vi "7Decembre2016.vi"() -> ()   [LabVIEW 2014]
panel:
  out "Pattern BAB":string[](array[string])
  out "Pattern ABA":string[](array[string])
  out "SLS Support":i16
  out "ATS Support":i16
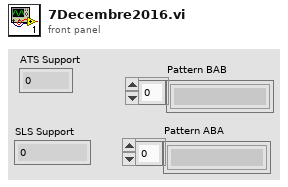
[diagram p1: front panel]
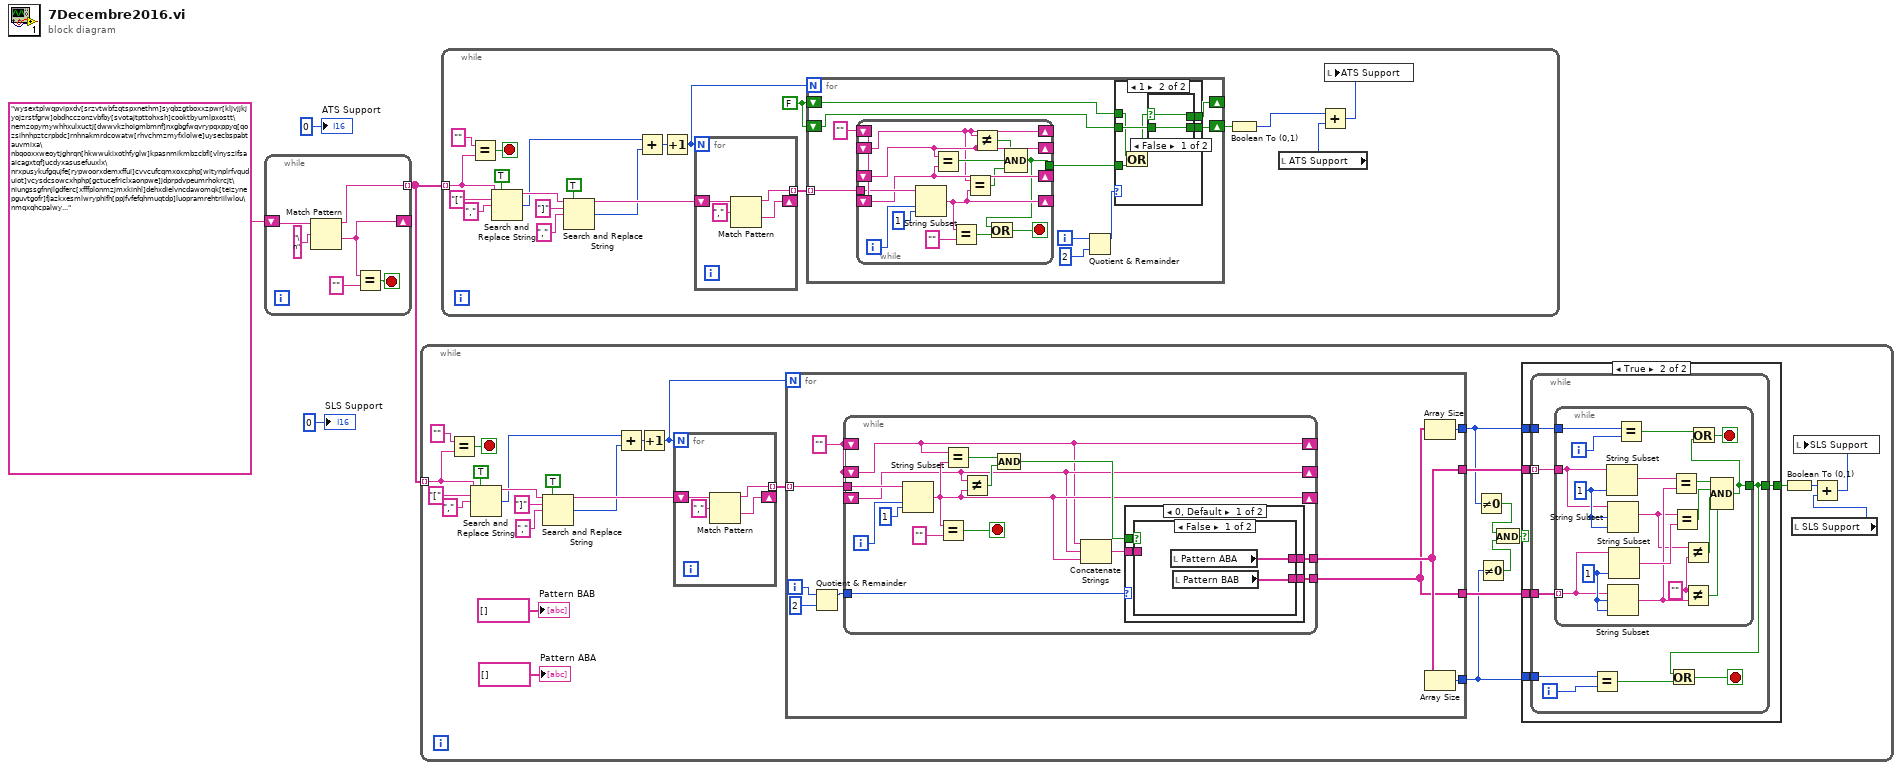
[diagram p0: block diagram]
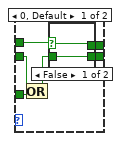
[diagram p2: hidden frame]
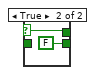
[diagram p3: hidden frame]
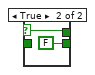
[diagram p4: hidden frame]
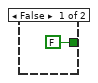
[diagram p5: hidden frame]
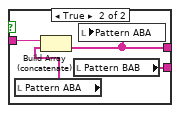
[diagram p6: hidden frame]
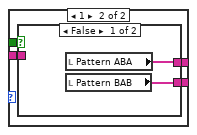
[diagram p7: hidden frame]
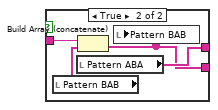
[diagram p8: hidden frame]
diagram:
  n1 = while {
    shift-right: [w7] -> _
    shift-left: "wysextplwqpvipxdv[srzvtwbfzqtspxnethm]syqbzgtboxxzpwr[kljvjjkjyojzrstfgrw]obdhcczonzvbfby[svotajtpttohxsh]cooktbyumlpxostt\nemzopymywhhxulxuctj[dwwvkzhoigmbmnf]nxgbgfwqvrypqxppyq[qozsihnhpztcrpbdc]rnhnakmrdcowatw[rhvchmzmyfxlolwe]uysecbspabtauvmixa\nbqooxxweoytjghrqn[hkwwukixothfyglw]kpasnmikmbzcbfi[vlnyszifsaaicagxtqf]ucdyxasusefuuxlx\nrxpusykufgqujfe[rypwoorxdemxffui]cvvcufcqmxoxcphp[witynplrfvquduiot]vcysdcsowcxhphp[gctucefriclxaonpwe]jdprpdvpeumrhokrcjt\niungssgfnnjlgdferc[xfffplonmzjmxkinhl]dehxdielvncdawomqk[teizynepguvtgofr]fjazkxesmlwryphifh[ppjfvfefqhmuqtdp]luopramrehtriilwlou\nmqxqhcpalwycdxw[fkwhjscfmgywhtvdb]khadwvhkxygtxqx\nihekzgbwpjxgbau[eqpvqxncntbtsqn]mbtbcujdkbrhxdu\nizikobnovmjzngo[ombcpcvshnedtndu]lnnmdkuapgnxpgyxcmg[bgnxdzmiolfvvaizu]tcvnrfufuvhgmlxcm\nyhrowrreplrrsbupeor[nchtznfzbzwnogh]rynudxihckzattbz[dshxeaqusdlhydtm]rvqzuffgqtysfzxp\nunfjgussbjxzlhopoqg[ppdnqkiuooukdmbqlo]flfiieiitmettblfln\nhgtbgxarmgbxqrhghxb[hflfvoetxfisqsj]syhkugztqkywetyhad[fmptjuaqittvvyooda]cjkxbnylglnlfleelzu\nnpxhwtitqnddkwg[gmzggwnvygsroeaadtc]gudnfyefqbbgyspdxjw[ilthbdqubqnveowv]xitfldhfjyjsomygjg[knmrlvoiqyytigytlum]dlfpsnyzmhkmeevfwsf\nwjzwftiuixvwyzmgoe[jbfghrqhyywwhlu]wcijbojvlgjjdtowzpv[lgfvxfdusgxddsppbxb]pagicuiuerzeydww[wlpjklgzyilrifonz]gdicckmxibtwwoesaxf\neilrieezaciolhnhrc[hcisnfomqiiaculxfv]bfyxxhgrakqogthzft\nxijomgpzpilomlpy[sfgwaovcybyhoogrxsv]ufncwrahejwlhyvz\nnojlhdpfkjbhahgqo[lqrkjabuijutlcbq]caszlkvkofxjyqzsttc[isqicyomykudneq]izuzehgtmwnnvfrlrja\nqwfvuzrogqzvnhyqdv[qhnjhafmrtghosbmskc]msmwswtgzlpmtmzne[kovzhefjqtqadhj]myqisirynftmtzvxvvz\nfrfongnaecavmrhj[uuptwvcqozxnglsd]kwpovfwuhmqjkog[phtrgysxaltvbohmv]abhuahonmbhsmfglltm\nwdqcwcbtpexduecepe[zwrcpctlwglgfpappb]zdadimzdcpxhxwde[yquulvwgyyzwcfsvkdt]thgziwclyxxfyjpbpc[ypkjfrfkxlkavboh]hxylcecamgezuoljh\nyqxkafpkuuxfafe[zehlwtvpprtiqbl]qswqigaeaneovxm[bqoieihtxarwyrqegb]yzdopgmqklqaizxjm[jhrsftklywefyevvha]xuvydwcntczjvuduj\njudhawjtmpsxfocai[qghshlgvbitxevt]xehceioknrewezihnb[jvrzemakemtgmqiqmvj]wewpjflvqmottqx\nuhokpvanmvdobqitn[eosarcmqnukoczgz]rmoowtgbbyimkptlxdu[rqhewmnpypqpyosgehz]nqdwglwscsizxey\nsbnojmynueuyyutr[oonxqrbbjxwvwafad]krqlneuehyrghmkrq[khsckkfwowubtglegu]xweufrmlufamzbcedk\nnmgjmbwyrvcbthw[ogtvotifzugvvrsfe]jucqbvfqclkuxzumoed\nuaokpcytcrfpitfursj[lweyfahryjfprulw]dsdutsxdtugaced\nahshwqihivxlgsj[ldnmuwbrmoxtypqluyz]intafryfavcnotgxu[xjggdyvoarfajgp]zhfgnytzjhuyheqdy[yeynlfshsyrhjxrzguu]onvyhjfwooikmmqzwgc\ndjkgxfnfojgjpxec[ngwqajfbywoxlbm]oqdqigzeqadgqjt[tvojayieruftbjokeeq]gxwtruomnhorqqrpzt[bxppvnbiwhkhdka]rhpffqekyrcgwqmoi\naasbwiocfkaahrjwerr[dvlemehlhfzxnzymqn]okxibfrlswfvmreuf\nrwcjoknjvyufkrp[hsqrwhdlwrtlthp]ijezyezjdrhzgltliq\nazawpddzkqbosmltyxt[zoaaqnowmmwkmfkq]lgusvzwnimvgagupkt[scbjhqdftzssbvnvff]coiaslgcrwvyioxx[jouvwdiwvbsembzf]popmlnhjkoaeahcny\nsnucfdhspcbcsgjnmcc[qbicureolmbzhsy]cuabqhzbcbkezsumkq[cnggwqizurflommitua]ajtxxkqwqynnwroi\nbsxzwpiauwlqelesq[uqfdggoirtlucvedpl]asacxftfqfswiapmj[nqohanbbzodfgkxihtt]lhshhkgjvjkumja\nbeewgulkwnmwxenstrz[vybrrqhcdpkhfnshccv]xdfvqzdslwosulzatc[kuknmynmjntvtyduwlh]trfvychdobyghnrxrfy\noxrwmqpvxntdkohmxb[wugyubwxumwnxlk]jidpzvtbomuymyf\npqzbwlnmvtytsfre[pmtmcnxkylmqaeb]alfdaofnqpohulpmfoj\nqopdwichdepaubxxeu[ifjozmlqttahyugyt]mfmlwxifscsnuom[kiyjlqqxunsxfmht]icofrxpdpsktwiifyb[hetijegmockkyjhhc]aarioqngqmdpkti\nklumchkwczxuuekdb[nlalmjunselydybqxdj]alagfcxocldfyzdnzd[abfnqrgrxbscagj]cohrecgrcaxljkz\ndjydzyiyydcneoubp[gorqzujuwkjsqhelfrp]pvtvbhztirfzmwcopfv[wfjumxbfvvgvzltlcf]ergdkkakrtfzcxmqcc[vwnkrxhayzbvbauvn]yjoqveipzibbmjq\nqbdruhoywfjhaljfkoy[tznfejprrnzrrewdx]jziputgqfcqtbhvhlnw[ikahxtlheeunzrdq]tmoanjmpioumvpcu[tnmcvxkewovprxgzd]trnmnhdvtsisiujqjk\nllojixxpxtvcwxaxp[rurmhymwuztchngs]weaefxdkjmofeydvfy[hmbracjdcwxfeva]jkiybiomykfexjlyg[pgrlrqgoxqqtoio]rdynpcndtqarmkagbw\nkislmybuoblnpsc[dvsrnwlsvxxmzuu]jakczftcvijbavhjgb[osdyplcgliragfnpezx]kihkywmwgbkjtgxn[tdsgdadcvcaxfrbur]lzyjmrjqztybfdmm\norfngwdzlrucbkbqd[ibvlkwlnnzwkhnoad]brstantuaxwkibofh\nvuumejklanuomqqdbva[mwjzrpargsphzkkhaaz]lkkewmbrvuczyyu[ebpoqgoifelelzzhd]biflvclnnimuojihdmn[llrnjdgzagktjrys]edtbmzmcbthpixhwwyz\nftaciyszakisxhzjhbo[khfshezpopvjaki]pdnnsqmgpgatvubllrr[ovjrouomglbpgvtya]ifwcvhascqptbvbums[cfpimraygtnuimiup]zeykmilehidtlstjux\nnzgbxxiimmzsvhe[ixypsgextxvdckbjelq]jpklrvkhgzprfrsv\nmpdlsziccgzmvorvm[vhxbfkwfwbxqbvxp]zbsxgodzhgmrhrprpu[pvawdsvqybgdncgxido]zuhyfbmmhzegohu\nrdkteyoeleyhxdlfa[nrrzftpiqatsnnnsd]qwelhxwbpuwjmrjxmgq\nvpdhtcgjpkrqmrt[gozqldncggxpvou]zedtarenbxskusqk[mwpmzpwraryuqqmdhrd]eoculislafmbqzy[okpddsvrtyrkbjtihhb]dvuadhnaxkfewhnksl\nivjfulhqfbdqiprzbbe[ezhkhqxcviwxbwmlnbb]ttekmmdrphuteslzwcj[iocuduwexawydww]qmrfnnedqtqezclpuq\ntksplumjkpsjjorux[dpffmbayilzuszc]rsiowigabmredkfv[aurieaasmsrxufpo]lbwvhcrjfgomkff\nuwuobjzxkgeugrivc[biktdwykzondbwiko]nnrtnqzhdhdwzkau\ncjjawanjvbxvmvdmtu[kubvvkuoynaawzowphv]ssijoohfemyhrde\nqlykdpnioshrexuw[tjwoswemjxylnqupgv]ymovhecbliuuzhjwu[ghxibaaourtzzogrynv]hmlndovkousrtbomlnz[nzkdpmqrqovnvskh]vdvntntzrqrhvcaxdov\ntdhrefyrccgkdquxz[jqeprpsvvkmmldlwyq]lwhnimtgegsziejeh[gyefzqbmfnhzgtq]fmbcvbjtsriuicde[sbkkbqwzlluccpa]nwxmuolcbhtwcllmz\ncakfzlwlaxgrzjpgck[toihlzbehdzesbt]azrsizelgzczqxwejb[ypecquckfavmixeyjgr]njiyddhuwlwogbnpt\njadaohixgxzjcopk[wopcnehanaabtklxnez]jgvumwvmixxxwaolxb[lrhmslkbmylyvlkx]tatmsbtlbcutcydlrf\ngelrpwfiyiszejt[skpclwjhzgwvfbbd]ibwzelwwhvudmvoe[gpdveubkzkkxvtjn]khmkjslnkdlmefcx[fcwhuyiyvnjgfcva]qjcfuqxwmkyvvzuj\npbejigkioxtdjjzbl[uihultqxejdyegacm]fitsnuitopdzrxskz[shbzwyodcotpvoixoz]qrhuyetkmnnljfqt\nyohbaryhrhuobkf[fmfsylvacrgvpnlqdb]iucbpagpbziaqae[lfcjrlbgxiytord]mhjlzecyrqcpbxsaq\nvguohtnahunrvrfv[lwbganvrrgnasnkqjz]yuoncrmethwiglfiy\npljibizefgbrfauieem[yadmbpkftrtwjrize]fuzpxdpomsdxfocc[lvoahklovaxtucrpwhj]newpgoizivpqkpo[uloztzclhwixtcjhyon]qyzzqoyirejavchy\nplinqqpqghkeuipqppp[rndecheohrsftgvku]ogsyvyxuetmdomwdmx[lumcfskwppjacuddm]uptsydogwyqaupdft\newvtreckmjqvkvwgtz[leisttvtmrxnzjv]bfzzponjsjmepqjfs[knbonuuuhvtvteiov]vaejlijsnrpqppo[hvwwdxernqcxtxe]ssznbkhfmchmjjiahkk\nrrofpphpfkeeqlxcev[ierkxtuduxxxbilmg]vmipzdomogxwiazla\nuqmllifxqxwcskoj[lwrjkmxgwxwvkqrsajx]wpbkbsohlaeskzbv[boyvlwxpqpppcknocv]pgsvgtugmxmoexrvpkk\nzupunwchccxqggie[sdcdhzciymhppyaaaib]izbizcvzvbcnofmqt[lvvxmcmydxruvudsar]gnspfiadqokusllygyw[wbcpnuppeugrqobtnu]mcvfhylypayxquurcv\nngscsmmvttxjxoaniu[wsfnnfnkwmjxjql]ijtqswaevexzcmgime\nhkmykmrremccqxvfdps[izfaeewfadfhuwwd]yffzgiqtmayebphb\nznzxjrdnxhfydrhr[kwafvmygvlylite]hmskvvpqyoblrygj\ngkxzweijinwxyajq[jzljdfxlossksqa]octzjmrvxkumtpn[jypbqguwpybykguwn]ngriygtjydfznsf[cpwtojpifkhwtfknjsg]zahxvqxjtoutvvsphh\nkmvndjahzayidho[fitbtgfncjvmbyrbvnf]fodwrbklqhxpsrqwh[ccwvgmocbtbqvwzu]uuidhylekzxzvmce[qbhkjfhnczasecv]ctsfirxwjfvrmayoeb\noktwbkikybfwojcweal[pnhqkawxmfxggabhgpa]kdjghdalrpgsdhqj[bxjcqdytenfjirvb]odnhihekqyskaoedyor[pqsixozypkjdnnntbng]negjtmkqfykrjgewt\nhriyrcurqmacydyay[gfblxaovvngyesfa]tmftedgxujvmjze[knivpbneiuxdsowcxdt]zzncnfcouzoppog\nedabqgdgbyjqkzjvzhr[rdejmmymhnvfrqvf]zknrxaqjohlncvwc[lcpuoqnkvwgjycfm]ohuebodqzydltckrsb\nrxcyawcfxcjtdshxg[zvggbsrobekoxidyx]zdpvqowndwgdubbhst\nqngajrgvzuafovkr[kracjvrryquumqerjev]mqddkdpqmfgexahczm[psmbzonkrrtlqdpgqci]obiynfssuwhprevmzm\ndihkldbnjicztjfrvga[qtlevmacqkefjomc]opjaojctoraohocxaca[ojldoulpocpcpexnyx]qnouppkcuggjmod[oeiywfzmbjrhtxz]mvhoarchbrpndgwhxga\nqyncschbsnqwgvfu[cscsfdcfbfqiwgwqi]pqzbontuospgycwzqn\nlwvovybfksidtajq[vrtqmrxzouplnjogzk]gailtfjtszlxzwhbs[bgqzyhgudphwgufmg]levofhjnxjqhkcy[wbffnapyutukiavenm]olkwwlrbbobqudwvnur\nyeqiptxuczuxzeatp[upzutosphyfhuho]jehejxjvfpqeifogn[odhltqvdcwwmshl]coezfdamogigspon[syppfhysfwfkisltwr]ihkaelrbcelykby\nnmciqyaovpdwzldwt[zoaowvxkrpfuwnyepcb]yhqlmmrxxvguuajawb[rmilfmqzokaeabc]yhmswnsiyrepbudi\npifzooabiqmuicfqi[tvaqijdwxsbamxzg]zncutzbfmraagej\njpgkrbovswsjnbcj[bjybzimnzszdkqj]mvwmgdithrxecpselt[kghbhnctqnhhxxhdro]drttsuyvtuuygdtfaf[zohajxyfyjnqrigq]gadarjzfafqxsjxk\nwivyofwdmipecdxuqu[trccnlbsvfbagstm]xajuejldffxzxfygsg\nqsuxdmtfgpmlgkh[gisuuzaglpmbmydtt]qzyfvzryxepjmnr[mgsjrbmtxxzkadomelm]fqzjahepxspwkwpwd\npncauthrouncvjkrik[cyiovjnoesdgpeyjpvd]ajhonypsbifeghxi[wmudcxwbewumjbegnh]qetzbstgmzfruzxqln\nqmkcddrhexvtylukq[nwrryzbnjnhvvgm]edxlyprwzzhgfmhz\niuonniejtavofqdqsln[ynjrsfsqrdsgydhpdvh]xvqtjledtcgkjkealws\nfhbxdtddlvkjrmjyae[nwwjmjvxtabdwdezfdy]iwnsmstiulolahbxka[lqrxlwifzndbeid]jilfjomwrbjeniwybv\niptzrdexpfzabqcqkm[kvaxgarrbrobtmu]fqaedifschjkoepn[widcirixuswhcvcqywp]kpkxphryiwwnkmb\nzbeoanntetxhvigve[fhwvhghpujcldib]ncrcyvevibooqesy[ougjirkquasabeqad]ydufeicmimcwgtbg\njaocnzcwgxknexaf[cqykwbyvxtcwnurw]udxjnumyhelfogapi\nsduqgjoijyfrcnfencj[uxuiwklsiuqwjjrzcfn]epnvqcjspwopyffl[mwghrhtfclodjan]ghamugnhrrzjwmnc\nwoygyvtrlmjzaeteuj[vvvfohavzuuzyzgu]xjjcxhosambmkixiie[lqholbwbktlvdljmapw]diufpkdnjmjnmyc[ehjexwagbmezmpj]czhwzecixzxfykaiafj\nnkijgkhyilzqvtgj[llydwhyhnhpcracxxd]zgtsspcwpyujndbxvp\nnawnrsgxqpctinyek[ieguugfkwujnymij]rfmqypeekkdsttdw[rfuanabgfjgctueaaqo]vranbomhrynvjyywmh[zjncmschlfmkvhd]gfeoftxsawcgrzvrlx\njgazasxbickiiiz[duuskjowanfmieegl]cwgdwtrzpbfemqitbhb\nlahkgoaoeofjlocsei[bwxyguvgmenwnpwlp]jigdlgdjptkimoyipa[zlcyjbqohvmlxgxp]bmovqedgchicusqzq\njhkxinkbwhpddvjzgod[fypyyhptvewejlbwdmx]teagznqhjydanxxi[wkppnjsyzhwshtpo]piaqxcwqolwklwzsfkg\nsjedigezzdkqlxlcnr[xanehtpradlngiob]uonmjrieoycpthh[wnsqwfubwxkqhlflzv]smrebfwpnhskzlknva[pylbyttmhyggonlk]dwqkzjmatybpmgeb\nktfcuvnwueamlwvgwmq[czcgevditrtvddgfh]djmmelqewdnzrlqliz[fkpieaipgyxnkmjp]rdpkfzvqpfpvczv\ntixjemagwmynkihelk[bnwfmkugsnivgdmvskc]nlasqrjqrlorszi[kbatouwdhejxchpdhd]etmbkytyrpnrpgqvel[xahfkfjmsqjycaq]mispsimhcckrhqvek\nabudxncgozbrbnx[fllpjgocynbuyawgs]hiphrvpugpfnnppn[jhmlgjsufflkdgw]ldmdclrkorzjtbjqcrn\naljahmvdrraiavzv[tevjntkppnjqwovvuuh]ozmgagxzixxyzuy[zgefziawisowuyqra]nrqmsbwgqbfrxqvzu[zvzglmnjmjpmditiodb]odzbozesvocemfyis\nzgdukwtswaosbrossf[ugdnezayjnbjuhpeh]knkvomcsgfptssifni[votpmaaohcyofgdz]skbvfugaaxutcmrmsc\nywiphurgqcvybiakgok[cscyksufsduegggw]rtvvvokrvwmwsvmk[oqvdxhoqfsfdwwm]sbzajtnbxzkyiwrj\nnxrvrsbjsrysysvftoo[qowwnvlezexjyynm]nknzluizyzjpbzpevb[adkqviapkjbmknchtb]xsgtthuifmsqidyh\nejrplkjjbnjjouesaph[bdtybzkfyictcjuagr]ivtcttyunertnzgmpqv[roikukeznmtkqomqbk]lsxzsjrnsrdlxevj\nqgcebktqtyjjwsav[naozjsnqufkkgkp]evimphuulhzflub[weanrdvlsmmypnh]rojhwlyxtszxsjiuai\nzludmyuqlfpefvxcm[hejpyhwaqdndtwslan]ldtxkxxtegoqpntsnwg[olhtlkpvkdgkkxkisp]hursraavetjgloks\nrosuljoqspxeovaqr[ocjdnpuzmwioylt]txylrlsndrifxiuxuyg[jnubpcjyfzhiwul]pdtcjcrkpmzlayzcty[gasynfnouxnvrplkym]naxwpqsxlsbvyuavty\noxbyqbqmpckkdpfjtr[ggnmfcjtyfspqrqkg]tzapjijawrabozckadp[varichgjrivmseddxv]admqmnzxzqcbapdquwd\njvhvqxvhqfxnjzmv[hwfwxvwhxorzqizc]rpjpwggqxqkaznkuqn\nyrsucbqcfaukancrr[nabtowgijsnzryuvbiv]sfpffzxrftnrkjx[qfyfsbkyhetcedf]xdykjbymrqgheanxx[oxchcwrkbqvvfeyi]bztjlknshikocxztjm\niniqqqqprdeznwhr[arooglolfjgprfrbhbm]sczcmpftuhbaagwgedq[yutgzaqyxntjxoglmb]vswbhlspwfulowkif\nbjcjrdzwhmssgoinrcj[jobrpyapaxkasve]hzacshssrxkdtrlqhr[yygotqrmvhiqjrja]ljwfwudymzkpczysknf\nlrnqnaxtavkhwfebb[vwyqnqkveujnlzv]coizhrfmviizxgz[zklqinvtnwtajyjx]nxvpznyebozrosfgh\nccjjszgrbozbpopagns[abiuzirqfzactus]eemrbqrkhhppvan\nxeaifcibybamzzzic[ymvsqllvremyfify]ftgmrkhzswdpbmukcdv[fbyevcnnwtnodgxy]slfjznnldyuvair\najmeryqwfhniqenmi[bdzlgljpkkgsvpjcy]hqzxecqxmneterlqizz[pzrbbprbhujzpcxhjmh]lvrckyomhvidbiapikk[cyyapugbrwlubpmn]toodggarcneobyz\nlehpdvqjccdfpzpo[ssunfejvfxwzlzqy]dvhwfrwiipveqpb\nijmthhifxtkoubt[jcgoxkntpnxkmdp]rzsfekfmamzddgm[szvzrwthulqzcorhnk]lmgsxsjjcagkaysalnj\nqmfgzmmoylbruqxoh[uoyinkzbglorxud]frtffuhkchkrwbxfx[urlwigeirzobvhir]pqrqujuwxueommaj\ntzjhaiqumjufkzcvphi[lhfohqxxuoqybomckm]qjhpjkjljzekboyc[gvzfehzyrfaarfklybg]fhurcpaukztwesz[lhvnhfgpmunjukye]mdzcvgeehmchcqe\ncbyyjbdwzgdhveyw[ockkdpwglixvbom]ozezplbkvaulagw[vmzfmqxplwaqjrf]upytqbnzjrclzfvti[hztxfkqwcuypqyhsfa]sfwcfhrnccesyncbg\nzaclpaavkxbpjxse[dmuzswkobdcfmrejhaj]eqdwvpiphijpwrvg\nyvectfptgdasqxi[rmpaospaiqhwpjwdru]ollajqbxmfnqmqrdce[jqixwgznolbepskpm]pmyfsrnbdcqdrhplko[pzblovbmbnbwjzsxrk]hgwpjhgshxoozdu\ngpnplfnpnmdlhehgazx[gkgcsjdcfnxytzp]wamlpixcrqvbtseb[ijaxccauotewzkgu]usgmgqmezufmgqjslbu\njgtqghpjnbjkmajymfw[isxpkhlvtuyqpscvm]czbrsyeqmjnksov\nfjsepwfaxbbsdxlcz[efiljmecvcsybpj]fsvcvvewoepnvqz\nnxzdtgomsakdhwefrn[cobjsrlxnkxvmhk]wkfnuypvsigzcnswufj[ttmtjfkbnhmmdebtr]ffumzvnvgitjccgz[offnegtizuxhpqmic]lbhljegbjmldqbzryis\ngnnsvlcqoatssjuijb[eaodophfeufuvdodj]jplhbuvzqfgvrqbuy[ezxxqanlgnxdkohew]vsukbzhjshwmmqdkzdh\nshfhzsmqdeibrwgyr[slyyksjeywcnuaocadr]kdwnsokrwkajgnwi[zsfujtkhknplyieg]kijuvumdqvjyjpbhl[qyrlzloooajylfrsfk]gwqdkfpitiitrednt\nzhmwbilhpywvxrza[tgnybotdqixzolvn]ptxzyjbayyevmcqua[hcmgjpycosutmqbtkf]tboiprpyhwgjceu\nejuvrirctrlirihunm[nfjigabdmqnkfoauuyg]rfwcumqndfgotyx\ncxkwlruaswigkrtxxch[fjsovwltjonhegm]zkfawxnzxlkaqawq[rgfftbipxlmelfnpf]qhhslyyiluvowxz[bgxutaxmhxyxxdob]hzthuaqpiyeomlgqqcn\nqyzwezoszvwrwiilglw[opryawlpulfkpkmuave]taxeqyunnihulfp[vzxzosekvamoofva]bbtonpohbgdwfmt[xwzkmwrwruatcdqrj]enrapbeqoxrufgp\nlowqonzaekybouni[uehkpbaxwfixuwlj]ionorsihznoszwzyq[cnatlobscugfpvpbw]lnsmgieepzvmhvbz[lsjebmtctttclkxqok]jwevnfmcrtmgjyniiuf\nltxumfyzdinfqrlf[jyiwmlpqkbnbgmu]bnicegkghtwivvyozea[qhgoiugrookfmdsln]fpokyqsoknuahpmutnm[smzqellevlxgdbbet]vsadiuyglyyuccgkrz\nfvhanaukvcjdkhsydnz[pbjsoundyybhvaqglj]esjjvkdvjmgmlox\nhcckhzdfmmvnsmuzjg[uuajvdzksgilxpjmnv]opbmjvfljnqzxkql[pgdelzddxqrfdoqnit]hqrrfnwrokufpybg\novtjlczqesucgox[kiqphngcbakoelqncyi]jhrwrpwdjxbhnqp[kqvqdyokyuxulxidc]qumskxudarjyagegy\nmxrxpfkynragapzrmdv[rdhsbrxgeywqbqh]rpoerdiwdisciarhl\nejbdfeqrdsrijztlibc[beglofnxveiorftulay]jslqibpnunabgqmi\nuplsbqledimexhzwnkk[sfreaeitecravsu]exfxqlrumxaeasi\ngicahlhkuxbhppe[cypyeqpzkrggfqrielv]pkuwwtbezndgtqhbz[ojnnxanlkamvmpqfj]eozgnkxtbtyecuhs\njtzwiyeueztuiwysyv[awibgssyyssrnuxrvuw]mmyvqfgaaraahzzen[rhscfvdrvagricw]qsqbnurcszgekmp\ndxkeveuauhblqnq[oksqvawybtejxmdw]jrbwmyxdggncxitwcms[fvhnmupxnynxmprs]odbifiqqxskxaqn[xwdwagplcltcepjmtf]zsfevibkmzwtzoq\nkflcnlkdujmtiug[rwydvjaazfgmfcn]qolbbuxzxhoizfqcwn[tprjkbylcrlvmbggae]pjwhgcmgxzhxbxdceme\ndonbjfkqtygixfpaa[lhfcyuzcmsgixjbr]njvgmbwgzimrtpdmvf[eonodblqfpgtmex]rkakjzfmuyeajvhs[lmgtvenasnqbyby]jdbxoeqnwoednoncq\nlaiyueskjnlltkwm[lzrgjwrjchpmnais]pqltpskalrwtmtagvm[luctnpiuqvulmtmw]awlqbuutunlbpusn[hdetxhrtzhkyfktmfn]qpmezabxzrtquidbjc\nhritvdzjxipitctgoex[jtbjcyaysbefjme]ebbcyqglydfhqjfa[uwuwqhwanfydpxqk]enevryjyzduawrfc\naxxprqpxpifqnwte[qwkkhbywyixngun]ufwcbmerbqiblbdmn[mguzyerbfhpqnybh]gscgmmckgfxvvwgxxm[gfjzckcxdowpwmhmg]hjblyfatzhxjyvlccb\nqzzkrqfnnzvgfmrpjr[sktcrqxcctcduir]vmhsrsedrxpnrugm\nmpxgzowtjabzwfcbeg[olgfqepvinejmstbrj]fnqxcfzuxojvkscyk[pxbyuusrrbjwrygkxm]wiojjquwvhineivnkys\nvqcisychxuswbqlzdkj[jetvpggxtqqguuh]tyllnzfyfphoudijzj[xlnznxybxscqjktjn]oysyrlqascsqbclsb[rzhxpwwrjwakoldm]mrwzibdjlhsdsbew\nrttdskfweqmkjolrgsd[gmdwcimmgetwiprem]wkyklvpjyhpzvmsh[zftyxsrvhnioomw]mrvoyvyyrlguwedz[xyrajtcatyabfqigup]srjmohoxwdybksfv\nxzeexlrzdznmhbph[vobtfjuyowqppxw]mjxwhgwveozusndvi[jthhtubbkbmdiepfh]gtedeqwesiwzlrfny[tppxuofhnwwkbkysg]aygwlnvczaarhfgkw\nzxirxtzlqkptwqd[vwdzostlmrbjclfj]aluxqfcdbjwbeerhr[nsjcafnammlxjafrzaa]kipaqywrtrpkbcdtnyi\nvovbpdgnfhmeuadh[bcgvleartfaspvvjjz]ajyzrbirtimuifvs[lykguucpvkxuupcbims]qplsipqneiycefb\nalqzdecagmvodcigcd[atmngaijkfehfbc]cprsiaclouvtbpaab[lfrxlrzuuooqdtfirbj]olcjwtrkndcvykp[lelvgglysdxycvk]uyakjndqzxtzmxs\nsyngsortxjqcdwcz[qkiseyvolwhibxdg]ucuxqdozkfgaxqwovk[eqeessuwvcayhpc]wkhzcbkxgakgxnmho\nbhtxesznfkwqbodb[ptpuhbdsvbcjpmnsl]oohvgktjsjwxqgyxov\nudnbbnkojrdevgujkg[cramyjeuckywtuw]qtldussgogyblkm[yuwacyafnikvgbibmwn]xvsgxmywenrmhdctxg\nuzqtkzkmmeuttwyklv[rgnrxkbavqabukxvnp]whhgpmwocfmplba\nkvbjvjxyqiqitikvm[vkzunkivwcpvxng]totvodotoqiqokouz[luzygityrnpuiih]eadddxqveeuujmvnek[nyxhwlkatungkgm]bdhobvhktlnfpjelr\ninmnseeoqimzjwzhltk[ntwlsdvvybtdoqciu]jaurhomtnyudxxmslj[wqygsctddywlbxg]apsdlaftsghmhtj\npxieimaprtbntgvm[xuvwwsinhwjjapu]taeomoijctvzyeijfr[gitzztxejfefzvepf]udobxonjlqagrkpaehc[fkqjhfjicleroxp]hxpzoklhbgtngtagcz\nlqmoxvnknpqzcgs[zktsmqcgzqjponj]wfhhzvqiqkxfwrrw[actbxtcdlogatfkprc]tvzphmtxfrptzlopv\nczdnqiwqhighizbmivy[tptpsvsahslbsovazkk]ycppvkqvuggebgxibe[qutumfpnpzjkgqyfkok]ixywxvmvliftixfie[qipgniycxomhgmwje]vnhxbcnofkcnzep\nigvdicnzsefxlgk[dzppkxdievabwyh]fvyywjzcyfcqahv\nbjzwblslduiolbezybz[flvsgshhznvzmrxo]lottitaizuksqfihn[kgsgzawzjlqjsep]ihadewtrfpsudggga[oecgswhnbhslysd]flpdpxndzacxeskzmn\nsyxfjuakhrnntipfpb[xmntswflflstndkv]lityfpfignnxsyirja\nunggjaqgvzrckyqx[llllagrmuioghea]qafuiwqpxcljhvf[tevtmuvcyqqrzvrduc]kqnaadyfxfyyzjuco\ncpjvjnocqphsagdizq[rzfbvtnodwqrqprvqh]rnlzshtjhrevjgdu[lbozqegfwoaikxbnt]cqmzymvkummuzjfx[vtknqltevighwfdnjv]djhfeemiljlvkgqkpp\nadbbbgxmiqomckxesb[dmwxvrammletdiim]eiozjsockohijbiinia[zyjjubdniurametk]ajivyylxbhvkktrzdg[byxiykqfbvpfdzdv]zborzsvqimrhyoyhevj\nfrshflyhzegyezg[xxaoqtzxuqbamukfxed]klyullmlailfvcz[boefzsdpblwpbna]dbnxivwobykcfwogv\nxxycwortiwhndrvlr[mspdwmhyqdwtctlyek]qnzfcwwvvlfsael\nfnekkofpuwhttni[mlwvhzrwfdtfnvof]gtlyjqokjymvtkiqdl[gdjobagxsuhudnoi]jgcgyusdyyocqwwtatk[rjujihcuqgdpcbdnkco]iewvagokrzdhhhskv\ndfadfbjefyinccgzt[gzoojtdlvqysetfihg]nlsriqansooflahzhoa[vlzwtzgipbaxudxg]htykxxpfmhigbdqsu[pzipnakgdfpajkbqowq]zrwedqiuobogirulfwm\nwevlduhhsouwlqxdcfc[bxcvjwespxdkulgun]hfuhwpzgdgqsujeex\nzweayhrezaoqibgvc[sosownrvumzvynfpvr]lzubqqqepwraqqdxxy[bniazltbdanpnjjjuox]tulybfbbzeiyidrv[zbebbcdzpcvegcms]jdfofmnlgwrnvann\ngkmbgzvludgmjgnrkck[ijywdgxetrginhtaa]yiokddkvhxebbuyrwoy[erhxxldeegvsebr]ujqickibpbjpizhbjw[mtzvltxionpxygo]mbcgbublhkajfdfvf\nddjzsqkoizakmeifr[sigtlzmyyrflvjowj]dyqyfvpkhdulwuj\njivforicorwbkmccpgj[oviyldmrjjzbojbs]wpztdiwcdrwttmfdw[jgylosmbgxlrogsa]htkvwsfczzoascpunqr[uemtqxhcvvphnvktio]xkghvnicljrlndjtsv\nzkzjccnvukaraob[asytykcstvxtkvermx]lqgjlittfqpyxcq[dwyrqfxmwryvxjzr]edufjnmxhzxokjgphk[ucthvgtgfpzxikmnjv]yqumujliwpjujnymcen\nbhbndmsnnbhspzjby[llodpdecwrlspsbhbhm]zqulqmxwcerescalp\nozkoqhvatxmivox[qffeloluwcgsimvcrnu]pweywrdkmtqjiflvcm\nrznstgdzevfsthcc[jpgjzgeibmumtatu]asgwjccfkwzaigwp[soegoylmysqcequdsw]pennknxcwwasonjz\nafniplpdesiwqvdioov[xfkwuijxjgtqbhqow]idmgzrcmwzmrfbsubkz[mjwyiznfpjztbfervj]cythmqghdkjcfrt[ekhpwckuwduoexycc]htaeivvotvlstvsrpj\ngecbcvpiswzjjeiriav[ivbfdesbkamvngogjb]xphdszgbcburesbfi\nuldzgctwccgqdbxrmpo[guiftcqomdqlqua]dmxluytucnlndazic[mhmdapmemlrwmvdzwkn]oqyvwmhlabcwxpzioz\nmganrfqbsckpjsnvlh[vlwmfxhxlnnpsghrhmr]eqyrkxjcwpkahqpxeqr\nwpbzefalgkbnrke[qruzjqtrkbzsvfgwz]vahtniazgsicquatrg[zzslttuxbwolldy]cuejnzjsuwgkobp[yspyowiamjpzcaqwb]vhakhmjrncjoroe\nycxznczxbzrprsiw[oggkqxyiyvsrmxck]asjjivqayantzzfysr\newbllymppqrdnaeni[qkytupytcgsftpprv]jfepwibznfbypfnf[lrparpwtkrzlxwep]vdsywhvslycyohef[lxhwibvmyypfrkdsley]kookbjfsapqphmywuu\ncfpbgrwdsnrgddzzh[vbqzujunswprxyxnk]efqzsevzxurynhnm[cyctdnsmqdssnmzyrg]vvswrmqzxnrbkhunu[homwjhndwctdbecwh]cdvggafdchgeuqy\nlihwrhvzkhbrgct[hmwzxlaycaimxchybqf]ruvcpltuinwybvv[xjbzxcihznlkorih]zxnxeqobqveujyrdnur[ijhueqaqprdlrdcjsh]blwxhcuajnskuntgo\niroxkwgrjpzdodvmohd[wexdltrhssaqwqnh]ynvmdpomrekdsfrjccp\ngfusgnroizvfwwcsc[jgvlrznerrnjretc]dcbnruamgkyrowpglv[tbusonvwwycqtfk]oqngfriboradzof[yosalcuxlovxpjnoss]teunwgykswgulguic\nbsjpzlhhqvnghwnp[gakhkxegeohljlwz]hfhculyhgdwcflbdt\nataqyejfhrpvpagptx[ufqdptheyevtxqjuqsm]tekvtwjvapcyamluzbn[xxktujajfnprffsvfkc]espinhantulzwpqug[pamkrynxvlrwccp]bgzabgrubbhhwwanvf\nqkyfobviahzasbi[dqhxzkbapqmrubogqg]aenfdyclijdpkeqzc[fbetcpbytjywomh]mqzvwjmgiexjfehor[ntwcsnflvlaxmfqh]uvubufoducqwacwio\nzvygygjncwkyceve[knrtgwmfgpjlqdzusvb]denyidxiinzvmhkeads[nuqpppqdsbypxncb]pzqujhpprhbxvnuzis[zxyppxjfqtzdplvbegi]imswdcvwdghzhmyyoci\nmpiwlfpsupluuwzyqte[mtyfeccxfpcorktwam]jtmnexxnxsdutfve[ktzdkimtvwbcjrr]crdupwumoriklqckirt\nclubjinwpyiguop[xummstkqfygcnsu]rektotfjzzguums[hcxlqatyhaqponifaa]vdzuiclpdtepfqmbdiw\nsswrlfxpvbjntaovr[cajokjrogvtnguj]jsyxzvoomnfbtcc[lgpureoznbgrfwv]rbrwjeeiqshuvkwub[gzvyjbprnocmpkyk]gzibarcxnwnvuymlxpn\nwpdzryxwfahiwguwvtz[epyjrrvvjpkuogtflte]shadblrllcaigwocsw\nosmgewmpcqugjqyddn[omtivijufzacwctoaf]rvlwqcfmfuazwlas[wbpvzrbsnzqnhygpexe]vxvfjrrcjutfivtxb\nunyfptkouxbhwwur[atheuhcficbccfur]djycwrtnlttopnjcm[pyocjfcogkyoogo]uoogeqkztdvsgdj\ngdmorpdnzddjtbzo[hxulwsrafnvyxokoe]flzcmbhukjwjfnxsq[bzqqvrmxihbugam]kwwzidcxteeodrcekl[vtjszsdbmsxqouutvkt]whnkvoierxzhehwcjh\nlaswazcejcxyzcocca[utnlyecffzypkiocowm]nievutnusvrsixk\nxlcgrfodctfmyxvsms[bgnofwciyllnekkiqf]knqjmtgrurhsjrwahoz\nenrcvyphrazilaqswz[gdxchlzickidnqfeo]wmadrvyuoczftbdbbij[jxlyycfmgmbujmas]gsreebayzepseakylr\nzeenyzzskgvaysxe[drhsgkqipilrdmcl]xyhouejaqgfdhoshp\nsclmsgjqcijlilhtyn[tyxuebqjqjqdnzg]rfeqmnwynyzfwsfq[jnrjwlqvcnvziqjqnz]zjyeqebxncecsykm[jizuywrcdskgjpv]nkogvpblfiwwnynxf\nrkklgzusmfikiyxsk[zfcqvybbvwxwxlosyhk]pbcybycsiegagdr[jfrnxtonuvihkiueuhz]xlfvapkzcpysqoi\nnllzirippgseojljl[oahmzicssbyckdhyb]qqaeuleefpxlwfl[orimgxtsfwsplrbuppt]eyzeliykpnmmklg\nsypyjddvabqnknl[zfoknkriiqmevubru]rcxkbkzngjzzcchl\nuveautnfudowpkocevc[xqckexnnmsrzxwrgnwo]fbrkssqktfmvbebfs[jmkkvbmhembpojk]vrixaskbnwyzibmtux[evdzaxyibnensgkua]djjjewnszeukvelm\nxcidhycxopgdfgzxp[wcybbxckgqmwttrrvq]zjynrtlsoibooaiqg[zzsjshnyyytzmrcskh]lnvmmzokrgnyqfvsi[kjpgxjqiyimfzec]bpdjsrxzsbwigarmwi\nzytphsjaeavezjmtjf[ocfrxoepijrllfc]gsnkhdomwvsrvmctk\nhjrxkkrrutrkmsiax[zwsclcwdqaukxxwmbgk]jjvxzyshctodfeeonp[eklzpyupurxmcvgndo]neaovsspupkhdclbo\nagrgepnpjdjmmzxtoz[yptupgqukzyiwko]zegusqzhdpylmvhgh[ftclkimlyjeiqxymyc]qplgypcugeybdlznf\nclmaojwiieaxtkf[hybxxzkuvyvljxs]nqyvgwkyfgwgpvjix[ffrpmlqwqbfqfpyn]wewixukrkkavdgpr[zabgeqjcvdsvydus]crgezocdrhjcufljyf\nxwekgqqxadszfqxp[xgftweqykbpaqymyaev]aawdhgjkmwqayhfuja\ntynmzjhrddacgjexrr[kgxebvnmaazmffon]qercmbticxiauyauxmp\nueswrzmngurxaqja[yzlfxoaxangzjbyqm]zrwxnhpmqiespczu\ncaxoesrhrghfcyunxkf[lmalmkbhrhijrvmafw]sdbhqytqtaviurkzi[ozohqgqrkgcbhet]wgwgtjtcfcqzvymnp[zxuhhoxlpsgrfcrejmn]hkopyalfpjzbptgetj\nosmyszkhkpaedzdy[xfincacxeotivra]lksiavomozgiywoxrdu\nfzbuakjjvpyjimycrt[vvbkutdqqtyjgqz]rxzeygtijyrfiqm[qxcgvagpoqyoxhziej]tfoadqfiddsurhergel[sxqvskkcvlkpavpls]ivztxqjuntogjxx\nhphqkgxgqhazalmlqoe[ovhvftdmpwudzdicfkc]tdfnmaosfddlzbhv[obkkfppmoqirgmih]xrsrqaohawnwlxpvq[btfonxzgatdqmohserb]bukakcwcagvcuuwvhtw\ncknwenzzehwdrlje[sctyfugmaxgbetxzf]fcsbyyqvoowzutlge\ngpjdtjgclynikoh[vicphcxycqsiiiglrsw]bcjlerxdimzupbpnw[waevcaeooffjikclq]nhajkvqepdnzgiijfrm[lvmtxqhswljuvux]rnmiklyolpctfrfgxs\nweolymxfeyqemlpxulo[ifjuypsxwrwczhpsw]hziolxpchkfouvegj[svfsshaljdhmwcmu]zqbrupsvenlvvfiuhf\nmxvfnwvzsyldqyi[bvfuwmmrksbxbzcmzrz]wktcxsiresexdodbtl[hijoaneecbrhpmaa]xajfvvnvwcocpcbrhbc\npboivziugjszfopvkwa[kdcvzroeislbcymt]plydaqvkrjbbtlutgvv\ndtzdswmudibubrthcxc[vgmrnyfsqtutxfq]xwbupswdznzazrecwr[ijppmhwabxmhfgcqu]rwvltmqsymbydmqfnzp\nagaxfzobcsjhyutfk[ftmcykjveqrlmvizdt]agbgsgsmhehzvoy\nfbgqlgcyjmcjajxgq[xrxyfyshmvxgquv]ubfzmnkgipmqeucbk[ebcveyedtkxwqcni]dvujsyfjdfowgxfh[oubuurnpwusoxrx]bzxtjgpylljsuruwlq\nnbctombtbcumuwmay[pryqddzmpxgkjlz]bwwebcrzdpkqlex\npvwqgvrjhkhjycm[luquegjefcvhweovots]vddsjvlawwxvkcepqx[xkomwqdwvymcgtgxky]tmjyqmzqxuhzxjekwpw[jdszwjkhkxkkpjjwkvh]jnlsvhnyijndbcavtlh\nccitzedsdvzmktzl[qjtmlhlgdmhomythbe]skkosmhqaqyxvrpwyvi[toqfnarddgzlwhipiqf]vlallikphqpggunc\naapudqmdqsoadhf[bptieajhwtguxpprkdn]fiopmsokjtonmei[rdcwfyvsmtkqwtpzwcg]pmgiakezkvhfiqxw[bmglrvzatxatgooc]jdkxirlaztzghpcgiot\ncsxohvjhmjbjmsw[zgvrfjdvjkjrrsc]wbnhtwfofrquxtzynmy[smcwkfovyaozfhhf]yfribcdfykfzsig\nmzvhznqsykmcdgkphhu[cmmcxolosuhnkmuwhf]gkzgbqwzbzzurzehdm\nyecvknvwvjguxlytj[pncdvmrcqcjmsyix]nvosjrornnfgznaby[tzuoscqaarhjnslab]whvfxspoocikxfkyj\nguaouikkjfrtolsug[tzdjiielpgytyhis]gwwwtmdeetytmerjk[sorwxqfcsuhbvecom]wmfmxfovbdjhajcaxyx\nouvjolrkjyetsqlo[vnadgdxvtdkqlgi]pivwtbhwibflcoh\npuboxtiwmmabyqgn[zhxzdcswdaavgdaly]ksukgpnictzfxxsuqsk[feoibpurptzvrqy]tytogwcrtiofplr\npyeiwajmvimttmi[pkvpbhnufrwpwdwy]dwdpuymdrskpgfwp\nuwctwjpjojxatnyjwm[utlxyebxsfrddigrjh]rwepcpjgrqeafmr\nmcibrhjsqyketegjx[wjiejdvcjjaijnmoy]lsjoughndzzedmblz[ovdcmldcmntnxwk]gtjntfaikfbfhuercc\nxkcadobnrwjczwpo[izovquqhogzhtajgcfu]feiizljlnxughttxhy\nzovyoejioovblepnri[wpjrezfxmhepyyhi]lissctcyvfbtuklymtd[vtakkwrsocdxmyqjkl]idfjftptuoiheqi\nfjylzurwqfvphvctbn[wtraagycimmpycsbtw]zdolnnawyfkozoduzht[wqccswxyzozewtayycz]zngifgtxacyrwiacyd\nmkdselqpwqchnwxgydj[orjtmojhzkuxfbpmxa]udrbphkhzchgiyq[ckkhkoltyjlfzrro]kdyudnkzdsjpvonrw\nbpjaenogjpzaxxkejpa[jqgajznyesxfcdhph]euziwygknckkkkunxux\nbtjnlodtnbaubkvb[topsbnzgxbfanulah]uksjmxxfwfzxqfcij\nzkfnmdwdaviehibtjy[adnmoctsyzhtangoxtk]rjydanokxyuxajmnx[rbamopbudxevhpoezc]mzurnxtacbelmitu[oidbxqghkpqjzyqrrox]ezgwbeyokfmjwblqq\nnwefqukauecrgki[ofkmtkzupjriwlml]diautbiayphukxvmhlo[iggbxeudmmbkayonzyc]hkijrjxiffmncybco\nytgimnonvbqexhbabc[jbkbctatpdataxjqtee]bxzwvqoqyazdgoy\nbjztbbhxzzuannkyvet[mngxjhitobvkzvls]abhmarswjsswftn[ihxeotxkwnknkbmkvjs]iovgdoevhkarwuraoef[wvsvcnptmpcktslrn]ldjniscnknkjaheayp\navmlgtbubxrilqdbvd[eqaifmlaniocwybqh]juzknvgrahckcrhagh\ndyvzlyoefrbtxizlod[ussgexxviaibhrkb]tcgkgkyckgkyewp\njvrsopjyjarbkenouax[gwyjvegfpwvjsdl]crgcqjzhywhasbuzdji[wqqiwpzcllmnopvbf]hpirheoriudpernd\ncpykkvqvowwhoiys[yjoethxfromctdkog]cvlcjvgbugyqvqxjbc[ipyvfwhqyocrksd]dsvipsvdgzruhsli\ngsyxcrknbxxyhvnss[zymlfgpcupgtzycu]sjucevsghhzpuqe[qldvqrwjankaiexmj]cacvncnvtlbnxfybngh\nndbxeywazfrnghgdjog[vncdnjelecbwcnuecit]obhfqkcyucffwbhk[wiboksymurccujv]kxhiktclvdsgbxt\nieqiuumamwhkexjene[tubauuniiqmzdntax]kxiqlujdvpjqqrtkiy[ubnpvsfjutgvfhpe]fnwawoyfoqqdgyr\nlromgmscqlmoqtqrr[wbndhgvivyrvevwpbd]fjvqzyqdkqfpica[isfiiygygruduhleff]lbfsdwsbvndxjord[zmgvcnxjevefjnqx]izvrxpsfekwsaxhzg\nvfqitwljrqvsyilpb[ugzycuwrexfoavmalm]dshatbrosrihtwpf\nhduooarqszvabcwukj[ajuwsrthbgchctbyuyj]tpzioxoqtyfuwtdccn[jisrxrmnmzhnhotwra]swseywswdlsbzzqqlv\naarocdgubnvehgg[xvfugpdczaccgttycv]nhzocbyrdhlppydelyq[uloucbldnjeulomssv]ayxgxkrslthaspz\ndhyljzgyamlcdmmz[zdkwfrroodcyfnfie]zkwhzngaidridcagekh[emzeeodcnuvzddnbm]vtwokrqakoovvcdisvm[nzdlsyrpcsicoedyx]rrnfnhgpaeqtlxv\nnxybztwairyftfvig[syeyundkruexgbwyvz]pspeqstftxbbaevhql\nsbbhfvvgyscleyxzki[hgjoiilqwuiiogtt]sblfjsptehcxdilpgw\nfmynycbkkkiwjllu[iolpwypqrdrnkitax]fwfzssjntanttkkboq[afgwfwvsudpprmpne]fbzhbkoxpxavaskchfq\njcyrspmtzwxqtomkqab[xqivjfrwadfvtfmp]fxkhdbiczckphwhil[ztemqpsvuwhwhfdfip]zxqetcaulofvxrsak\nozgxtokkrotpphxsnt[txgvekxlxkhufcwi]hspcyxwyijgjaqsyfw[bcjgsvsfzmvjklh]bxjmkqkynrusvvq\nwofaptbytcugaluqc[qdgdqupqigweysdhq]saaeqyqazqqaunofl[iorcsdtwdhfmajh]owdrcjffsvszwflax\nicrmudvzysqefbfgpae[uypfoutavxnzfpcfafy]moghronhxpgorkpypoi[ayrgvytktzzwtfuvfxm]ktoiazynmsksawusbsv[vypyasahxszocsfrcx]wyodebbscuterfrji\notrgqclsvnjpznt[dwzibvrmtngomacr]xtqtbpxdtejwbstddr\ncsiarmhcmunsjogtwp[nborrnynefhrgwy]lvsacfkgakkbjyny\nijejwezkizvuswn[zfkgmewadvwroqibng]kqhmbrdzuvhcwkwxfwe[mgopomvjdemllzygc]ivzzvgcwpmgjewb\njznavprnlcygwvvj[eobpbcbuqceogtei]jilcppgbqnzzjrjjjx[xurpitsmdxtiihb]pkwkdkckicticboagma\nhrarppjudvbccxdepdg[ksabupqjypyrwctd]jzmkavpyparwxrivfq\nkjtgdhvqyzisomc[koywiyiymrrjpbqno]vbbusjzesxjpwkrh[zfalkzmohlxcdykl]hdctcfabyzteadzofca[vlbsevgalpsvreryxda]oocgdkoeoxgepsikokz\nnckfsyxjdgmgcdyqoaz[cegnbhaksrdfaokttjc]rmfzhgwbszywwzbzpe[nofsbyxiguiaxju]vjjitkzyrugozdspwjy[gwkdakutwllydivtnns]gswugowdiouemkrf\nevjgxyciglvcnkjdep[ixmlhpvkldxvcerjb]eqpkpmyqvctcepuljz[aylvsdrrbajlptvfeo]nqmtctitzqxeluw[pkylojlgnaunmolry]patyaqnazqoykcls\nyklraufwcbbewrzdnl[dfsdynavgwiwbkmmpo]atqaaprzieowbqafr[udtaocwgbvqqztkykeh]eyzakgtvzrmejksf\ngplhegstsxbqvxtnp[sheoxtsrbdxposgmtx]fazbemqbzmssyce\nulhekckzsguaeuectg[msnwinlfedcaqdyb]przurxwotscdzgtcjv[sbqdcqeculwutvfecqm]mjosilvbpgaawll\nbjohxvdcujujaoxe[buibijjxplrerpiphn]eorjpmrcugznwsi\nyflomjbhtnsgkkx[hhpskaiqhzlmbnpv]lgsdbeankbosyptonh[vxodyzameaaajwc]nwpmycktztqrgmxgbg\neajkclofrzpwbscfuwv[vgcyrfqnycmarafkjc]yfrtobkpkwlmgyckhmt\nczamuejkegyxhetxmou[edrrdhmhhtxvpoxvx]wbzihlibvexqyvclzml[dnzwkagaeyicaojzg]wkireqqnngbfxsygz\nkwbjoaorrluxekext[ffjrmxvgeqyaoartr]pwxypyiquumrhbz\npyxpvbqfwlpnawrygi[dtqrrjolckhpczlk]mtknbyltlictunxq\ncgwtgnafiflwgoims[qdbdbgkqhmtkzmmyuke]cuhipgoscmxtoihh[ieqobhwtcxsehgils]pmtyremzeqhcuinxs\nlmcuchgkedjkgbvxjdw[jxqmqodwyieikurcwf]mkfmofgbnxsmluu[rymmyeyhyncfnzobk]jnwjbmejttstvhumye\nqsuhfviyinfcwufzu[pqmeenwhbstgguzs]ypqszcvmaxfqwqcvqro[xiofditiroisnpbx]vhftrwgnrxoxciva[esrtbbadduxicftf]vcslxziacmscxaxvnbs\nbbfcqaoedfdwphomkh[jnslunmdmvkiyup]gfnnjqweocbybtjdtn\nsrjpaxfvehavomsjq[nqqcwddbzqvxdacdep]hhpbhajjqaazpqyo[fclqwfkctufgmkqm]pzkwekfirzlcgduifqu\nkfmoszcssmucztdn[tllxhkubjuqjmgfeqw]djyeyajqakxkoxpk\npeeaqxjifuloiujd[tgplullzdgeqjononx]lsmrbynngeveozz\nchytpljkoqzhxfu[izwdbatnmmzzttst]pkfsahxrlgxedvsev[rcxdfirqmtavigilk]lvrudkskrxxyulbjbe\niatlnhdapqsyskgstls[nqzlofurrzibukxddw]yxdwqadthjynwvatmp[bdkndmhtngzerzwqgmx]iclavwyossjrhtoqf\nvvanifuojsytdel[dmqjrwfgjqrcyazxa]mivahklphnoapabp[tlwiiuvxlonsucr]fccfhxkvvqeqvclcnr[rankwbxciojgzdhuuu]eycbcqhnkawkwmkxb\nkyqnkbwfvcarqcrcfua[toxpqnxiuyvfjlekjk]hfponcmqqsfdzqtlgm\nksrmipfvtrgwofiqxx[dxncthyfpoivapdpf]tzlnjrfggtbgdxec[tmlpzqicqjfhxwjcigo]uzmkhvbltpwdbpxzfpi[yfkkmkzokekiidxpugj]jbmagsjlfozkajt\nxhrfhwrsgduyobjodd[pazkwxnflbwbpwxych]yvasgopohztnfcsbc[dohwmwtdklyjkbaqe]cttccmlckzlioizfufc\nlygkfdlnlrukwjskxqp[tcskymqclunvdqywv]rhxfxbjftjxdepuwax[eoqchqlngjnnshc]gvjhyrvjgueweik\ncehpocjxzxkpnxglhzc[ltjmejyuouzkisdnlah]ytzdlqcewgwzxdz[hcupzenhdmtvigdodq]oivalfgkscgnaxih[opciwwcvzkrsehcznh]iveqylobdjvqqrbb\nofluwuxajcsnkanvg[vwpsezopzkpvhlobfos]gmnrtcprhthefopis[yvcgpesbspnlbvdcdj]unooggcrpjinkxmqsg[stfmzxmnwkyujhwqilj]editpyjnpwaefawwq\ncdneyarppztbtwsaqy[euyswrwxaaolxkzgcx]cqqabzealhvuwzo[hvnmwoqlzyjguvyy]goqjeapcwghvfszwsc\nhohlnwotueozwhyfgg[bdiawrubvrnulfemv]yohmiujjdfjexybb[uyyzvnainybidqfmll]pyybgwdxcdqdgjp[qpowhiuynwospqdgui]lqdoiaufqbqljkvhgjj\ntirxyuvikznzsavp[omifkdfvljmhlrk]ouzmaxynnznyhfrud\niyoipjyrywuhpipcx[zkrusibgupcteuls]rkwpwfppboaxzgkbwuh\nyebynyhsovfufkhwoel[rqgwgiuuztoboxqo]tbcahalhrqzpqxhud\nmxvixuvpntcsxjzvpy[jnjtyjwuivtsxlko]zugkjugtwymssxd\nddxewdmzqrmjcdx[tehlbyapxxetbkp]lkfkrutmzvjsvynmt[aryjfitktobzfnhcxu]rrbqdbzhgjwwnfpkxbx[ggbsnbwuwlduhlfp]bdniebubtcxsubscaad\nosbvoidqyhsnydypy[virseojzmlplzxfwcdk]qyyespqaegmtzgckltr[kjowbsggjlyrbtcxj]poychjfbatvhkrs\nrlvvjqnaiasedvpjbr[fufrhampzwdniipjc]oqjmidcyiekvayqfl\nhvtczuskhiykvchxno[benlaiuubpaghzlwbf]tarjrksfzvilwquxj[wehwbwsxfuaptyty]gvvlkkyayfstbcut[hxnojqaxevtbvmaz]jnhvumhqfgkaqhumxt\nthxtkuentusmryim[hzgibspwboqacdlwc]clsunqcnrlgldjbsvz[scnclutgijjilirutnn]izdwhvipobyzirg[hliollkyedcuomrwyyq]dpibjmbezvzyspmkgwj\napezafwfsqifmip[kuxynugvrndkdifwhd]pixpqmsbuqspsdpqnzw[qfiqdwcdzbtidgm]otzbkrciacwchdnqa[kiblvlkmtkqjzyyv]hnucmptrhrodosk\nnuiovzzixafjgvl[slswktlejrrsmxujjrk]cjassomselslooj\nvnlustrakmrdrkjwju[nnlzyowyjshralbkgo]jpwjwpehndfweegrnq\nhdiueeojljpcqrdkdfk[aseznfnjilqktdx]fubppvpqwksxeiwpm\nkjlbdmnhtzcagcpc[wybonbamfkugypt]gnjrawnjietdzhaf\nufmoyzcmcxoqqpsg[hkdzmupftmazbrhul]mypsxfpshzcirslsq[rumehwhrobhrjstjd]tcdatsxbxwzxseileyd[iwyafcoefsrbynl]vedzteatonqliwgyj\nwtmyhvmsfoxphqrusjw[ozpswsyjxemnczhga]xeplvzvjzdgqspqjv\nwxyocgbulqhbzyekcln[dijevkhdfkfwmppnert]uuxxnhhkbmcegbtugap\nijgtsfvyzgrzjonlq[bxxhmrfelsyxkyxrex]pimhbbzahddhwrhudyo\nydjcoqvktwdjucx[riqvhezqqrwpizvn]pptmsnmubbjzwozxy[rbzbtfnnkeyuvjqhjhu]hnqyyqccouflfzmk\ndordtdxwtwahcjcb[gumvtsackxhwojebt]gdzjirhxegmrgishf[ueivwcnfptgagdj]kzqyptwgfykrxqsc\nyovgolzpfuxumuusnu[yzmsckgxuxbcfhpovdi]ydcgpjfgjgstljbkc[jnxpktvohnxeoett]wijsttknnkaxhyx\nxaajqzktqfslihurb[ssufsbsajcwrysbaweg]odddpcsenmcxilrkp\nlhkzyewhnntocluc[witlpxxovbpaeue]zokmfkrsuzblnubzq[qbubewghnsjcnbku]xicstwzulnzadvwgv\npzuhirxrvaghkajqsg[edyrpkukyvidoqbabcu]vfqcnorzlzxypla\nxythdypgcqkccfv[zrbuwbhkohddkmbj]dbkreagpyprchmoktz[mehstplzokdjkasge]bypysrypwfqaupkwmad[ywkktyjruqqoexms]xdvcvnaeuiwdtcjcwg\nebmymncvgrkqlusommh[wtkwqtpboedpdwaxoxv]iezxkyrvialjrev\nnjvacohjeagiztos[afpmzgmxbvpzrkpikb]cxbsozlksnpvdxh\nwnpqmnhzhaclqkn[neseqjerkxmpddehzpv]buwoodytrhkaffpb[zpqzycmuzkevvyl]iqdqjuqnmddqdmktojn[ocbknhhzdyzcpzi]srfnmfblqrqzwtusu\npaxcryjinpwgadnzgdn[pedljgwehinbuvueies]wykembvekyliivgd[mjonnndjrswlfvlo]vuanwryeqmmovavhf[pouuyesundysqaxzciv]itixbjpcioinvfkh\nvmlgtgupmvpnwkh[cpuwomxbeionmrkx]zwjdjcytxjxbzltbp\ngxbttoltnwfholw[srbxnbzsdlwegml]ufeghhwivplxych[kesniuppshrvbic]ongllrrsyzxurhxc[ucssycrhethdlhyzd]jvhniomjxluggwtcv\nkpwrbbrusxmusejnwz[wbgriazubzccotlcdbh]dxnvqwslhdxbbufe[pobrzwumffnjxfghv]qplrnuqjguonrpmpv[xxwugdzbckpvhhr]vbrmirtrwprtqli\nmlonozngubrbmumjxb[vzvxodkubovdionkb]uidfhtqhxxsetsnvy[spdgbqevotzyzhtyy]mjvctpqrtpxrbqeckq\nwftjnmpwffdunhwr[nzepzikompkwgje]rahnwuphbxpmwmtwboe[wcwxzwqppyaeihnxrvi]wozbvaemreqcvsoafr\nlmfgslqcwpzvgxgmgty[ihjhsbvhdnsbkroszc]scwicucudbqrvtygt[iomkilvjwsofqnjqtd]amzyfxiaogrsdikrgye\nfcjsdhrxjiuugivwyk[kazerfwbmgeiituwksg]nalxpcedxoajytfpg[lldrwcgzwhmukpmsvot]yzsnbooxncfhjdqi\nljjwrowxmpvvwvsit[lhezgrfdcwohtllany]huqtnutwnuamaahpwa[ezoifbtagkrzzjybsf]fehkkskjziztlravf\nqggqdwibskgshrkyc[bcqhsghufawaskgezjl]tikipezkvitcxtefpg[rwvlyjcgevwbikop]ygxubvtkciptbhi\ngmlqugapdwdohic[fbxygwjlnwqygmnxma]sgnfeprkyxrzspd\ngtokbujgojpkdtrvt[hxtbjjffjwxnpco]vaxogwcclwrodfdxlfp[hihtvdymxjotbfuyfr]muubeuzwzbdsydkkss\nrpqdqfjuutdfbaarkgb[nihwtvhhcmxwbgr]evovoyejllhtmpv[qvkudqduftuvccmeby]caeupguvwobwkccojl\ngxqxcqpcbqmscefvj[jodkjejtlvhhyrw]ciduukfamepbpemyol[uchoefnuqlolilidyp]rsjsqlxmjccoipqueq[qlxonqxtccxuwcnrizs]plzdntlmgcnrwawrxdm\njvbbytsctqrwjrdr[xtqorzwdmhunrtevfb]qqxbyumulbmrsbhtx\nyoenmlwliczccpkolc[xsolpcnqbbkrani]tzczkjomtarfeqiq\nogxowfxoqczptla[ayzmunzjrhsyyit]ckixtyzdkicgemx[hhubqmeqeenjuwuclx]zjhusfgvemklroia\nwtnnwdcuqnxduod[nugtcdeviqkajsqxgvh]ujsnisiydziqndzgtn\neylerocwshewgerk[szefiobgoejulsas]jxmoefzlxhchgmspo\nnnwqedoiuhqmmbqewzx[ocxrbmgeqxsjeorfrde]agqexvigcnntkdck[vopzcxqdokfydsh]aajrpilxdhftxbprqn\ngieaqwfwcaktnyrak[ckstsfspnaxvkkecu]nywzcpsrpeypytm\nnlsmbjepecyztmhys[yseyspewhduijglnxs]nmttyybnzhxcbuvcm\ngzimfexrobypudb[fmrtikpcalnxzjco]qbxokzuhvtgzerkwgig[otsumbzbiecnrsfvgox]pnbeigikjxbnesh[ifovbpoycogawpmbtuj]qjoaetsrenrirpvb\nybjllzyznkniidrl[txlisrbknkopgbgutv]rspeuydexyushei\nnnigaodunsopocfqf[fdkbcjzyxamtnwn]obloxevzqyrmswtc[jkuniykbwsytpivsh]ceuzwuogyqxferdic\ngyuypjyncazpjtbni[aietrzglhhgxscvnwvu]ccqmabbzdawwoctwywe[fassebimijhpenb]bwqtcbfdilruikksetv\nldxvntffkplnjgt[lhwtwwfoyuoumxngqbp]eyoreivfgqwyfet[ylipomgffukvmjynvu]npvyofzmqlyboidqya\ntpnxkxbhphxzetonae[sugfadsgjpdwxup]jainzhhwfvgcljydo\nuzllwzqtwsmvdpoivdm[geidfnypnnnszjjgc]vtwpieaxgzxbslxld\nlzeizipamzynfflhuhz[qzwbfnjeulpgjjn]aapdqkjbpljvnvt[qhauhykubojxcoyuglc]tkflnjrdtjgwilk[aorfkrzlpuhgozwyhj]kmbwxqqwfjxawbj\nivqhauvcbmbzijrl[lbsmgujvpbayaoy]kteathfvlzvbfzdgw[xkpwoqzbkbdgrsjzn]hnihhzpetldtahy[ocottuvddcefplijb]vfolexdinkkgmcdwfyc\nvqblvnbutgxixnfcwc[kphevjpgctxpkavh]riyfeqvpyvgckaselrb[ryoltaxliqsnlqdagr]shrflexwtlaivfow\nlreoiyjedxzdyhdnlde[levshlupfrkvdfdeav]ehfmfwbetbsduiudzr[uoxbgzrwlqkbkcwo]wjlwlixknhzeuyw\nabnhwwybagtjfrh[jaoeeifkdmlksncnjp]rulgazssxsmrrwe[hisspgixyvssxiumqtj]ohkxzqzkfnkvvgvrhgf\ndrtqdxxqsrkujjyyb[jxitdcumljupwcmxx]kmzgykavruhbplvjjp[tjxjcibazngasivc]iuhgnmtzaozykgtedes[pproeupegraihkv]vuptfrfnrwopiczzkos\nkbkxcesohyjlgyynpwe[bkintqjcoqshvve]torkeaaagbkbxosriuc\nqklkbdielutwmtwkgz[dtruujvmzvmannceu]xmrwrcevkgapcagtuof[ebouhjnkpgmqairnh]trgbvkjhgjvqmceu\nxcoycanpxtathanw[xdfzqcekyrgixxcc]zpbmkgrykuvlldgzh[zltkqabodeywxhtyfkc]jzetstuqnplogpkjyx\npirttznzezsktas[ogefjszaezeqipdhy]tfzgyjkulhtyuhnvf\nkxyvrtcpdqieyro[wnvmnmiobotxsispv]qyvdfrfhxkjuqwdtw[qolhrtzasgthtplihxg]gfjpittpnbsymvnotyj[znwgxnufnotguzwgwxd]rdmgzgfprxmavttnoz\nmubjhrjxqggcrus[ammffdekmguajiq]wvtsxaabnjzbekpx[thnwbdcskocytas]yimpbasvxqiylaqn[mrrzwqztanrkdqwvw]uvtlhtffzkcautuvm\nxbnvzradisweizc[ogurjxmpvzglqbgjlpc]hhujtmvfmcqqcukjvjp[wgkwvyjkwkufvventj]ehdkswmxyekfimbk[ovbdceenqmnrjeqvf]oqvujeqvjlplnzgi\nggbrbreeteveahudoxy[wuvddvvvugkdows]ftzrwbghewsdfqaigt\nshelsgoglooyenhx[lylymuuhrtnflwww]muaexmsuihzdiyly\nslmxqaktxwfpfgrqv[ekjhbymdpfpiqvm]zybjhwobkrylohor[xflqcdxcgvqpzzdd]txshvtkbijbkbnsh\nbpocmihqoplucwnvyb[scxgrmfmuycybgura]yupkvewviiggoszst[suowhbqfktiboyik]hqqmqjvjczoxgeoqof\nelmexemdeoaajpjhu[kilercdwmwidrkpx]pvyefsmytxvaxuzsq[xyyhrtmwtglmcqik]spnsavadaexrodemqbq[wzzqmadwqbqbuvdxpmv]tuvloljoyhrqccyd\nrzngofliosgytzkunp[cyjzxhswcqeeqhmkjn]ymhsqcfuowylqtjrb[pwocjlxtfqsmelq]ezhrwjlzjtsdqorfsn[iekekpprqmwpdyl]aduyoxkvlkxejyjnqdz\nyhwdblscdqhpdbthaac[xadcyjrkldvjlntkxl]tcohssfmczzbomezqdr[wspvzvkctwmmhfujxm]fgxpvtsninxayplzlas[poflalkhzwwqwotgldo]mihbeaapilajefhlxs\nxgwckmpjphdwvzujv[svfqqafftzlgoifup]pezixwriwatkcez\nmfgtxxoygegwmitbzkt[qxivglwljmpsfzn]mfvhkhhddithgxaokf\nnpkhgeapbthebsqk[bwoqhnxqzhkkwcm]alwpwqgoitrupvsz[yqvcrithxqfdgzux]adoiatxqsplvllzivzb[fcfyicpoiqaagrb]lummgoxyspqibxaq\nvikqemveklzlaqdxvev[tsqfmvvhysvdmlspknc]ejryfsjgnpmxcvks[ecwobztvirmokwcf]siwzbkgxlniwnmhzyhd\nltlhegkfxhbndmfcpo[pmcjzvzmerxvsdo]dijdhpewjuwnatewmg[ylninmvyjhiqvicagy]cqrtolyldnbzfufnju\nmxsbpkqgsuhpvsrwzdl[dlrlhbdjvmrjwwthq]rqowmkoukgclzrfh[djjugwzxaaqtqavlo]gdzvdzibnckhkqb[xvfheuckvskmouv]uwrmeqlloqbtbfc\nemfplgnlzranlwxnk[ubuhxoejgoxfciarjtr]uzcfagjxdfnewbxxcb\ntlkmvlcqcbaqozlwn[lbupwjeefgtoovnrkkh]sdzgkexzxzcpdjgaid[qisspueisheejzkfxdi]inhxlauecmmkpenqqf\nfdtrgsgechhugwnidpi[dtwwiqlxgtadmnrtej]hdgoyjhlzdrcjzvl\nmtglmkersierfaishps[gilijizfqdzqihkbsd]ieqqthavsiqbkxvrmll[oxznuqiocyxjzymxm]epuxtetrnfrzrlqd[gooprerdkioisowygrb]zzowrurkwngpvvh\ntznoyelqlffpalatbs[cmtlsjviihyavtxz]lphzihbzjykeuhuzpg[xqfwolpahmfquhuh]rpqawvkxodxmvfhswz\nybityzvtpsfbovx[yrggwxpkqjtzdvkr]gphdlfythiokoitpcjx[wmfvcehazqfxesy]utjcvxaybxcikaqgrx\nolqndwuwjvfqhxt[qfgqmmyeowawqckfh]ngkiagyxtqpdwbrwlm\nukuozdurxxrvljkoi[eysjyckwyiyuopa]fconkkukvvmgnvyn[nwkqsifcwlzjurruho]ryslsdfmhgesmdf\ntlchnjfxtkubrlta[rsqsxplnikmqxsyhyoq]xcytyjjduledlzhuh[qudvljyfmodytzaw]hspqkfbkjtsvcwpl[ptfjakjrpvqcqcuhmf]inxwobxnnzfirnvgmmr\ngaviilzxljsozua[vmqvdrqoqnztbdmzstt]ufxaggbphqyxgnpcgzm[zglcpiqjhahiqcb]tsiqxcvrwvqistphkj[ebajnjrqotekcerg]kciocwshxzksmunx\ncgpgikxsukwvmwi[janhpuvmccsdahfk]rrmkjehchkefwnz[plbujeqhgjvljzkwg]ttwfjicxkkofysgob\ngirkwjuugyxtovkjr[htizrvsispydidi]wqdtgvsfnuisigmalai\najbikjzwulcmizeoasw[pkkgiucjnrubiwqoll]gscdqocmpsuvfznqhah[rztusgyvsxaeqfmesh]rarydwrmadghrjtx\nhxpxckfcwipinrxk[morfsambyhipqzwl]wzgttlcuikfpvywm[cyebxypkgvxhope]dqazfmcgyppybetn\nnrisbenoupwrstlxy[uewucgmzkoyulfbt]bbvorytlrgqknqz[zwseofceynlohaooxzm]hfzyxxxfpjmubbjysld[tetgwcwvhctlndovx]jxflzwtuhkltaqmnuh\nnmyrirhwawjtgcgma[ilkcycomeqvcsuwmmq]iridicawanwkaeumbvz\nsunhpdrgrjztzvkxnl[mtztitboyfmtysqeqzl]unugkiwrweincocilom\njhoqhwlkzccmtrlrs[tazackiqztlndogrmgz]zsfezvlpuzwmfwee[vcfxoionmgpezbalm]ujdbonopokhkgynmhp[pcdhdmwegmihhkh]dgjjkcyuetspltxpl\nsiocivjbvwhltkyk[imgupkeeknlltlk]qxfcqnjbjtenubcjasr\nhswgnfwswhyngohhyvo[vamsrkcpvakzvbsvls]ehqrevmxiccgfsq[pffckymkoredwdpcmx]vjdjsrqxttbfjqf\nqemtumhnmgkgfzfzqho[wfluvctfqhrwznyzfsa]zriirahfdpleznfto[dugecvltxsfumxvjaah]lvudvknmsbudzxoadg\nmvrjzvsrconakgifqj[ehgbxxxhfqcigyhuyya]eqofdufzntqtsjukffc[hbzrfurkracnfeig]zmahsqiqbinnlhnvrz[qdajsuhymeavrqpdoy]nspfggpgnwnalzuk\nsejkhhjswpiqukaddwc[vwdsuuxtfaxqbrcne]njkrzolxoqpmmua\nfumcwsiexfoqklovype[bzxfxytncrmwtfrojv]bfvsmplxarmselz[nrnsymdrakyaqzwivoe]fpvboftrzvkemjgqt[akiqkjrmnvhucjcxk]ynityzhxqopnjpslhg\nmsoqujlsilpcgchprz[gqdevmuryxipqcgfdwz]wxjkmuhjootmigfietn[flfcoqhksuopnwk]cewizdzpgetongprkb[pqizytyliwhnetg]uknrvmoahsbicmeg\nevyofxtcsyfbjtbml[wjqpsedellhzgmvk]emdpcwxuuaccubksbqb[krehpfhgyibfxepo]imvfvflnagwulpcp[cldtyjrcehkgtfyxnws]gaicllkdzufdmja\nplinmvdjkaswskiw[zejltttlwtcetjb]uqkwaifdtedvcmiqcs[smlzeqfmbhssmvvmvh]lgypwtxchfxksqgmeb[fqygohnnxmmvazctrl]rwbjopgpdkeejeb\nhgxczafqluesrmrtuc[jkowxyxlufhgbmk]zbiycjiafsngeoz[mltnmcbnsrmdjini]wtokbcbelvzibjncpat[dmjqentqrspifbnind]drpbucndawosqjk\nhqaysnyyigyfvzsm[vrqjwqmhiywsbblfrq]wseacbmleqwlaci[eisrrgcmewmlsqkremg]hfqkdkghomzddiaeq\nqrcyyzpfuupvipsuor[ujvnwghyvsujblbiwy]uofftaesrxvghupknr[divaemcywwpnkeejjo]dmgdiifbkggxpzmfy\nqjttccgwnqwdehsoz[dfbrkdapobhqvzom]hqtnzkmtiunvomn\nirxyxnmdlzgxmpg[ityfjgihvzrylygz]qollizryghyxjglce\nbnibapdblbaoehfbvin[kmummoqopswsmvtgiz]isaumuoiybqckfvkhx\nwaimkuqinxbmazab[foxenwzsxkkupwo]yjelgjycvabztzb\nexxvbdzpyswekjnfmef[tjmrddaazxyynamc]nambmdtnmfhtkiyqqct[patbobzwiwlidazpoc]nzbneeilwcjqnxqwh\nobtckokgcgcwbtyww[gxpfdpaggfbadjvdo]trethfifqwrfexv[uiucztyublzgcky]msapdqrbpbwxkoeuidi\nyfhewfkbdwvgwvmhqbd[fqginmtqmkcubfvci]aidxbpzcktshamejexi\njjjryxfwjklxrkhhcxu[gwwrmyzrpjmjtmfl]fvjaxkdviibxaodo[csagiwfbhogtnpixzc]miorozrdmimmefh\ntzpxkatetacnqzombnn[bwzhrlkgwcolxczvcbg]rplchqjvjthsortjqb[oyqjdlyeyqhqtrfbfh]munhcovgrhuwhvkjzja\nslrtmwlceytivwzb[xapqxilotekdngaekz]rzohiqiljdhennylmk[whtwrgrfpxkgqrs]rtlehyggcuplhrfwsvs\nvjregfcqrdxbfntljq[xpfnzsjsmphfbppf]kwfjfcrvygtqwtdgh\nmnrnbytuhhsxrzgz[nzdxekogduhxbpipobg]ydgjseiypncodnm[oylueeldnmgcwmqhq]svqllgtwmhshzqaxf\nxhcxtoxuqumfxatsl[qlkqdcziwtbclcph]ysfpbfueqmlluib[jjvxhqopyhgxgvb]flovcgpyjyubpbdmp\nnvpcfbzmykatqdpgpv[eywcemzcjnlhwhfbjv]gcnnnrxczlzbtufuie\nrhikymyqgbqbwgw[eeitheuwdamcndqibp]aiikebogsqexfbob[tcsuzyilztxrrqa]wutfkolihzuhbvptoqn\nkokyhjebbwniohsgrbr[ggsocxmupmielega]esekvzvbajssesin[ipwqyvkwospydzpmk]byhqabwpjuihcpgipx\npizgcsuyqldtehjc[utwlsnwndcjqnndpppe]qxzxhkayzcicvstxiws[tjqhoiifvxdzdkigtb]zjquhrplvjxruwjpyl\noadivwkprasfyitu[yygivqpjckczybxrq]bezhtnyscekflpszt[eqvoapqpfnmwddehqbe]mnkqjstlvogsipe[vmcrcaytblgxyarcrx]nwvjubzclcaxtdmgl\ngimpphsdpyklrcsbk[qphbkjzijutqysed]fpokchopspibqiyyb[owxliqxhpvjjqjzvs]ttjeutzqspjqklxsx[nvxybvsgtxxwagkvg]pximctvjdqxbodwbid\nxmgqacsovxksrfnypy[jjybvmwissplkcttnp]ksakyoqvswnbrezeze\nxoxquvrpgiiopvepjd[xakbfdhgtdrxixz]uuidqssmeiardumqppv[ewdkbrnwbodzzyb]kuyvmhqxititvvmf\nujuuypsguepvtqiurq[psgjujogkcbqrtrr]ckjvvhzookepzzwyuye\nlwnhrcbjrjqarzdx[jezkqlffqqbioajjbnl]zssjjsdouwbegdbnxx\njghqoqlqghfqdfh[jswcksaiwouxhnssqin]kqcasjkrnihqmenbqbh[mgpmbwkzuduzsmnjb]dxsvhizedmabyjo[rbupdqkkgeihkywitk]pcgvmkrlpkbqfhune\neopvqwwlvntomltpv[bwkbunwyjojuxoteyua]arbceqrmsflnytkl\nrcgjbumerakfnebou[qimexcxydncncunkhv]frixowswdjgqndoos[zkjdmnsofgvagtnlyph]efpdksfvricswsrn[vxscblhqnzquxmxw]dxnstwznvmwyawith\nzjddycxtbubaliviw[cwmjgucnnrbsybtpxu]zhmadkawbwtdlnjwb[qovxqaebehomoacpxyw]qctfbtyvbabebup[bwqjuutjmbgfdznqfa]jzitebxzsshsmoge\nhogrxyrrvjayayny[kdweaxnjncgvxhpud]orhfjkslldcjiokooob\njdduztuhjzvbooejd[mcudzrhxonujxksbibe]ybhfelrayyxuuhuwmyx[lgshxdlzxbzcwhuru]zdkvnjkyhausdby\nxsuzxmrqkqtxmchz[dmgddhaltnlpfzkf]dexcfjfqdnajuzccluj\nezpxycrcxzxycllpyc[stdgybwrxfzewkqqvzx]sxivpekfrrrqlfhg[nolxlfvwwqvkhou]psuyhkfiyohkogwfmt[zxwiqmslanvyrquhqa]fereljocexswrvs\naeogravcbprgitmqedh[yjqbxvjwrcrbyneghi]lugbamrjgzqaixjxpa[zpvvfxavievwanxkedz]zksdwfkwtrmtaoy\nmvchajtfbplmslzxhk[pmkjinpckdvwjliz]lwigecrikkyoijkeow\nfnwfspmlakldfdhc[ujbeoudcbtqjmjy]tgitkdutjdhlrkwbts[upqsuxqtzrmwgmbjqyx]ayaivsgiqcuzizeau[fiqnymhyqjapvri]eioouxtbfwduighy\ndcuvsezsqwjnsvlqzah[jjzbyxctqhdxfuqer]wztjqxgjynojjur[zkiosthyfrroydaykyc]ocihuyyzvwdoixygzk[psaghlhtqoptvsldbdi]zxqwrhusqligxnoa\ntjzqnocojjzktgk[omlfecncaondrqrvwyw]dxwuwvsdiehvzqmafo[ihbhwnmxkbkypmum]enkexramnrjguwuxq\nftdnelzrwzvxobrhjtb[kwnjqdhwztogpvvt]frxznutubezaczhwucd\nwtvnfoqoqvuioaotdqv[qwzmcsqjvpkrudkdu]vdcgzytjsihjytaunui[vxnbnlwvtribvbzv]lclrytcczbraubnr[fptsjqwofyngtnurf]izhrnmwjxwvsdcfai\nnqmhpgsurlnnjikyotm[nxxdysiylpgivpuc]uofofpqgcbojfofja[gmborbfjvlfokmkjlx]yptrgkpiarzgsgl\npolwihnjvtlojae[iyjbafwjoxqcjbwn]ecidvqragdcuotbw[ununcsfdoxstecbass]knnitckftuczdpblih[wylrqjxehihxfvzjn]lpjuibfkwrcmcijkho\ngsvfujdbedschya[owwscbzhfkkymsfy]bbxedxnzigfiogb[sebiwzxbshqohku]wqmnnhmldplmhwnngu\ncvgevjryjbmodqfw[jskismdjblbsjgmhilp]xhjlblnepxqayxpw[pmifrcxnxmadetumwm]lvjmmbceghwqdmk\njgssirdflqhglgopgx[epcwzeqqkidejdrw]mjnozbbmubmqooiqr[wacqyepsgljjipi]vowguayfwcghbghhoyp\ntfkqxobejvvmglhqrgw[ddleaoforgpypavf]flnaiggwuxdbldb[rqqrjlzosctaouurtsr]bduvfxlomgfdwhxj\niwhaxbggngkgdfi[xklwprhyorwyfcyo]lbrfcbprxedylzpfjk\nixorpegqzuxidsasn[pwuwcywpavudpbkmdrk]stfjklbehmjdobcr[ziugachuezezjsw]dzwuijfiexsbbxjcga\nlcstmefgsfxelap[iaroxcldkoxjprhpni]erzoueqtwtyftuvz\ngsnvneyjuacyhipd[aglvnvpawajzbbgk]ptnrpilavksgzjyyo\nfrxawoaynynrnxzk[agbtdjypjtpqskh]ljshzsnnynqotgog[ckariglbjzvbcedrap]sqdkygpetxuwfnk\nnuxleplcklptuce[fxsyqwfblquzwqjw]ndnvzriqecbqphdoc[pmvfypuinsxgglg]vcgzvoddzudwrapmyh[laengialdtihgzitt]ktbypjipfpnczyqw\nsnghsdifwlabsbpzw[xgnrqjnhwdqkbhowzaz]cygljjwohwpzvxuaw\nhhxorrjxjnhcavt[lkeigkktbiaquqqh]ernbnsmtunqyccft[jiespyeonlsjliwt]vbhzvdhvvgsdgijg[lkxvfabwpujiaeaidj]dkilxjpizbzeqxkzt\nukgapmfifvftpexnr[jydugqlbqyhvbsmoxd]kwvttiyqdmyaxidts[lqfofueuycoihkxig]vqbdiqazwnqetguq[fxhgbqqsilfcaflj]oissblxkisbkmolspwp\nhanudfleaqpnnykwfu[kllfsqanmahiwkqz]mkyztkpwilxirukacz[vnwdxbzbjrcvmmbx]lsjlgrnzdilnkxp[hhepketmdumjgjjsu]zrgaagprkrmgggpk\nqcaodhkekjwrjeu[bvbkikapkhneodeaqox]xxshbrfdxgvyabbuj[nnyshhdaogsermyisk]ieutdajlitenkmoh\nryfcblckaejcahgy[kymhoizkyffsxybzdta]olmhiudvbcfbkjb\njryuwyprwczmcczi[vtijzvfbpssohcdgv]qizkalsooznmasljh[sdvwxkvydoikgjtomxh]ixzqpazdakfwczn[tyjorxvairghzrqi]aunhzwxnkjqryibre\nmlcynvuzmmcgoqkft[fkeqzbjanvjoieooecy]muvosxtjytdkhuh[gsdxscdehocmajsnhn]kvqitwpizpjwzmeb[kpnyyoozocsxurfl]obfvxcgoavxoiyy\ntunaljqogcgofeh[ivxhcnvflsbnmktk]akwwtuwpdpbnesmrklw\nhicudrdjoglrnongron[mxaxjxojmjgutxg]tbetamqqcheyjbpa[itozzzbcpnyerpth]brqcvektqfaxazdfivl\npdyuonakwvugssuduom[swhnhhzcbkrrpovuomy]ecfconssgftuhtwswfd[mjdgnwmncbjoxlinm]oklhmwptexymbgyfdaa\nhcxljuahgmiolty[kulhszpqyvsurma]xwknankkjfsieauadw[anajqqpwdkodeaagy]iupvtabiqsykmohiisl\nqruhviuomiixcoarv[idffbgdhamsshlinl]ygsinapdnmzvgit[xinvdhbqhbvqrjx]zdamlvlunjkkhof\nzyeynxvzdmmiybab[vhgjepcwqjbolwnft]aopzcryhnpswgmds[yynbcrcgegnrpsk]munxtddzxyvzwwcosq[igdwjifdopnhwzv]oyebiutkmraayzr\nonkgxvprjaynfipxeum[jjwmjcepwxbleahq]ofvhiwoyxmfnjbn\njdwjapulavrgiviora[vnwjfwpsfcdkhamtg]jqcgsuleganytwsm[qajmdsarjnocjpq]lxpalpkeehxjdslu\nmzyzoemluwoovah[bydwxptnmzqxdqfgdgk]hekhqzpgilidwvpey[ouhnrujqyhnlilh]qjarvqynycolakyiu[wzeffbptmwixrmr]bowqsnjgurjpkuc\njawvxlepzelbjymcke[atwksupwtnjjnkwe]xqqcmguandaqptp[yqsfhnssllituzzwa]xbgaqeuqtnclehgr\nxumjolgnaowjdoq[obqxrncwytcvrsa]tivvsxdntkrivblx[nfiworqsxjvwyki]nxnpoipcjqeeukx\nsvkoyidvkhkvock[htgrjltotuunrwka]uqyezwkltzsjtaysa[tqaaskeswcllblpnozj]yizblbkqgvblvqghvk\nlfqasqaubbgirmw[xxpjcwlwjsklklgyrk]fwckfwwekdgcesswh[xkcxlxtanadezjpva]naodeooepetabkh\nmtbhzeufmgeskqsp[deibjhufkntahso]oxebgcgzvpudozi\nepuzizxnxpmgjkabqfb[fmteazugbgjgozgsmhl]conlsruhnwdekaxf[zimnpzazgotaghhaq]gmkwnkivobskmeafcck\nepbvuluuhaazalp[dtsthsijbzgbvwzwgpo]blfatalfityajcpmyc[bbypikyeizyfntdt]tcnzahhiwutntyt\nvailqzvutssuxjy[llxrpxlpcojwmab]kqpqrpogogkpefajeuj[afzpfhjmpnestctyqz]mdggrbuuglbmweujgxl[qhheeepqrcbdfhlxoo]lxvrdwpugjperwt\nroreocnumcerxnrhr[ricaoyebqjpgzazssc]xzuqnzfgbrcvfnmpcgs\nuludakjsmsamkpmy[ropmbbvjvupftps]swngrcigiqzdkie[hjhbsazzxdxrseczxyi]pjymgjgdksaalxbav\nftvggoxgdteaxbrq[tifvvmwnraoiprgs]xopjvpddfjnbmcuxpu\nbuzursiffpqcwnlsl[plvkitdlxiyiotdk]anlvhgektgbpslsiai[gdgwwvjcdnywwguf]bydbjfxclhxyfgruke\nindbphvhghzxsuy[izgrijghgwhcooc]gkaqbcpwwiyfwmv[xxlzhbqmxquoawq]gbazvlthqbviupchz\nqofufmkbljfygwxym[egvtczslvioufuzsyk]uscakosnjpjbcrggach[gnyghyvmgirmwolh]rotkdpwevcsipnxjokp\njwaktcuuojllglwmr[dfntqdtznawzmzgwbj]gjykvnqmtzelkaus[eghpxrcnnhijhev]osfvouazhsijprtbtnm\nrqrtzzgqsnzzfntl[mrleyuyknyxyjhoibf]mwxfdxpeiyuhjcbdyi\nxgqwglrrdtupbjlmy[ayygnszmebgddghqg]hslqxsvijohmvklknkz\nsfqhncgimlzgjqs[vsudwekhrjuwjgig]fwkpceyrznigiwq\nbellebgmjpcruwv[njhctgeptjieourukf]sgybshminsxktqlfxr\nmpwnzwvblaseycnljze[qhrfygccokretvo]ydomrtoamoecceekrr[lgslvkhwnmsovxvhqhs]cbyuvbrusqqpvkmlhm[wrvxwjyyzsvxvxwpdq]amynjoncmemftlnqa\niniemtnmqwdmxvpicqn[drdrbflsylzhzltq]orjcjdsbzijkfwhdhz[mrfovzdsugacpyvlaj]azjikxjuaszxpapss\nynnxsnsrjdaqbbaa[lyifxbzcyzenzpzzulj]xejnjfbuykeojbeatvf[uhpeylmwgllqxtj]hirppxrtcuybulsuek[tzbdcyvsbmqtrzbakxj]kzpsdszfyuvgbtlksus\nujrrrtdxpyhlpcyxs[molsrkbbxoexpbqhnhx]aesumqacmujuchpxv[jlwaktyumxuiyvt]mmwjujsvuvxsxxmsfr\nuehksybnnztmczl[suqgywouppzavyoi]zbndcbjuexdgscb[cliuxzpullifofbhgy]kupndcjvxqiavpk[hqgafivwddbbepkvjj]lrqalseezuhjjbkese\ndjidmbcuqbjpfolm[cbbrttiwmetodejw]ghgnojuvsogrchwfp[qpikwfkqkfphshxbmxm]gsinzrkbzacyutlxso\nnvvjtnsnglopvcmna[opnjujeqmpgipfm]rudoacagklnjajjye[fqrtapichjqkhhf]zpkowfxfuoecvzq[juwjiqcolafbxzsw]fogkbzmrovqvbxbxeb\nixciqkqggdxskbso[wkjptmoonusnkzyadmx]tvbhebhhaqhopjbjqht\ngepgaafxcogfkyecgs[jdqmpkhjkqefzkwxglq]zfpkqukaelflilmzwph[fndatrnmtrwgbwpj]bndevgsiouveums[fqxvkjthzmyryobt]ywgqodizmhsymako\ngjlyyrwgrugaulnj[zwsmlmyahggpvugef]ppqrrbxasqowhwz[ngwudjmonpelxhubwnj]ucfcaicagnbvlboiwky\nlfckmicaonarlbnu[qnigowwaziwjlmf]ihypnqqozcilwpm\nxmtcgkcyfjppjwaa[jlzhrxmfyfjfmadttpo]vucnncbadihuewzn\nsviknjiphswrawyskzz[vlsdhjduekvalqgwy]qlvefwhnwmxrzgxq[dwnapnjsuiowoqjts]pnepuekbrlbsswijr\nfknvwkusyvzledp[qzplkidoxmvxrxcfs]jxdhirqylkerndfd[vlqmngoqxsbmljcle]rtwemwvqkpfwfri\ncujhxofpcjpskrgn[jxxgrxhgnutgsusruvy]dewdqleqewbqftd[nfjzhgvvqummwzhyd]yrccepfnpbehqei\ndmfygizbsbrtgnzam[xdnnacheufcqahvx]rxtljkenkwxgkhrwos[xnxicyqemngzgjp]slcfzksterjpmiz[okdqdoipoqwcoyfyamu]cmoedniphnfddoywbne\noafdrqypmxjzxbxutj[yzlsdipaswmgyay]xwllqynhfregxpwc[tjgxnibylfayarir]phswgvlkkfjjetrhdl[pkcutagssxligtwbd]xrvonaibaytcqnhgc\nivalpefzoxwoqycavx[wnrysytaesivblx]dblopqsupplgoom[vxtobrfntcvixltcb]kzktacrarmtwuhkcoin[eviwodeyddmsfkvhzue]drtrnlgrndrxgcp\naygkprnkwdzydlmww[firwrjxyrnqlvycccg]lcqurfdlcrvbzctz[cxzfxjybrqysasrppqr]domoafryutthljppcg\nuowwwiqusrqkpamdm[cppbcnmcxpecyoey]ndmdrcadjoukusxjfl\nmueapqgbxuyuttzaw[eojhbogjbfdbhyqjp]sxsjeclolvcjexxvxij[zugkiortijshaocu]mfayspauxoxdwkbj\nswusnwjcduzzhsjhykq[jhweoafdbntsmxcg]fwqrvlhlltfeygpcnyi[wzibgavydimypgdao]ocomuevbncyimhlbppq\nvzatvkicsxcmgcx[lembxneuonlldqupk]svfxiuungebjjgfre[ijwzrpepzkmvdwrjck]bhjiggmcfirhzyjljkd\nnlauzkixeqoldqwd[dwvmcwkqnwjlzqscj]hnnwnarbtuijzys[umpmhpnsrbypmpulhf]nijrnkqfvbyjfvgseaw\ngefcvkqyyecmnorr[unfzknqltdwwrejeix]quyfoemcjnbrarjuowo[znhhaogjluucobyvq]nozfnuqwkqrcbtwujxt\nkeerveohuokinft[vtganysszjzosaco]ufsxvtiyupbeddibmt[wrlgimiwaspamrdp]wdjcaxuqikgauum[jpwldupwbuuufjnx]tumqrmftbkrmohls\nrtgtdqksqxgvgxadbjy[uclopjtrzpccvdpjq]hiqaonacbzvgvigg[dirbsktzndttpzmtznz]laimumxqrcnhoitaokp\niqthbpkfocdhsvzje[jbxkmkvmrbnqjwlp]kycbbizaasoayspojv[iojspytksdfugqsqhvf]dlkjrsotrfugfft[zuzflpijcwgbioujw]tgyhlfclaxcsjnavdkh\nlmekqqiuknygtdo[ramnjnqzfihksfpoqsv]jhhvgphkjifxgap[dmpwxrhmhkwfsfgtn]mfzdjfhxmkrascd\nfywgfyehgheiqhbayw[ntuqlvjvldeyzokdepc]jrqpaluvezoujks[ijkurhccihukzuis]cljvkxweuvldevt\nudnphzgdlussuatatj[phfqqkmuhvlehlo]cyvspnwlrcmatbwoua\nlozehtimrottjudo[krocuifdrqwhsmm]uhauuuzfssimtfl[lyshrfrnvlueierymi]xogtepsflxfwcpau[nurlztguypvwjvoldsn]yxwnuqtvewgmlbfj\nqkioxzfrxxwbcddg[iecvjowpxnrevqrhl]qxpciafqndxasahsvoo[adfpiuoapzqsasajd]lduzndmefgsvzzdpmcg\nklfxwvnampkmmqjmfc[pcaeswcdleyweirmxpv]jnwkgamdjeoakjcnuep[hjwzdndjlvqfzkarwk]ewwgtcnyjuczgmyif[eaaehzgwbkdfbcgbz]eeioocxrjsulyuj\neptlgbashiewmonaaal[ohtsrundioavfrouii]aydjhcanascnanbfzvd\nikhfkzncdqyitenbg[ldqqsrhumdmiraztslw]aydpjfypxqllkevec[aponlfgxnzgcaddwt]yxlzqyhbilnsgjen[dwdrsgergyrzumtlpvd]srlqivkdhbdbevnq\nxpjwxwgiyzqfwajto[msisxrvzebbtxiv]zkuujbuznilsymuuxq\nvkmqsygowhcqzdxlslt[fnaztaplxaputnm]ykkslsosxwczlrwbpmc[orlhcrbdjuujhaj]odtfvozkxuwqdpsm\nqqxdpjpmujaveczctbz[gulkmdfhbgvyxuyd]jtxafmzqwqxauaxjt[jgfnrwhgdtkwdfgt]unidfciwdvpazpgfa\nlfcczmpjpqgqonvcvb[iflurylkaiuflxp]dbepqquyeagxsmrhbwr[vjjohmujkozstni]suvejhnfwknjusxgxwr[wkjnfmxxzwulujmw]qyawlzkyazbwftlw\nuwmrxdaxrlsvujdjrm[dmdnqcmdmnmnhhwicwk]uowycyvqvjwrjgtpfqu\nzbxlifyzwnwujvs[pyyyjxylpmpwgbh]iutvnonqqqtbxisfopf[qevehnvgqgkyfuqr]mqrcuibiihlwdrzd\nrxlnsbgsuofdjgifrnu[eougczwqhpbyqjpo]rokdsivylwcqepdyhfp\nyhzwpokjwnqbwtsxuh[ekjrlmzyakgkzlemnxp]gbktdprzdyhcifmigxt\newjfrgfxriqmbvczdtw[wlbdrngfgnwdvkt]vxgbaaggmwndxlms[vupgwxfgfpxtnen]kfeekrdualqqnril\nawkkejmtiopfrqfasgn[alciuobkmtbxngulv]qlowmadlrlapsquuhw[hhtlyfkusvlwunbbjod]seacetmksrrodjqdffk[aunntgaemlyoabfgpf]yrlrzbdjfejbmskdtrz\nuegpnmuaxvvpcsuzi[pxcbpsgaecuqyhvov]oiyjoyraxkymelqg\nffpelsnrffyfzzfdb[ymtulkndbgguyivf]uauzvyseztbkdvxow\nomolchhfvuuzzbodx[zhvhxrqwbdhfwlnn]wyyrsjfjsfyafjfpoe\npuihcjkezjyjjfl[cornhtqjyqlebvqyl]dbemzlxolqxpzoi[qeihkchqoewcabbwog]rlfloutfwlcjywygd[glqjydslofkcstjxd]oxcycaaadlnxfkl\nhbxhlyelfyszkzyc[cdxcsyocdiifefpytl]wxefesokgwwvcrp\nvdqcqggyjstyefs[yiskvcmdlbyuwzdom]cwmntthjhfyzlus[dpoubuwkbwrkpfvlgf]zryvvtowakcyclcg\nkcpbllbamycbuynia[duyxsbzyzibjwejygq]mszplxmgtkqorlklg[kkbpzdcqtwkteqfpm]nvgoipyzmaxtizqkxk[dkjpvseaxvosmsh]ourguqaabxzzovsn\novojqexhiiwdqunfvpy[ijzonrwpmtbftrqgs]zkmuxgcckijagmj[oygvczrrilsowmxrcwq]jpwamodaidqrzmal[yglvklzzljuqykuxte]cifhyowckekufubnmu\nhqsemgdtjpiikngtrd[bqryvzqcejlkziqbeg]gycysifcawyjyeu\ntgdpvbxtvxlyqvouu[xqefdugumgqctwvihz]yxymyatxjpknmpb\nmghmbjssqzjlzlg[kilmyfmenoqjnmwg]hzuujufmwyperhvdl\nieqarqlveeycgazb[azjmtbkbixtazbcv]xroiknhtlbefpgh[xnhgnpluemfqqkxg]okbkpxswfoikufwzazc\nphtjaokeiocojxb[snjwozbjnpwckhr]cjwsbiopkgqjjaz[rxkobmvupvjvobifvx]edubeedqalxklpb[nyfuqcxwtynmofmfg]zwdaaonmcoczxvfr\nfddrwtloipcoigpruvm[nmnolrurottdlkhfwzy]dzztqofiytbyhhzwsy[ovdmmhigvmzuuji]jirdnbaefkkdpgi[orlijsvzupzadsvi]mnmwussnnikjigkkr\ngspafobrohvirgeaxdq[igehxnlnjtwfcuc]aeibhshuiyekgcymyty[xhoayxpksnfvdzjwh]ktkoteqwnsouvwcftyu[eqfnhshsnakdnxwonzz]wwfzvzaupuirropirue\nbpyvotpfgrefzidpn[pyvnycicdpcutcayrv]twcjgpggepbtnute[fdumsgxervdixwv]ydccutccndbxxfjrxh\nokzxxrtdrfviychsj[ymguzlptohblvsj]ofquaojgbjuxhkrm[ingfugdcfpjtyoj]xwplthdujgksrosmv\njbwwuuqkuwrrzxmuwh[hxqptnyqwndsntckqex]mgmaotcyybmuihu\nrojskmdnydeouqz[cdmuavkcabowcozhe]znwaohorcanpbyhjii[gkpcxjhxnhligil]qbzwurxyzdakgsnwvh[ettfivzqkrrenpxmsj]dfbcrgpjbivcpcpcoqr\niztjhisgpskdgwxwfdq[avnaibsrkfmlavnyuce]innbnunmtkplvdhq[lxexsvmjqjzpswjyrju]adcnelughetzceb[cmafkyaouzplrel]iqhabfxgwxdrqojp\nmcxijhkidamijcggv[buvpvujncpcwxvvt]xortwrcnebozerevim[ylisqiexudovelmczm]sophxrbvffupehspu\ntdbjhtyvoiflmgdt[lbwyayxikccooiw]rbhpfinzxpaayibe[twvandevzmehmiiot]npuymvedotdclzovsq\njtfyyycvwwukxvfbpq[acoshjowooeituuy]xicaiqqcrtpkwtu[lnnokqhsagantfsyl]kchtjwkppjyxtwjh\nvfzsxxvmxhdpjrlm[wpzhdncopnapfijmlcr]lqhsravxxgptgjs[wwyuluteptkhznh]tthklcbbtbvhauug[nfplnscrhldnwtdyzqe]ockiyqmpnksijbf\ndlnpcnognelscok[ibbeqsbqltfskgcgqb]htrpytqxmucqlnane[vtltdgsfjrwohtc]sbykausqnffmqkv\nkxnaikbdqxcponrlivi[pxltpufeegjrawwanax]apuwyiawecyuqhgjc[vtenugjmwgebqzdt]jpstgvxeivppyaqwdbh\nbjnvrqvazthxmzqe[vhhndcvzvvtdjpu]xvyoyqrjtbnonsstb\nrglwwateiuipzihomf[rvlceqfsjsdeajp]umwquiuviykogvs[nyxtxtkhyplexemcvjk]kgqhfvraxxybvapgs\njfhopiiqntjmgdsj[lrijxadhlagitvp]uiwltkpdmqcvklmj[celhtexfpelokeyl]jucghcilfpxmuhsxlj[lnzbuosgycapkcujcsq]uipyywsuzrkxcxma\nzbczjtvnmirbqohanm[bssrqrthbgrtjlfdeyh]sajloorydqhdlpfx[twqasimfthlutzbvc]xdyjyaewqxknvdz[exppwmacezbuavlhe]cldjcsqujgldchzigys\nxvhlvnfixnvekmxfzr[mnmpxowwvahbtuiltn]facqroxwyyelgbeupk[liawlvgwyfizmas]yxgndlsxircarikrb\nyjisbltbmhloiojwzy[uiqmflerfnevkzvnfmy]kecwgynuudxejjvth[joscliommzmbkqcqa]pwypdesmkawikue\nhsiwncahwnipmmjwspf[icngtprynzjdnsgmh]htclvcobutyrczggpic[saypixczichbjeve]jmpwkwrnvhjcpglrul\naagdbakqyfriiolq[cjlhszgovtyhykgikl]excahvgfswdnpezh[typkmvlnkgjkmherbx]zuhrtvvwvcvhuzalde\nqdunnnxbbpkljlj[opuhjxcwbtvnyzd]gqsaxqcmgmnagnim[sbbkqokcljlriqvwlj]vvgscumyxkrpmyrwz\ndrtuyztubzingcdvpy[ichljckfcgomhcfah]wpkgosokfjvzabii[gufmzunfeecjsbgg]pbtuedlavgbxdqq[vbbhreveuzdzbjygt]kglhdfghynsujkvnug\niccedgowicdllievwww[jrxauxixbmexkgfvvz]fysjaucelduzrxp[kubsdwfsoejcskemvl]wszejdloyalatpjq\noujirnbrjgnlqaksps[lphfkzalpspyhuxf]kuscphbgysuwhwyhot\nvwpxodocwmfhzkhyf[srbxugrfpcalangfdj]bopxssvinpngkthdqyw[vkkyaqsjhizvounptrb]iiwhyeuatcqnojoidrn[xiuphhwusooiewosd]gggtfejwtpburzqyr\nysoiymdfphxmwlmlbm[nudcbwwqdfabqxc]adsnqcsxmpxwrhdwp[kullnmgtapmantsqr]ykmzsizznrmofzmy[cxnrxafdhfprlarkd]pffnyurmoaxrpvd\npouuuowcgcsgvuznt[wvbnsxurcwwxhkpdg]oncpjgpynhzxyvi\nvlyfxbogdlwgzbuy[bkgdkemihxctcppam]ckevcpesenqjadifwz[smxfhxaidkueomhxyc]qwokiceophbpdyjovvy[tmzeqvagzhvviakrh]hionrvofdutctqdb\nupsxlrmcnqiikdzhlcy[hehttqfmtzwgrmxfo]irippmddtqadjgytw[zkxutgforgpenbx]coziqjvbhjetosrtek\noewwtzgqsoedpidbn[rjmmegjghjfposhp]tgddsmuqxnvfpopcg[iwwvjgzvbmkhcmlhm]teygdquxhyhkrtiyjse[sknqnxtiutqtavvf]bcqiwxuliuhpeto\npdejprrltzgdddqhod[jgwgzdgvdopqgknwbqt]jaxeauvefzuvvgxlid[fpahofmhzzirjuw]enbiyknxsjhuxzx[bicvtjwkkhelcgebywj]ldvpqmpgzvihjkejl\noazlgrzhvtekbje[rcnbajbbtikrfapsnuh]gtddpwaqibjnpmfhp[zxarpxagmnzespusnm]svtfacsjwezouqnyfa[ujbucyylrrvuijybde]bgumlrbysgompdeo\neyescsulrvrxyngf[wpzojptmtmqywwvdz]oicscctycvplkhsb\necwhdlfufxxytti[tjpmriwkymqufurtux]kvcdcihmfxydmxb\ntmlzauuiszcwimcvli[vnvyjnebqbpoaotvcre]eupqvhojcmoweveps[cmjkegzrkspdwmdyuo]rjcxvzssaopikbi\nwmgjjrccewrspnkcdg[kqagiunuhskruqpsmql]histajgekuklfzmu[caldsteatfkgwqogjb]hwweftyntccwfmw\nlvwovmvymkxwcvuvuov[sxedhxpfwkndxgtwn]jnpctsvjkqsybbfy[coophwmyxhbhjjzvf]applfppvbrejnvz[ipytgyblyicrnet]ogktxhleyrrhjwqqt\nxuiednrxcdyejmgcsg[mlmhqtzingaekkj]xmvjiydsuffmteb\nzyweldtmlathqbd[zsskrkndiopdfqocigx]mpflfwtncuwjcnnvhf\nchmlgfccuyimavif[kpgcuavqzwvekmahgxu]zrrkiipozbierayt[ooxqyjdkmmuaonht]qhifgfwmnavhlgnz[cnbosuyqrbqiuye]ksvsrroennhnxup\nagxsrnpuwtpthaijwgi[fhyxwctpsxqkkypdfie]craulpcmyeifxluxu[yypagmcumxjcraxnvpz]zdgmbgteapcjwwzaive[rowspqgmcvqudjxm]qydbkwdeuraznvzzno\nrhlhblmxdccpvudu[jhbawwnkolhlfssiw]rahopqrzbhdivhkrl[sdyjjbmlxlpcfabw]olocfasvuwqfxbbynn\nxzbhnrzyvfvbrodi[kikpaqjccdhwfmjps]tqeliktvbjjnbpxwtq[jqjvumyqcjodqippp]ufaxyqyvdhjxccwbsfe[pxiqyqpvccnocmbinr]fqjralzkdemnowygd\nlvbihonzfclpqyijtk[tzokuoeriylwwjahfud]vqbyrpbchllhsmeodxl[ktbdicmiebbpuxnyi]guxcypoxyjhshqgshs\nnnmyoxtukxhrsgt[ecovrntpmkcaekonw]ncfzdxdlawbwtxqpkik[fkkkkxidubuatpihcnc]wqxmtvyakouvijt[tjvyhgempiufanh]bcibhdmbmbmmbyyi\njjyiltmpfvlkclthbz[icijdepekvlffegr]xnmbqmdiaskvieeudt[clfecicrgtuxodur]kqcqrnvwfdhpibndt[xsieatgypudmiedmfo]eqaouqptjuohpzbxml\nwaqqyhmfacfjbfasug[mbghdrtwrqihjje]jczikhpsasvutpmb[obwkagptmpwgjbhev]ozwfarybcfhihoku\ntocybmyipesjprx[jdsdjyflopvltwsccxe]esswfgrsjawbduxuu\nqwdwzgezyklxtmnd[uikylllxmtfhnwh]dmozabuomdvhcoz\ntffooggeeufibvgyy[walfmmmfaegxaua]woxfjealuwsjajkk\naipayrjoievpqkqcb[pcnirwsnebqijke]ocpwinpdigoxudcksgx[vvuxytomiqmmacndtk]lkwmarnwqvzulsxofid\njwrefdombiesxvvap[fwhhajyhfaqzgym]gersxvbwsbqezoxcg[iaetgujgempehiaxx]llbgjukufbvdfxvjs\nhexdafengwxaarjkqhe[brxnqkfcyltwlxc]tfqwhqspdfcgajfzlak[shtfaywffbchkkk]txpanajvkwazozn[jzfxmgozivlbctstlz]paxycypplmjazycksx\nrwttdrhdouzvmhalwc[ozryzmmhwztywhuif]favxmwzmgawjdmcho\nsndufqsbyhdkyathrxm[spluzodshkuiqhrm]gwctupgaumdalep[urynlbtsukjumpcrgar]mvgkstgtaxmtiufho\nmiypgghnpfhpcndife[uogotzsxnulstsucja]wrdogybnlkagqdtv[uerlwvvqvxrvtsaycg]bxpngxvmakjdvvdqfed\nhgcyvldphesdmdma[inomdckqkhupvxmc]avlnivtukipmdmts\nvgjaofvwaodncajhg[wmqzkrqiwbxdfsgdc]uzsywyzfptypsbto[lwfowjvhczggllfrw]nwchgcixmkxheceuq[eanuozoreimfpjooin]btyiwwfizhdbpfazpjx\nldsqkerydfisskoimys[ltqspskmalvyujfyrqt]dtyknopltmnvdtc\nekrdpdzvkoxfkjfpx[dpskecmtgjtwkhi]nidanbsojuexjgife[pgpitenqczwzafdad]mfcmnjodtkvhbknfto[uutgojscjiffmofegr]rwirhlyejxezndbs\nmhsngxyweukngbybc[uiapxfrpfptauhiw]ruywrhlzekcudjgkw\nurxtzdmrfedalnuuha[ioeyevidklsxpqkaahw]jhcrcdzwljhnudk[dfvcwbualikbxihqg]rhhwlhcfpbkexewpgn[gkgaygbsxboxypxbq]trsaulacafchpndootk\njmlhqgixgtfbcxyt[vhwpsfjufpbampqyqa]wwzszedhhdmztex\nexilqpohtavxypsco[wtjdsrkpmulcraoaooz]ozlzxumlxhyyvcg[btpzjjbgjlydtfq]suniwwnwobellpbwd\nglgwpqmljnfxjwsgae[hdnpgizkkafrkqfalpg]pskoghwqhabbrazqtgu[howksatecaqyemgxpye]bvrcfhawviubspmkeon[qciouynjddffdlp]kruofqzvhiaqbtm\nekyqqslkiuaxpucbsj[nsltoiyaeyfkygmtaul]eryfelvxmeekndddu[waprjreciavpzzsj]cppczdrntzrrqpk\ndraegnpszalplun[jwpjzjfpanpyqcxnu]lddilnitonnehft\nafwslsdmylslwvekv[ngnsirjimcteduhmbia]utirtwchbjinjtkp[xtdywavaenpcexfi]fsxuipobvivhpowgioh\nzpjzyqnadncjcbgulq[wtwvealiuqmxtmgbsu]wyjqglyafposcrwxue[xqmgfmbrcdcjfmazd]hjcjhoqisrvxdtiefm\nnlchdiedtvmvrwq[aeqiwviurvdlsaxzdy]vrjrsalrqznvzhwxpjv[ghsoysknlxlzbqjv]cwklpwafgddnupknr\nzxqjiqwrswpnotkjm[vdlwfpqexfvgzxjbsdl]avnrytuqubaojek\noklkhatqbeccsctaq[jfvcdwlampkhgkjw]hwnefdbhaixemttbk[xbnquvzqozdzbntm]rpyliiqlbmravsu\ndazldpxyqjgbihafnl[udnqydjynzfllmxayne]oasevmgbxuvgxtmurus[alpxiujmrobllilgb]rrgekfumvabcjzmh\nzoojpgbyojsophrflji[bobvppelwuyynrwinzj]kfsldwgeqtbvtsfy[icdvpxikjxhdaipte]kxyxztmtqiksvidn\nensxpontjxipkckasr[bdikuxubzmiuhsb]rffefjgowtxzjltz\nsuqgbqjkbymetile[jmgtojqeprpffkogv]pnffnorgbyrwddlm[pozvbivhruebmmjwogs]fuleotnbbnpuqre\nyjwcijeeaqhjdmu[emqntgsefvphvpc]hddshsiudkvrzghal[aieudiuufjmtihwli]bbytteummcluoygddky[fbkfhkdwubnigzvl]phfapgcqrshmwis\nfbqpgkdmhvtjmkepui[harjpumdzotcylumk]fglgadntxizpjsy\niforzbbzeepoddbalyb[cutsqxklmoljnexuaxo]ajmokylzrakmmlxcub[rximbemhrndnogfzf]pokqtdgeipqlswvrim\numtkjkgoyutnxym[nizqgpcfftiydbqutr]rzgvklegcqnetqkg\nzdykayyaybkihcyc[qgmrngcbixqqdbvx]hcicjeavoycywax[bkjnxvfknauougpe]xjfsxnxlgixldzb[thjemtygmoazibfsar]qzdtbduakjdqteckq\ndwwceyrsaqrhiadehmw[bushvhvxdeznysxjr]hnrekmeoxifqrsq[ynfaykimagehxbcxhka]ucdpjqxgcyyhvhobmdj[ywcjwcveqtzgqkzx]poruhxqfxuyhgqog\nmcxpgupgbiznbdjjfzn[nxackwalqammtynl]qnrwciginnlyfxiyiv[hvovgilkgigolcolf]fyqfptzmgmzbgkh\nkwzvwimdnfngglsqk[tvhytletnpwmogdq]zjndivdpftqyecxhnyi[iiqioqsyphxjxdy]diyppzzxximnlgyhzh[ylyboefbsjwjkkxbar]fuvxtvpoyomnkwjwsg\nvlcyiigmifwxnvcdw[enlnmvlfghlbwib]lwsaxkcpgluzkmx[kglnyaprvaagswvfg]vvdeqkfdrjeqhfp[fcqxurkfmmorcenve]copdpqayaaolcox\nrxjfsazvypysbra[pwnsoibariykvjgubu]nyuqsygdavnxfakwlm\nkkgyhdbiwyexyhxgd[aigctwltgdrvyxbs]xypkkzuhuzpxygupvcz[lwjjxozwzniiywpv]koyfescfdlnyzhcgxin\ncmgqspcojjombguppb[atincfnafdmbhtgzk]bidgxkkmgvgbeilvk\nfphcdhkhetqucchmtm[ieoeogxnvdaxsayhc]xeigwycormzmwgf[cllkxjnlkjdinvouy]ammsmdyoyvlpldkgy\npjewtnwxajalxzrw[sreuxtjgiwxqmsfkj]nghqriebzmyhgcgoks\ntrtaefztlkjjzbxpip[fgpnmiewbmzvqfxoikc]wpemgpznkrerwlgr[ptjdchwakbcdmrjwxnf]unaxvqinaglgfeoi[ekfifzrybpfkjiehpsi]bxkuqrbzgfctzult\noyuobptvcbpmiiw[fhefjfnvmrpohae]uykwxrtssawavbuk[cyabwfmaxwqgmudcmpx]vahdtwpzvebiypwjvq[twtyrryywtwsckmff]vkmzcehpgydnorxo\ndbgblaadftjartioq[avryclynyjmceujmy]nsqtusikmlamzfht[qmvmgeprwbsokvbzmmc]ddeuxmektypsukme[gqzmpenqiqlihjqoceh]fmsjcayltvsxycmzv\nixacedvqlzvneoqus[zmgeugtrxuidpdtzzn]besixpupznfgvqelwxq\nausrpqkpblrplbq[pzqlirofwbtvjvoua]yljvwgnjvjehsyjd\ndmreexcoqmzxelfjeib[zaghgfbihozktuebhb]vdwkqxzetddhhbhhyd[smjdjtmnswvdeuyt]noyncdtfrtokngqld\nakpixaofgmscjdmr[oiothmxmcgwvxmx]yjiwdlhqlrqerce\ndeyrfnzcctnmwjagql[qgcmtvfvpvvdminuwa]tynjoikfebqrxgvyehu[qhyenmsqmxshkvcmohh]llpblusdcqfywcdq[ikngnvowhnvaiwno]ixndafincaxkyqwimq\nrjcoodvjnnbhxnlo[spesoflcmfcoifzosgs]qauqixapgyfzvtjbpee[zzxomezynqnoeue]xpiblpyghkxfueapcm[qotnfesblvvyrnsu]keguppozqkwfxlf\njgrowursqweqfwxbg[rfyvmzbkacqjzooslnr]znoeuzryfguydetugz[ssotfccqiuilzfuexd]zqatqqmmdnuiicv[mkijjomihqrtuiuobl]erhrjzotwvvpqek\nunyrjnckltxyfxyj[vdlbfpobsnokudzqab]dhhsatcnsuifpwsqe\niscfknfmwdnipkvxcma[shkdzhzbrpdpacel]nrbkhvxfyoslwfhkldm\npoxfvymkfzuhovx[wyjhfwnozjdghzuenkx]tpldycstgwuagjrz\ntaqbysrkuxvxncweld[vquzvmysufavywl]irixymrfapfwvnorzx[wznvlqeltnvzjhd]wgpdkhhoypflubfznpa\nveeytotjubsezxvh[mlbakwdftkyfbpid]qehdyxzxctrdvvmpil[cfnhvbvjkuqwyzgie]wxbvbxibaqoefhzkimu[vcdhqkaxllbdmbuxowp]ifrawmsqulaizxxqytk\npbwglxgdiijskqrksnc[xryasmfvaqakaovslr]wslyywaninmrddik[uhieoolqnqxdmmltpyp]sgjoghttawugzcwzstd[zwhohshbhultyyoti]anvjcthgqapmftxhe\nwmqxexytqfmdfgzkw[gbjexhyoufthdghiibi]ejhfohkfsaixzvtx\nmsrjuadzrxxolmxfxq[slurgkvzzfgqpnwdhxg]mhvtwtqplrxzvrmwtw\nvzrfylnagvwqrbukxkt[wofldsbvtgzqsfxbl]scrfvyjrwyqmrsbot[bngltozaybaghfij]msdphikahbxebdar\ncqpwfhfmgioybwsq[judebliwtcirgrtjcs]zrprctntnwcrszilkws[qwoaitshrtavmpse]zubuyfygpgdycnytnt[ctkvsrkjluwdqeeyku]ksncsilzwvkwtmn\nlwtwlwmtqtjqiym[nxfgdevoxcdimcnb]koarjfajilpityyhmbc[emidtlwzhvfmrpqbhik]gsefmkukbjyhgdclj\nfesirdkrgznhplitqo[erpgpujpndzzaho]wqzethjbporhxokift[rwelvzaswcwwstny]xgqpqjlcukivddrlv\nzozyeoozrjrbdccroq[pffesupjavtnanbmhae]gatiaxphiwsrnnwloj[viampjpkjyrhypjmto]vsqwksazgcaggsv\nfycnqvxfihmjnkjogf[jjxnxjolrlkbcqp]pdqtmmxyrfzpbbdm[fdaejpjrasjphazkc]hntqbpjeliiqmtne\nyeounyqfhbnbmjc[mzbietsligfkult]bywnnvpavyhinsm[xuwaqmeiaffetkpkvoq]ufmjhazqnhdmqyecja[ztqflfgjsoqybaf]pjnbnrsnmfrgqamxb\nycyxnmxnttqiqnsnmi[wkrtuoeddszbizysqv]yzbksxesoscmlzquqfp[unqyazgxjzdgvhjylfd]kunijisskcelgtxzp[ciyxcpyyefoyhqm]eoqszchkgdhttjn\nevecetgcdniectsnadi[skxzpvvuabkudplm]zqykqoduyjvgssjin[uyojccqmnfbztpdnwvs]uzysyjyjvowlsvpqa\ncqkietrmjexdkqb[rhubbesuoeclwmtakqe]ivdnvnndssfznwmhbrk[zmjmfprnnowiedabycu]rmgmbgvihdcuzarhbum\nzdhjklxbktkqeglhts[iqagcckadjftptawh]ezdtjbiebkjvivekdzt[gwehifbjyqnazsgzziv]fhdnwvcwnamqdaeb[rgxvlygqlocpfgqfpd]kkssrbltmsamrpiedjw\njlttcsywphepmcike[kufzshdcbvfvkwsahfu]ioqzvlzvjqnavymv\ncfyvaasepjmgtofy[hhoqwyrkhuweoetwtir]fvpxylsiwyinialjsg[hqahlwsskotrjlid]azfumcjerwanpukap[iqjcxdwtvmvjkoukcvq]koeodiiywozmrtktxur\nllaevsbyxpkahrii[dxfpfzvxwpzedtvhtlx]corhjnbybhlahvogj[aeukoetmokgjlswve]iwamrxgeszbcnzsxy\nabxkqpiyavrfgxjbmx[uqzsbujxbmrjyxf]dsiktkwxjovhabuir[baqaipezkcvfjyqc]svvyuknankhxlttwng[kwsoccnvjnctnxa]zgnsnelphgyhfolihu\noquaqiwlkhwwfxnox[rifozvbwcclekccqk]mmmgicxioqwhlvjpsu[tndpmsoarmdojex]spywovxndxncbpshb[rgceaghxxvddklc]osijkijuctxjhtbv\newucowyzjaqacfu[hruhcyudsttblexjwy]mjxsgzalkyasstkuzi[drnyfhqgaemafei]uuimofkacnittaoorr\nnyzetoiyaqbsxum[jowknmpjwqdutjlfwo]oalwqxqoyovfjriwb[lvwabzjorjiiemeaacg]znsbvpusrratzywwwyk\nlsjzqfxbbuihsdx[akccvjqdtzmxywakf]fkxrqzurzmqusrx[wmkamfvugczykevpq]avcvjbiwezkocfvo\nohoszcqvqivamuaisf[lyyacjpyelrsgafmyl]icwpankirjvekeg\nkruylpszzrkzbfxbmk[thxwtofeyjsijenmom]gjblnnkhejpqdomos[xjfzkxpgfltzzfdby]fnbkcvyhwtwmvpykj\ndtqrdvxfjedeydhdsz[depsrsktdbsiwudc]unbdedwnchjgetnwf[bhojevqkvcgacid]jmyzzhyslvuhnaizc\ndwlyvffagjfzbevant[baalozybgljljwj]jomnxqrlanqrkcjds\nkjdsccouzjkqxgicub[ghhfptkxbsgatseoxgz]jiqgnfilkycyuvlwbid\nsxbgpazgvlipytzq[fixpxpdcuetwlqprcs]qcvdieujpvhwveur\ngerfcffcrfrwvsjw[ypgmjuvhhzvvavtyulf]cjhqxizulglhcvy[mpjpctaxpnlrfhalp]wmhafecpyzjuagisv[aumyqoujcjkxusu]skhuivrgveucfrfzb\nrqkibcopsltsjwq[gmnenbrlgqtvqflnt]xuczjcgsxmtbmeaysdk[rkjjglznqblxednxx]npiikosjigixuvlnzes[vqdtacxnqagckmz]bnrzgyqhejnbmtqa\nekzqugvzksupljx[hsjwrqxwwgcdhqhhzo]cqnomxxbemqmhqnnw[udcfrvgkcibabyssusn]zfuxkqiwlbbhssd[pfvscossyfdhjyed]zlwsqyhygkdgfah\nuhfxysjbqxaerhsanh[zyuotxgmbwkahzyevkq]dricwyfpfffhxncjn\ncmccqegbarzixhqucrl[ztgvmqmqpjtfgfuqjjj]ubawaltzbmhdhqioav[sszfycahkeptflx]otogjwoazgidspib\nfgfdvktoaiucefhets[qwjumhonvmtimauqsy]zkzorsvmedrlycqel[caaejbjnvlaqlqonk]ndndrqbsaaweqoyi[ovnpneqkmsbqsav]cepurdlgjkedaaeo\nnfhaistnlhzethu[gyozecvbgbkutaiuiiy]vbmcwkesewbbcdvw[zxgnhhbnldllaacb]kbtgbqxtmqtatjc\nnuxiknpvosedexey[gfixiukjvovooybkr]nkprytbsajposdjcv[ahjzndfqmisqonz]kzybggzczcwhlnrerfd\npuxghpwmypdrhykyd[xioiypketoaohdxa]lybkoxvoraessmzzztd\nqwlzyfwnqvxylbttyy[idtjcszoblpujfkf]nbwtcwowujbgzsz[mqckgqkhmbzpwtuekcf]xyquvnuptbiwlqdn[gwgdvbsouphvvovkg]buqxksahwsgvruovojo\nnvjqtzkgoenxnismrq[mxybkgtvioipfjecdma]wtgqwbkpqfepskvvay[qqxflmtbhprambdu]iqtqqujmqrlzpdwbljh[cmdesejkyvjzwhevg]qkclggetgpamrach\nntxnwuudhhghcgd[rlyqxrlsbpsdrdlls]qfzxlyrfjeshhmsyz\nrxgpjhpklloihtpptpy[pcbbsflfkrknahkeq]uljnjuavjkhklwwcm\nbyxqwjjdyqqsdnt[nkxqnfrxqqjtwsnpj]xstdzfnmxpkyszg[yswyxmgmqsrvaxdkx]sjfpeyrrswxgeflbncz[likexnumjhlodzimm]crnvrjyaumqgmjmy\nskwhvjyhmosrbbziiaw[dbztswjofjvkcbjtapg]yrzwevkwnjjefwzl[ifwifdeiaqpvuyiidrz]kqnqtbvgpxkejxvf[ubyvhimnnmhkbbnbu]zsqpbztopdvjzbpj\njttcdvuuyawsjnode[ahfzcsoxjswcdysclk]ubdipqyzzhafcdusjuf[wtsiychncfnaztdn]teqnxwryvsfwqbbw\ngsoacpemvpypmizazb[rzluiccnkviutvg]bxmhsnyomypyueyhqbo[mzxxtfjifzluckdypta]qlirsetsxpkgewemam\ncdqotetervrpkaiz[tohfcmgrtozdfduhk]mlgpfaviqgvzicff[snphhquukvzrgqynfqi]eredworrsugqqqowk[fvcdlekaqtuqhhchh]hhrerrbpzzarqnxiwwk\neitniklfnvnilfttm[qduauheufxnjowyar]oxizltxvldookdlomn[igmwlbhxgszcvhshy]knibbdqqnftzglqjodl\nibypwndwhrbzbowoa[wyrgxqcbqoqayqkf]rlnhzutwptjhfwrsme[cfpmzztsrhtdcgy]tdvricsznenkyphwzt\norvqewlxihoswvwlx[ifiaqweqqmaeasrkvxt]icmqkogypgrbjoij[qnkooyxicmbjhormbu]wkpucublpyqfkpjewzd\nlzshelyjacfkrkykwe[jehbtylsskmnxigkrh]wgnozoomyzpbyrytrme[uwcvshtsdstibykyrnm]nykxibwjjcaacgg\nfgdrabfqaogxyvpqfgs[bandjgjgkuuuxfuh]wwxxsusuuiezkvojziu[jsprwhpeictwield]tbpmjxfilclfrqx[zdmxvurgzzrompujt]ausuaokslerjqiveplk\njyhxxfrgrdjjsorsgu[uxzaififwgjnklvj]uehxdiantcneqrxeqi[nigrgktauzcpyazs]fjyinlukaspltshmhlh[mfvrnccglqfrdbk]qrmbqjtcccjrsrdmgs\nnltgngsggdruwrahzhq[gvjujsgoyasfqql]btwmnkkccdcvuyniu[tsqzwyypufxxjhd]dvqickfwnoqtrhokrud[qjhdfcdcsfvdgkotq]hndylujuuecvakzmrp\nxyvhcwkqkedbjzarfht[njkseezhzjrbujcdjs]obghjeljjsjksswil[mhfukqardbaypasf]wjcerxswmwvghjortxs[ghqmhxisgehdsyb]ysvgpyswsdfkomanrtp\nwdwmhahsrdjogceb[jdwdpxaeemsjficjz]qqysutatflhmanx\ncpctsiwpwyifqkk[eebyeqlgxyvaskcoda]sjayfoyavfkaydph[aztkadhyekpqtys]jwzqgyewxxkbisw[gvlxjstngthhsjeybv]ponztgpuhfsndjb\nfawvrgcdqdidogtfu[yidikecuyabulhiia]fxfmgcpdbdzdsfkm\nyjateqpywpcjcbo[xddnertejcjeedjulw]humaqnneeeynnpp\njutrwhvpaknrwoxp[ajhencapzncoyszy]qyhbpivdpqjeebsirf[lbsqceuykthorgpk]olrdkqyikfzrdzi[bmqrmgcmvqcgaxosaho]dkejbjzuzvyypxz\nrhsdxnktvyiully[nciwcjzdccerinfkgi]czljhsizretcfuea[gudarsiefwzfdvfqsip]tedaanrqtnfjdvgm\ngrkgawgbvajxlbmbgwm[dpfpvpbrcwxethiu]rpfkykrvmatjwkd\ndaemahshxyowxgjuio[dwhknewdrwoxbgk]vggqgdzpypjshps[arwnnbysrmyfijttrh]mwuwdtpqmiqgfkntqm\nljpbbzgdgfqmvis[zqmfyouebpfvuscncay]omiockdgdxibtmyfwsk\npirgefjkoicryrcgu[qxkwrjfuhqmjzzmbc]jrofqkmdftjbupytg[mywqavlapyesbfea]trqscgjokafiarh\nqsycbrrefosycpzj[guklennkilcmomyngzq]numvvwtbyvtfarlt[frfzzodqottlwzj]qumundqekohrpin[rsxaymghybsvzymhac]wkmbavpbqtoewxruut\nerpqoualxstxkzkwgf[spsetkclioxmkpobkij]mocioemqrazrpexy\nryeoamcyfewnjlbdfsu[mmelohdonphatmxblhd]wgkjtelxmbwunvaxfne[xgohvvrmkweaabsd]dkukcrasqoceqjyehjs\nzkmkqzphahjdzwot[objfpvwrjdcdxinuvi]goabmmhuvavbjgebdow[jbqupsngpnuoubvn]xofdcclnjyfofxnzyvk[mkmshdjabucvgpkteh]kqxuwhyogoxhgwqyyvf\nyqlzjzpztzgtpomj[qcmfrvyamtxxtcv]hupfwqhpdvdwfvu[edoxxlncqxfxpsls]iyflxxkaztzxodxfd[xavxxfdkzquifiwuu]bkjzjuxybfdjcqw\ngspnkpswktczjhi[pkpwicpaszrfnsa]reqjlqsucfsixykwmg[matrmmvriujnldbcuaf]lckpqdyikkaprdje\npbkxtroofyztckqg[arrmawhzlhytfodqb]pirguzqkvbgxznqnn\nmmybfuxiqgljxdih[dzgfakmxryeoylimdqp]vizjwwrhnihcakb[njplrxabbturflf]qclfldtmazmigmd\nexhynsvqvhtzexfjt[rdzxptfigworypkcz]disdlwcxksxjghkkbqe[ktpysvjomszwxdmqdv]cmwenbksdvfihvxvz[vrxbmhxkfjwgktuy]xpyefktsqohxwkaowk\niiuuszfrkqjprgoumy[svdcdtozwwtofuizxg]gkenicdslqaemvwlov\nmldgparlhmdhgvz[bexmggptmuvhkjj]hfnccpxdkireolxpe\ntzyrycryhzonuxekwt[cvskbxzwbuotnsu]pvybsdovxceqjfmo[oxjqmhruryormwvgkc]kiygcylmgxdjubtefiw\negklopkulrxyltcpbnu[nmbkrgnsjyfjugcx]bufmkakubfrwnwai[pprytunilpvguaen]bceequilwywvtvmshg[aszamqynotadciwdwzk]uivoeunohsbulzpxko\nubhofoouxcmdsqqkjbv[fdvdmyjaukqeuaassk]tjajanohfobuhgih[dfscfkxpzwoqobajau]aspwsctdasjdjnqbmt\nurlkduvyyyatpkb[zrolecowduswyfn]bgkveercmmeecop\naitmhwttzyrqwwk[lxntglszzkyjrqogob]exmxyvhwwcopudfekgu[fzxdevariaovvyuof]almvqtftjsdqkevnw\nftftrmapzrqqyql[fmxcumhriyippgxmy]igyxwlfgcjfwwwgpy\nftkqjwepfbngstefaji[ekaiaqtwacopwxfcf]deswaixrljslcqc[nqwlvvuuziefvrd]pgfvwqsqxeqamxsjjw[zispeamntwboenxygcp]cwdhurmclfnjjjwjygh\nfixhqdsaxorgfndumt[ccglwvkrpbwideuhvx]fgsxflvifyrzlznwvp[lmebhuhqemgwxpuvb]psfuyywbujlpwcekwz\notmnqzcbakdxosl[skiwodrlvhfjsuqfsma]wtyrxmotiqdinxmrbe[lhgprkzlguroolg]kjgvxaekydqxdepu[mvffwznlsunzhxknier]irzzbykjkzjdoybqg\naauhucqygvsgwdaqfa[leenmhlorfgbyorrd]soryphiyiqsoydfkwzw\naggwrqdafwtwwqjr[eafpfpxygvnfblxikwm]mlgoiwxfigmduubsr\nrglpanreckskdaojotf[yuywsgztcjzyrfqawj]wzwtndwugnelcmxpyme[uwcqyuebxpprisdls]kjisjtwisxawsufrd\nuqeuvhdoyujlazejbix[wtdxrqucvkbkavrvor]fclqcjvpxqgnkkhi\nmgpszcffmfxeacayj[eorkhzrwqvxkrnessk]wykadaapxxqmohwriin[iwfmoieivcljpem]bxhutydaznvlbuu\nvkvvkjckohpxkolpff[pepxkcsneexhhlsjs]mffyiopxkqdnwlg[qmkttuxyhvemywmu]puqepezxejnldtlf\nfkyblzyluhloblrlj[uuznhpsjgbnzghjczsq]ekddnoeylbefgmpwjp[gbfxttshaolcvhfsl]iygnwnznafbluanu[mnylijsqhwlhhbq]ultecropzmivwizl\nrwpypdkhndrotod[rganbztsadndbxr]dorwmwqoeppdpoyz[sefhqmaxuxqwjpgaofp]kerdiohsaddctmnj\nhlzqtzrmmgkudvsaxn[wnujyposfazclkutfq]yugpiuxxydkbjtqd[bxeuhvpdnzqzvrtynq]nqcwrvbzjijfjkmq[gviaheipjpncyxq]thgypvingfouyrdexu\nabnhtjtbkrvmukjsbi[yivolobglxbtivbmlxe]gpoearvtfhhjjxedpq\nuiubiwrlfkwrsnewvwz[xymjmptyaoiartx]lkyzzzynibifaahjewx[ijvyqumtxyumrnpyfz]hddwfrbrgifyegaji[tguxrbbrdvhmssvbopf]ykkkdwtdtlajkmbgnww\nomqzieitwyasnbuae[citxwhjdkqyzmfotup]enzrramzittuhgjcv[fierpodjceckpxwoiav]edtoxignggotlwka[sbjkaiypsozrukh]hdwihijpdemzcdvlsz\nrummzhhnmypaltcxrja[nbcaecgbuslkyfar]hhfbjgrmbmjexlllok[swzivorldyknmqbnmtp]yjimyhqwgrgdphl\nmvpjigwjeejzhnr[zmxoaofpatkxkbecaq]szixqtsjizfgvfioq\numnruavumjfrbywaswu[aeypnvqccjmqfflsyyn]anbehjastasljxkg[kwsjaebdtuslcbae]corzitvsrhthwmjsny[gzojgomcsqjubqrwor]tcektreziofkfzlyp\natrjsjmfiyyhjjpcq[aygsawvwkgmvjly]nvxcabdkjbowvfiuqim[nxwlnfgnkfmmrdqwva]bjqsncyahbgqgcck[kudkiazyfbbvwvae]egtutxkpkpibqcxd\nyyxasjrusephnhgz[tbgueaajlxklmqfzfxx]rbirjquhusiueda[wwyfqgowviapcam]iwwwfcjtyuokivtkaet[ojcechttmtwizhjzb]ilybbjncssrsdpyvun\nouzhmpmtsxtbpgxd[xkpvjnalwhbhiwl]dohtpyllehgsmfqwio[pswfztwnlizwbhbopug]znhnnlkxrlsswkgrb\nwdfqtfgtawjujjnipv[ffiedysbmudjwegxa]uixjrzxqsqknbro[uijbgaxqvjeiaddellx]golimewbjgojubbk[cmkrjtwjwjndagjoidq]kuaetseghitsonmjxez\nhinvjpjfkrcfikcsnk[neznqyunxrviafftsv]xxzaxudvxzpzayzu[igikyqxlllewgxp]bbrmixylwkvzstannjk\njnfqvpcsjlhmsgttoo[keugkkuywiztndixql]fwcomunksourfiufwgf[vwalfwhhknnkmlelb]lxwrjniskrxyxxfgbj\nhmxhwwoaovcmrsjng[caxzefbacuvtevwsn]lgybmbmfeizwrbfrzuc[usgudhgiwtuirjfkpz]dmohwrrvvujowdchnh\nsuctmalsyteahln[iwbpvohjintrccllib]zdppjeyrkkjlwgfp\nhmnzkxvelkvxzminaj[llmbrsvokhyfowaimt]otgsfjkhormfnubhirp[cbycbwoqvdgyvbnmkz]gnnjznpxfxwfvaoc\njniltxvpjudmaao[ukqflhglxrfpfjg]djvtunwwabljjdirgrj[zkfyhzxkarvjfrbzbhx]zrrzbzubefvchvrpftc\nlyqyzdgisrvolizgkvq[fcdlhezvozbrglr]lcuqsfwchyucocowuz[acdcsqmgffussoy]jlnuxatzdobackkwgwp\ngwcvsoqytskjaqo[rfzimztlooyjbodjcud]ewbpnbzdilxvjmwy[ugoqefqofiwkgnv]pugnbbxqbmpephsby\nbbzqqwyepafkukwqjbb[sprroemdjetnbhdu]donxkujxpajsakirfap[ybomycmhvmvslykfxuo]auqvkrofncqftmjshtz\nqbxmiueonhzkluju[yocqzkbdskeisgvm]kaasgmyupwosdzbumq[lkqmadnwplwlawznb]zxldpcgbouydtatpo[dqdshurolnithdof]sscgvlgvpgthgkhtszr\nuzcvcnjawdeonomhoh[lnckzlsxtxekacx]ogcbcsdksosgbdlrexd\nkiiixiatixklryllfyd[bdtcggfxvupbohvclg]rxwnmgvwphunygx[jisbxeqdcnocecrtabk]cpbsvzurbvmtwucvhk[hlrjqjldshzvbrn]wlmkcxbepdkwafeovn\nxavkcpvzdiowrpduy[lujfjaxzrmxxcnxfrlb]szegppqkdzrwkokbi\nojlbyagshifmlrv[qexvdlykxlebrlrjkg]lvdobhyszjfkocbmt[uorpnorysdsqycpdoje]tknlzfganuxeulzv[amollnzxactinrv]unmkoyxobuuzfwduxa\npjhpwsfoiufywtd[pzudakbhkrvzepfl]cnmjmtmacyjulpcu[yvevxufpkzfrksn]qqdusuumfgtaemuscj\nffnxshbygoxcatgz[byegatenneixbjbrri]xrxazipjarxrrjj[ilvdkjlixdbdieycbvz]lvngjqnhjjhlvki\nmaocxpwqvhfgoaoy[jthtqiiuukttxhh]qpvgjokizpojnsvgg\nvstmpuwjzkvzxakgreh[vwxiygqjyyvmgvjdhz]yanevbmxttonaonlgeq[rskehprefzmdfujh]kddqkrshtgymbyf[tdciwdrqgnrwygvlqwy]mwyxsmscrhxowaezs\nlpetegprilvnporglm[efutqcurzhuymzl]vpuzirgjkjkqmpglqoc[ynrhizbevmuobpyduap]joqowueodytoothjk\nuovjoxozjbjgjoedh[hdufcoupnwyqzqsdz]bfkcibjpdceeawfsxnb[pmfdhpjltsthickltq]wnvrznraeqgmhfh[zqsykjfanpwhdbm]oltzbvppyqrhmom\ncuptpflteqvnaexzwj[sokwgqieratedygx]tlgoqkfvmifmdguz[kfiwutninqxzwie]dulfdtlbltfjevgp[oftsoxfpwolpbvflmvk]xfbcennewbsxcgin\nxoajbdvgnaxyewthsyy[gbvxbmhptnkenvoef]iyxfsrwruprnhml[pwrbjucvopfozdjlg]ntsdilgkqjkwifjcmqq[gqtizyvtmqydqdemxx]llggegbgpbiebcsg\nosoqemdejeowlmtbr[gvnuwetgdhuzlfoyp]ynbzmlvpoydjaix\nxmtosmglxiswygqd[djjpcftewakmxhe]cxrcujdbpfpmpqaqp\nkmffzaniobvxkqobrz[xemvsxzxpikkgnz]coopvxaqcwwvcpzzbwc[frbwadxyrqsjmeb]solyurryfbhunkug\nsyuvjlrlrotbcxtmqlh[plnbhkottpkhbgrmmc]tpkceggxjkkshgovp\nxypvptyubhdywjddc[dkdpirtrddhczvbi]gppnmtijmtndwsd[jctdyzyrapkwpsudre]ofnnmlflpjenwqme[wjlbkjvlxuwubdkskq]zmhodofehapyshkw\nzyfesoxeyyvugukolxq[sduqoqepedvxiaojef]ujbihfjhwwrxjbmjzwo[fjbbqkruyeexkrk]fyjhwioedesstjkw[nyhqlxexvrlglwcqbi]zgxdbhdcqgccgodx\nkbgeflyhriyaitjdw[gkmsfhbeeftzvlkkxd]leroadltgqyqepa[apzlemfdxyxhyqy]bifkxoyxysldsif[bypdkygwlqgxlhmay]odffxnaayhgxkyjsyg\netnylemzuybethsak[rbqwbwcpspvwcnrtiaa]cxdlfpvaizzsiqy[cofixscwpmoaptvu]tuvmcbkoqlfljpc\nnafgslpawkgystrbu[lholsrbjchktftlct]cwxorzjqzuibydw[wolwkkqcflunakpsf]ftfjgybmpgmpzjpxok[omccjdarvniomtniw]vmtkovkvuahhcgj\narfxtgjhwjbqqpn[ozbglzichfmhnsrmc]sxwomutyoliqdfrziy\nyrfbyqpslcykicx[uoxnsxbpkzuarrmhesg]ohscdwcojgysjov[epkotielizvhfbauf]kdichwakhcwuitdohe\nlxdfxhtcxpaqfgud[kietvvqhjbhmbdjh]rnnxrywwubyivxj\nwwqhnufhgdpwnidwe[trkijfvlemsenfvm]hwhzclbeilbbpmbdgvy[kcqrejunfyofjviz]ymhbanffstqwvlkczn\nbemjirozvmspfrojywv[gnkvjdexdgqeqvom]akfgpxfgjwsymkegz[yrbmhgnacpufxmilwbe]taxwtqhrfqehzvndlix[ndjuozknfyplqafyu]bwogrlytfyopgayph\ntzrwkqaembipwoyysy[zmjpcdqtbucakwta]eelwgobyifozmawhaeu\npxpftlpvkjcwicy[ordfpujlgwgxccjcvc]ghrlgcktvifkicv[kteuygrgxnqbaagldhw]elebyndnyuknsxwsz\neoayeeinavevnkocsh[wlhcijujotnsmyfwrg]nsghlrcpvhazacbriwy\nmyqilamxvrkimzrypsq[dritxccifmrgnynl]ahpnxwgmmlcrmtujqv\nprjupstfryhiyxjr[nznibizpdpgsxozff]omzpiwgyqqytncz[ixhfkzmhfpctiaflrsg]fkxetrnjkjhwmbcs[mgfwcdxioxwsbpbxg]pnmcyowtigkikfbqem\nobihtythngvjelm[flrqufrqlvaamtlt]gbuppvlrpotvhgoivu\nwdovdejwygfyguc[acoacyczfmzugdiwfy]hbboqkjmpktiqigkaxi[eirojscvpewshvdslgs]oloathxikscihfpy[vbwlxhdnmpcvhrdwm]zxwsxrhoksbgnyva\nvuaiucuvucxmowfvdc[pkwwdrystnkynnfonv]bkguisxgqtsizbdpon\nnhegyhsxwcesxgagl[jsdkwvzzfvxuxsmkans]cwhuierxyqjmueehii\nnmtqqwclrkwlikw[drthkxkyfxqugph]bbneldbvtittaydbgag[vviulwoviezlxte]oqzoapkqstfdxbxm[bmhsjxwoxtflbqeo]hnsldpfruxcdnvz\nxrkijlvluezxevaye[erofwbtsylzfvyrersj]bkvnbppereymraau\njamtmykfjuhzndgnzrj[ezhkpcujzmcdkkjjfbm]yojgtkoobnwvgendjt[jkeeulmfzdbfwnohfaf]cudgyvipscncfbvmlh[kxikmcqmpounqkwjhg]emsdqszhrpxpwcwb\nyywwadanokysrfh[btwstuwbsdiotcudf]qrsrtonegzitpgnzsvd\nhrhfutggyymxzgyj[agqctqvhyfytwsdmzf]ozyonngtqdoaagdl[uuykvsdfqdknray]shhtieifkqfewhopney[ydgftitgfmfdqwh]dfxovuekyvtaddh\ndbsuuitjdsiymhek[jgxxnjjzwgwirdlgwg]xwlvqyufgiwbwyfhqn[yywjhwiwijsuhlarpxv]zmpooqvlrrnwdfhsheg[piwaxxvwgzbbruij]izqwldwwjvrxmzuj\nnuxzejoidicdupcgdum[nelehvehbccqmwnla]bhazpsnmekeqkvr\nevnsveqnndjyarol[tgeuojqlculphzfva]rilaooxfpwyreyh\nhhwvcwpwgzktzotcrx[khmiivstojdaciyzb]xwaeqbqyqwqltdx[rgwirleearklteybyx]ckiyopbgfygyvui\nzpfozblbuwkdkkfsuft[lccwcopfworwnry]srwrcwdkalvsnsu[jmgukelsagifrhkxqma]wtrtztsztpnryaqw\niszcbgumuoarzlkblr[xphrddxkyclfvnapk]rzryxqdnmxplfiu[plghrphjxgqlxtp]cxpvhwxkzkeczxcenm\naezqpvhdbflknptrc[zykqxuzbatudehe]lugjrgmxtqlxrvt\njsejnywikaohtarsxmp[whmztgiaadmiarwlbj]yjrgwesrymvzhlades\ncxmorkzlibiuyjgs[nyierakbbzkhvyizl]hmtqhrxddgdwmoayyse[ldupkxzsfkmnsfdnzsl]sfpntvoniewgfnyfw\nrtlhvogqfabwioi[mloxkofbaemaxcfzdo]ofeukqafbxivgvygl\nrjnyhsocogdwhswqonr[jrwafksjhfamqvfjk]seiscoezqmbopqryc\ntxdcwwtcedbymvxy[dbhxqovjeifzsuvm]alhqphxcmfmodeb[zdzxpgxeezjaeichq]ggadublqxpfyoyc\nrvoblfajodmlbftahtv[dgglfidheitvcqob]uzvojeukksuthhlpyoc[ovnskmuaaxulloi]wqhxsjbtaqbgjpbw[ohmzmzpqzevicbzmtk]yjrbmkldmwmmcndia\nrnsgsacbysmwnhlqjps[hmjfyywxcpxwsicxit]rnikgavmgagtsoqjnfp[qvcofkevjqjqhiqhzek]vlhfbggnwqwohspyig[ibsdkevufgsnowonkj]ufazmdkexffmxxfwf\nqkcfiavyhcmknbqcjtq[lknppgsvbdvpftnzcgo]qswbyhtruabsyhvz[ilrimrzzjctbbwhc]knpudsvkdphxsuevep\nwmeryhgvkftqiyctbt[terkorqjaagtbsp]hilrpcfcjsyguukcehn[scmgvajuiuybvzt]enjhgqtdjabbkgh\nkvczijzgmasricwj[xhgvyfhnaxeugzje]xwcxqjegagsjbvnuskc[iiokktbsnmwxknkqch]vtuobocpydqweamu[jgmazxfjiryndgtcqjx]pykbsnsoxbfgacvgpz\nguthejosohmrswzgk[uqthzxkpgxlcmqyop]fxedavqwkrmzbfr[itsvdugwjezrjtgqmua]yotsdzczslbvzatsom\nlyltslrourlevnxw[dtiihjdbejwusjmfap]hdmttxgttdqytvdfpp[qhdrjcwprncegzdfl]iinunfljrfhgifws[fvjgcqtqgxqtgca]bzlvdtdsxgrtzuvh\nndwwncgabwoynmn[zbxvlpndrsbczbklwrb]bkcrlonwivcipxe[eoliublkzenpeyxfk]voydcapbmbsiuvqfywt[mmiirgxvnbpnkyjh]pgkocrralcozybthp\nlvrcxgzomstmslr[vczvuydqcmhfmlt]gmogxiffrfsazqbh[yvnoqlavmbnattcrgd]tsbkxinrrbbxypwnafo[pgtfpwnnlxibpjchgd]hznabthirzxjipjd\njtczttrstcpmsko[mabkmpwpcytkqdmhjc]jntwxslpyrkrehj[cqbvlkhugmarodmoqeo]weaiacdfakrkuizqw[uiwkgtbzmmffxrhtn]lhygapgcdaszgoyy\nahnbwmiwwwivkykv[pcsiuyrowqrqfxcvw]mgksjiinoudrumr[ocwtmprzvamougd]lvqqlgaftlflllvqo[akvkgazplkkvqshgbk]zvyvtmxkttxnxxdy\ntsbifacnljabpczi[cmmjarpfeeyoeplv]zsjcjdfidfjvcgdd\nvaviqqmsbqellpw[xjjzxupmjbkyuzq]putpqaavecqypslf[nkyslewbmmsxvdy]maszkbnmujztqfbzq[hjwtywxdrybhcvplncc]bvgsnjtjidiuvggo\njhejwzckrrrzcjgs[vjkxxdonhncwkykwi]kyuvbdlmkffyzept[jloktbqtmtczmjbdord]uzggzgltjzngpsboyxy\nrkrntmebnqrkoboby[gujdrcqoqatyewm]qhrzxubcwkrkqibjwl[hvnezryivakciaoukrd]teefauinxaijxil\nzkuajphbyhsxocacplf[tqkosililhbxgsgp]xttqprajeocotwoixkw[hdmduoyjxcizwpa]cihkdwlaxhjzpjw\nxzcmplyeabfrcpfr[qhfkyjzmivvhbqeblph]bkwydbvhtutbtytnrx[oslchcvrlcxmsnbqoq]zkggbeglckihzjuq[lxywqhpuarhpasbul]vqmgizoanebmehzfwyt\nbjrvsfwownhpxsowafm[dtmxsbtquavgypbizrj]boqoiajglkefiwaj[ycjpupieshgdmbwp]riufwociykhnwdsci\nurcrpmkeszzuctovhqu[vsutbxseevalnah]rwrptzraxwhuskb[inpentirbmcxdvof]nvtxiwtlkeknxfl[rddddhtpudrgpjafk]cojkmbekefbmuwev\ndjavlwoikblvsufxrb[suujlpxslswxgfmrjj]drrpikhibuvwdlhvt[iopyjysnsjpyyxngdfq]sijwvhrwtourowgv\nkitztjpylzlaposkaun[szjrduixywmdpxbl]kaltysqcxzjrengtkwv[jhsqhlzxzayxdbebu]apyxjlaydhhokxacq\nkvzdgclklqsndxdo[kudsmgggtnwtxdnrev]quljmegosayhdwum[kklkxlmmmtjcretlyx]dtsexdvvjndpxtggjlw[mpcaczddrmktrpgngw]usxsptmzgzqhjaycg\noxvlhxlmhhyqgwlao[wiqlkdwjluvqwgqp]sbjmqvssbwefsvq[ocwwdefylfgvgsygfbr]fbtqyawdbswjpux[loeconwsbvgbccoz]cdotdnnkzyaupynuk\nykozujsmdopwobif[xaupavllckswbcyszd]jqdeagvmvsxpumvmu\nnaxhmkdggymqhjcycw[xkhrapbevbaiwzdn]etnivyebbwvqarn[dnskxishknmcidwv]uctdvqkipycyzhgcp\nuktvpthtrtlgmwofun[rmevlwmmvzucsuxqx]zokkayofazorjdec[ickalywptsyxrttbynx]olddxeqctucllsvrvhn[pxfftvrdqdglkvll]xymmmimcqskfozlkyos\nrlqkqjeaqkqkdsfb[igleoesoxntrdwsyoz]ujmbnjtysangjwpsod[nniriilejnvzrrnn]mbqjytlwauzscjj\negnnnubdxhgpiypsha[byoisscizhhpsjy]hmtbmbgshscaxadry\nqjafhagbtdpvszwlpz[ipehjbasniypubhfb]hreoxsqzigscxhnaf[rntqxzmxfxdldnpxqb]jriknndggvtkifa[kavxsbypdwmsildd]uisivvrtykssbvmsm\nrwxhzignxkrqeuy[memzudqlzcfrgudefyh]pyoldsepksbcbthfdcw\njhgyboztenuwlqu[zjsmipieimgaypipjm]jbjlglomhxosmwypq[lvpsqwjvzepgvzbfs]ergqdyrvicbsgxg[ugcuougnecjcrpav]pzgpppoonvamxhkbg\nmdmifuoicysmavfkvtr[rdcuzujskhncvsy]ypspsiiizkvopyb\ntlwbtllklxrkyivnnuw[zqphdjfrntryqssd]uuefrmazhsiqdbodatx[zdptibmcvohmnwrv]jofpqdvwggfsdkz\nrkgfksxcpqkspdsx[zubzkcjhpvtdvow]bkbmwwrfqtmaosodlhx[shxfozufozglsgfj]tbtwcavcbvhjourcvu\nayayqmsdvbzfnut[nzwcajbcbcduifari]eazisrtfqhzophb[zkgweftquububoothq]lrpktclkzizrutnybq[guuneltajlsxbbx]rrakswukxamcewdy\ndtuezfpubkdvxojau[ipzyfbjcwxazbqeslhs]nelubzldtozljzyj[uqkgjszhpokhonrpg]pgaebrtqevqblaxqa\nbbduqlqjpilanyikfb[iwngaxahwxongrgf]krgrarolzgmzdtj[mbsttcbkbedkcmbl]whecpxbvhuemjloxkcq[lrtaeothcehqsmbes]chuesxuwklohzrvgjkh\nsextateheibnehs[ccvuuyctlffatnmhie]xdrwtaeangizfxkt\nnayfogrvrhhvdfqf[upaiyvrvkcygazw]wtsawgmklbrjjhc\nqumnikpzpmsjvfiwapn[fdqlumgxklzlxcm]dczsgahneieodmhgvgt[babaxdoljtacfza]teoddbtcemfketpp[vazvzbcnqacbwcx]fulxjfohtywgtagn\ncrcyymrdfaawflxfmfg[ovbkvuhdrxdbhmyphao]myqpzivnpjyjkogknqz\nxfkrzuoeclfphdae[wfuevmepzjjuzlbc]icytgjlzxvnjgugxyv[ppqszfvkmppjvktn]cifddqrtlcodiincw\ngobxpjjturfsgzell[rfhdgfzwpfoztzgcn]eworfqsmysqolgq\nlaagoxczwfikjawci[sljddbmwqdnwxlkhdi]hwmoerlalfpjshedio\nwyomncmyxejknhswjv[awtbfqiarnoabkab]nitvsmoxyfdhpcdiee[sipoxhfskauxfskix]nktheznrekmrrxl[gwpmodgajfihlnad]pereyxjrernitwktv\nxxkbizhzxvqxbecadt[omafffruievwfqocujp]zpuotjhjwsdbsxteza[otcdtybhkqhjhvjjz]zjrkvtevohcfvlvq[yjdkpxspyojxstjkv]fbccdkbjrebcrxyrg\nzrctbusxagvjendfdf[szvxchrhjussntb]mzhzysbvlwwflpx[heijmktbzrbgqsklhcu]ygpkfilealopaixduvm[rakktnzhooijvydazhb]msnpudxdeaujqysbje\nxoemgrrmqqtfwtnwnyt[jextspoeediexugdgc]foyqnwnwstrguzk\nsiuojescxsrrhvgpeoh[dnizqgnuprmevtqws]jtrkiydptijrwewcqz[zkvjwozfadmizvhfdk]kamauddrolxbdrn[yzfffqfeadlyfje]qanqnshkelszldi\nwdiojuevpybfvdp[zxyrygvkvufixzdwds]tgjzjufuuwenexe[outgdpnnysadoyeon]hvelposyxhlvfmdi[gazrxuhxrfxofsrxq]wpkujtixgvfrdgg\npufjsqcfddyeghd[iylozggwqlqevyb]cbkdjgvbrpmrwrsgn[nuinkqeqchwluhwye]baetibebzmndgrulqdo\nrwwiamjdgdfsttq[xnsuyncklmryvumrii]qtcphhihqqqqtntvoev\nbwhfulscfcqggdswt[ostyvvcpdoyzvuhodeg]ekpjrxajoziohdvkfco[tbbppuyifwtcgvci]lwjfhfqfmclrhdhplbs[pplppkgrmykhtfnq]sfvskkgimpacxfam\njripvodavtgdgkv[isotocixmxjmcldpx]oaptjpebswetmacnf[zdlipacteuduvqdhcfg]chciftufaejhxkmpozz[cmnwvdkbsczhekzwi]ovnjvgsuxmszncr\nylpnqmqhlnmuxei[cyqofexibcjwunyl]ettxreudzmlhgtha\ndhmperfgtcbqlipcjbr[gkmgkletrzhoyhfcwb]psllsosgwjmtrvfanv[fimdtpgcoolukvvpu]ccqgkaqltrreqchxpbf\nhuvrdvtjmncbokh[mxnsccgwblyahbdao]mpscnoohrsqideuhf\npfvpbqmyapypiubxmt[kjfhekecjzzqftpj]sybxxlmvzhloooom\niicuihjkntpnytg[xpzlplwvgwmzazj]dfiftbbvxbztjpx[patfyqrujpvwbsl]mxgsntaernztshbi[nfwhtuuwhgsljivcrws]iwzqwnbjapcfujz\nfdiifotbpdpfvedsfn[ptkzrnhuybmhzkh]rmxekkyxbqxmxccc[icwqbjmjtakfsqbd]euycnuevdyommhq[dqfyackkxmvbehucn]aabiiukaxiowhbtbwpj\nofaeegcqivqrmtz[nyotqurllbitpijzdz]pdlsomnmdsbfhdzdh\nyxihvlkrcvzxhlmzm[asvxysmyxovvxdvv]rrwmvextlthjopu[nuaoossiaxivwwxwpa]xgaovndeadfyofish[dpdhiwlsvntqxypdpy]ddmbndbjtnpazhj\nkfqeicvkuvmsljtsez[vplnucnqgngsbfv]ycjwthuykmlfejqepad[ngklfmgvredrinryy]snsxjeqdinbbapwuno\nyznxssrnyacwtxlfbab[mpjvrwoguxgvcbtbmdv]uflsilwcemofepjghvh[cpprubjartjbnrdo]pocdfdephebcdavrxpo\nxkiccyvosgzxwtuck[oqqbviclakixdgc]kteovpyjbcejxui[mzuzcghrxtkssnrsqy]hcdpzjidycnlowgvaxo[iawhkiyhbswqsibqp]ltyzmuplqyoivgmzfa\nqllumnywkyqjpfv[lgkmvmbdwnkhlhqfse]lroouhapmomchyeghsp\negmftdtwkpmhdpda[jlxrjvldyikwjlcwx]inqnhjexcxubtzbx[nxiniqbbzoedxkyc]siepprpdulpnkrussom[srrupzubqhkmccxcnas]qylljcyzwypwzumem\nikjwnxkhkzqmppk[tzaysscnyqriqxcg]miabsouchfluijdwa[cmxeoduyguwjxqcj]ilprgkdcvvopotdzzon\ncauxikrtpgqgwydmagf[nrnvqarumgmthrf]xyyopmoyoampemafwe[jwjgmglxphjkvfg]oxltiecspkarhualt\npjzcgmqitucfyph[cxxlbsznvwpxvzghv]woqulnjvvfjvjzy[wgxczusgzxnpkakki]fvtepvwjkaozguggqk\nfgwvbbyiyljwmkgcmic[gnohlyijeqfjldrpqey]qbdzxnxuiprcwjsn[ogtlzpxxzbtgfbjx]wxgaduaiyihyumprhe\nmgemsvccgqreluv[qrlpjfkdoinuyou]ovkiqoqefrjmrzgb[fzmqpuzoufcybpucq]aaftwlldjkholezzpk\nvxfsphugegtougthxk[lkvniyzlltosedmpgr]tomgbtfosxegecoqtn[mvptnxvxddkaqnjvnue]kclnhnpveadosfktw\nltlrncoqeeupwtoxv[yoosiulyjjmwacymwfk]vdgfdfcjubkcbhiixv\nediaeekjpbzidrfpu[rowhynyrchamhzrp]wetzubsftjwuksnd[yqbtzngplxcqkyxf]blzuvnektffqbkf[egmvyplsbysvfjjkr]ikrllifuchlkthknpqb\nohspsyvzulzfsgghvbu[tvtbzqptcpguecpgb]zyadwosbwchbgrkypj[cphkhvagaasozym]tvgkhkooyejddnhv\nuxtuhgkkulhrvowswt[etzltbttiofnkeyh]gsgnleidfbomktjtbrq\nowccdxohulgarvvxx[pbbuwbbkrgqlhxa]lqbqozlyegslpxvr[arduobjtbducuoiwykm]tfziqcucaqjcfrc\nfoxbwdzngattycaunku[lnkqgrufdcqreruqp]otrfaarzydubngucw[hhaqnaieublicggcep]jjvurleoxyatgtlexjd\nbxercunxdkmyxoo[zuvlzxstpwfmbnv]laszhsamraptopjmfx[syvqwydkiawwwpb]dyrhipcnwwbhmcotha\nmrcbhykyikojmqmxr[gijdvcjehxyzlpxms]bkzqdkykgcvrlbdcpck\ndqdrhkhanojahvaof[msammceatlnnwypjnk]yxkhkmiroydwvls[bgxvfxasrtzmiqpueoy]esjxrbelpjsvdcdx\ntuxcluskqsebpcm[xplkqkfmkdsjlgnome]qkweswhvzqmpkujows\nnbpwnioczrkicxddphr[zmtlntcztddnmcl]gjultcfncpmekcsosbn[pzwvjmfvfkanhxbhcy]kafsqjaraeicizjy\ndrcviwihoplftyb[xykuycwejtdqehmuf]kfmgemdaoetwhczw\niuqdiepdheskvvgvix[ayfqccpnsyzawotpt]xjmljfmrhvqedfsrdg[rvdqhetiopoykpopol]lnqyxioswrssucownvu\numqpsyqwafisrktta[eqncbzzavysoixd]wdtnkvsvsfcvfks[opjoivoqobrzeepln]ziqmbmxwsppwzfro[mkhssttidvdgsvstov]akkdvcsjflhxllpblu\nqjlmfjwtglolrdxvqk[yufnmwyfhjrqzrxrddv]pzcaaeoitighunvg[eamjujwzolooemhj]mxbnbjvuikcycvnfuh\nzykdcejnrxpiimmbf[ofuzkgknvcexqzxpu]ketlytmhcmzvwtssaq[pgruobcnyaqmyjvospf]jkkvdoervshvgeqwj[fiexihxudpdrzdwp]pzmgprenvskgbgupy\nedesihewpfcjzkjhhk[ydoqcgosoyuebpoib]oaxftiagsynwawlukdo[pobikbzlxzzatth]tzvwglytrgbmlsdikum\nrvdcduthikkjrfx[oxwihjkewocfvjpq]wtpoobflhevxjuwnqr[ltfcdcjnkkfetnor]obpzfslqfunurzhpr\nihikssgoutovoropq[nitrordhoxvqfbjfc]lxnjmoufkqnxizdcthn\nnsnkrlllkoyukbkwikp[anhzfrtqwndvwcndm]xyvidixcvjwqwxbsctb[awnmlqopvrjxyvjlbn]ldmgegtwfkvwjurzk\ndvjmhdavqxdhnbglm[qopsknwswyqoqccp]jycpmzubidfbwsskm\ndstxfmmohcyoivxmci[prdroxyvxqzdrdsu]qzczowwyxtufoewluu[ywzeufezgbazekly]tiifyttcldlhravctc\nanocufhbdffrnyhxt[sopxugpfxbbjlsgtdc]nvnnbdsjqfevwbgbaif[ljuuwzmlrnpjvxgbp]hoeejpqdkbrafcmv\nmvoaumknaokkjrduxj[anhqilrxkkqawmtdwhd]zuugnxwinmpwchymrx[ftylpriufvgtanapyy]xnizqpmgcbbotfpru[ilovypboxtuyozqag]aldfcdeyubuntmvyv\nxlvezhyhuvbnhgezw[yvaxeeokyjwjgzr]hqtybqtojttsyhycsy\nbjcbsmjssbubqixiqmu[uzycqzxxixenmtvz]ykvtnssyurdixcswneu\ngwcwwzlhdufsjwaxal[howbmljowljdsvbm]jggvldehjwoafvshlw[bfevufuakhrccqcc]dfufvaxzavehxgwb\nxuigvxgnmagtmdke[nxkzzxieoqxbaei]nqnpncmtrsiytxhy[bqpabinchcjqcjy]ysktjdirrevjyqyc[rwtodjwpnppdvig]cxedadgimutpobykf\ndaqanavryjmzxflo[vcpyomgckepdftz]tizgysgskfuntqedhp[bkasgyhpytrbqvgf]dtjwyykxvutfihl[dgidcqrglxeuqmjvryo]baclxsovuumhgjffx\nlpyeghloevhgthedzjl[schxctqynpinoswgvwv]jpuvctsvrdpdhwsh[xdjqrqfwodmrxta]cmeizobaqtszfini[ttbvcouiaworjdp]uwfkbkxwhrkeugsccp\nctvifkpejmwnuapjpjh[glykzeqimofbvirvv]kbzjjjxmiasijhyak[ucyzsvtasjfewtbm]zbhktdmufikfwsiqyfz[kolsqantshbocapum]jvjtmsmzjvdyawlrrv\nzbxgniymzkidlugns[xsyjfooxpsbhtjvjp]lydpcozhcmkdiactgsu\nrzsziayhprsxlwr[szdcnmcdpqkwlmhqlp]uctizqyfzorwogahopa\nnjpfvxluupsvtbenq[cgenluehtxacymtm]onnngstsltmtobh[jkjpmbsumgmtkbyg]uvsefrirmvsuiff\nqukyshliwhitgmyeb[eikuuslkfgergykosp]fthsbtteuspbrqpssb\nxpgwgflgtkmtzhw[prdmpsbkrcbmjfitdyn]kqiyknqfoudyfvdmlhz[zswwgwvjkyvrjlg]zzmkyxkalhbbgcouvog\ndgxbmggkttasrcjotn[hsfrmfxeeuvovzuij]lnbdybfhkdsrymhu\nryjamwprtdolosp[nkucayakarxezyxpgkp]qnezibzbjadqvqzz[kehgcplpjdlitdsg]nagotxuswnxikkicoi[fbpbayqjockutfqu]gnylxqhcacwdrdhlp\nquayrjbyxiviwukq[mwkxplqhlociiriaaao]lswnrperjoqewphn[nmwqzenrjmgikodk]sagkvoqqoayykkzri[uyenuakxyohedlz]ffzfpyguqryzodjwqxj\nfkymdwjnylzqnxhl[lsrorhrzdxpfkmai]vfytomporosnlpzc[pwpodimqjyfmczra]nibuxkjazxghetmxe\nvlrxyrxugxmmxnr[gioetjknstpngomi]jgzsfyvgbteacpupi[aeyhvaqkilxenfy]ezhnkbgkqgbymgzolq[dkzztikgwfghpltsd]nrslpkmvahlvwfhavn\nxpjvbcihegkoyjg[ddyxkmnhpnucgbeu]xnvxewhefxmfesoqkfo\nqgavdsmekecmyuuxln[toczsvzymwfzzrxprb]igonrcvkpxvekefo[abktdknxsdmpionl]uhhlekwqmalhfauva\nuveiuvjjvxlrlyxpc[ucbsqehsihiilfmxz]nvhvrtaxdpiqpbuyj[rhtfedxbiqutzvaucj]dxtgbmuwqxxqpfbohfb\nqerjjnnafocowost[axrfofdityutyzgv]acicnljrpsxzlcg[dhslugmdfaxclhrdecs]ekxnsbqhlxcfuron\njknvvunefcyqagtj[zhgsvdlsfrlcfyoqt]srtokcehvdjwwkcwczm\nwwwyfmlxivfqcmnwtw[kaeymickhvsdlqkfuqc]dyzktnegiqbohljysa[qmnzkoqxsgtpattmt]oxxczwgodhiecoyp[swszkqetvvgdctkhyxo]qrjhaothcmyajmpy\noldhdgmnxrbjncj[kkrntxgkrpbrsyi]qjronlhwmcpdnpp[ksqudrshtdnenqxt]wzbkmgdhgylcfpberv[nyddphsypgzienevnmx]memczjhmgzeyjchv\njxojiumgecewqlc[nmiruhzcybahusxwt]pqlrbrwjitwylvzx[rjwehkmounctpcecz]jbhagxjlhngeibhh\nlbpildbxlosyqfun[razlyptphvjizuyonoy]atrqbzjakphxrguvmbt[ybdqfljkspdlgisypun]xttstfdytowwtxytsn\ntxrzvdxevhqzpkb[xbsfvyjkimceqeog]ilzhcjiezytvmdd[kuhqkwaweasjoae]fuyyczwcpbdblxtxjgt[ujdwvuypmibgdbdtkij]vhrvswtmxfqkwmtjjld\nzipaigqfaywgroxzyh[nfaubfwofvgmjrlxw]srjdkzejhrpctlhbevh\nmtshlkbkfdacuvtjkbk[qemjvtgzaxmgvojtfl]emvduvrdlxnwgqrquk\nnekajppmdnadytnn[ynkibteahksyzvpenmp]jqxybiytpkgzgws[whyeilzvjokewweunf]ndkfvbdnbdoszwfugue\nfwfviekoibnqhpis[esurgsppgqchztm]vaxsbcgtqipiemvreaw[ytkxlxyzfifrxgmbggv]tygxkuusmptxqyl[lpuxifizetrlbsefado]rbykxursrelvgiilrai\nxyniecftatconlmstl[rpmxaolsbezfwzof]zvcmwpmmcszbaimwhfj[hggnwfkyexqkdancmc]cakzrmvvnmyiyzbwx[eizlhdetlkmzlrob]elvcwtpqtdpqxwdgjd\nyfxqriltoucrnfnj[zlvarepakboasju]bhpvqvllpphryccbjz[gilhjdjlsinanvhhe]rkypfwnsrmshanawlb\ncffxddoarujtkpwt[vgtsjcyuqgpoklcem]enplegjrghgfkvaqhtc\nkybnjsgrfnckxytl[obtlaqusuhkyeswu]vhaghsusagftgzxz[ganwwupndegfgxbckde]ncgnimjtllrpmajya[dmzimljmhjkbyozpmk]ygyhjeeexzqadcdyhf\nicjonhtmvgnwowp[xdtgaeotcyiyzozqwd]wudhamantwimysgpu[wjeyfkqluqgmbspxi]piyixwwkfdbogwcmtac\nqextqvcvlshqhbunkg[ouypttbdsycmscqe]qpxtjvipjkrbasofu[lzonfnanpflaekzhl]xwwxnjgtmzxnhmq\nzbtonkedeacrlltqnl[qlssupkhjptzbbru]nroemsymerldlshy[anmlmugxtrgypsvkgs]wfagpjfzgqcdhslmlnf\ndpjpmruktkfkpurvcks[mcdigtlyilcdvykpng]wrbydnqwmaatgjpjnew\nnhcyufcfcqqsxef[msqbqdsheiodqzpkcv]qlownycyhpteerrdfid[geiuncokzuwybrefno]mgugljgzgtdvyhpflbk[kwgpiyryqpdmphcwk]rghcxpkbbmimkui\nyyutoljmokemaksyh[ofyxkifbjqhrdklh]ltfjtukyeekhbjd\nuolodqcxatkpbywxs[qdpmghhjdsvuolwk]qfvcnuajofrynqndg[cpojwkswcxdorxvknrg]hluvdzuqsjsvhnqd[coemqesbuoorqrcht]oymvojeakuzzydb\nqrghrzhmccfpfymd[ejpldprfcjwhfthnli]wayofelvbtvjfesq[crskpxtazgepeguyywt]hedblyskngtnxnchdz\ngvebyckhjgfmqrxmmd[eklljmmtwggtlqdq]hmxazjnitvfcjmlactd[qhlsytdoiaksvney]jsdeegafywarxlsnkl[ycoyqpbbwsanlnoes]mnfxjeakujicrhn\nttowopleauigqfzpuws[rwaipjqlxeajbszmt]ewurrgikabumnsg[hqhoudrdngplyncdoq]jvazavwibnayzbkmei[yfeaerzswqrhjiiqbb]khsqzfojtdimvcgsxuv\nzysbeejbuanxhomwne[wzcjovlgygbogvj]wqqbmqmudmkidhnm\nhzetqrjsokpzsfe[sfvglwbyaoczjozubjo]fisxeqpvyscesgy\ntxsslfbzdakhenov[pdzbirgfxvyufuz]mwbclrbkpszfpgbrhu[ozmwusngkhbkluzvgo]wuwvzagakqcmcrcq\nvxmeolvgvkzdbldvid[ebhmwbfcvzykllewj]ngsvjbjjbyyoybnai[vvhfsezmrbmdkoxbdmj]pxxmcprffpzqadbu\nkagnhnyzbognzsmifby[rujzhkfynwygbcpuoq]wfgodhqkdextspa\nmeyjysyguijkyen[vjyhsmvoyoppjknvivn]yuyroikrroyknlkgfn\nyrbljqrlekktwvq[ubrwbmlwxxtxnwa]ekompfyzprhialu[rdglmpamldxxxsgpmwk]atazfgcgkzbjydvf[sjdezkpgsienutudx]zuxyrrwpglvstutp\nyqhreymyqostwga[wngmbpfomuxgcyqdl]jdkppprtdctuyaonlqz[dfpqdidzlofdishhmot]gnifxcpfecsxdincqib\nxdfslzwasuifmmi[lbvuxnulhamtgfyhwz]sarfovphjgpdckkrbgy\nbzkfxruybgbjsmeflp[ubqugccjulkryeh]yaldnucjnxhktrgf[jamlgglyzdlaidp]dsvhuxerhecwhjslfk[yibicfmmkiugttqi]byyytkpsforwainomd\nasxywcdszmdtdndivdg[qkyfhaxaietrign]sjpliketcpjxkwxaoo[vmjxfuqxqgscfpd]mnpdsyqpnhlksmrcpa\ngpgcqhpkdzpmjoxbjvk[stpachxjlsdooglph]jaaoaxtyaogvmuhl[yochbczehvuvauxj]zatcmyzbmktdoohzgx[cbwozqlvqfssqaagyf]dkeooopvydlsoakyc\nblfmanmskfsbhnj[qurkejaextecwkh]iekzoszfdtcjcvqf[cllmensfekeoduop]kpldtlzhhnyaweelg[duturhserahslsvavl]tlscacpaddzunyhknql\nfgtfcerscppphulhdpc[cjasnicuepcfcpwwq]ubfqrgkjexhpcpdh[fcuypvlkciryarmpsb]lkazlfdxilmfoccr\njaytjcjzwzzrwrosfig[bjwjolqvmwjwehvkyqm]qdrcohrlcqldwsj\ndarwjaqwucpzrgob[utcloaeoixtgcssljwg]daazkyzlexvrwrvcoho[hesdrjjliusilwgn]kflojebucroplzdkid[mxvmzdobkvksvvzg]mllhibzchrvzahrj\numabodjruykdkzuebe[pdyqfuwbwbnhvbgh]mvwcfyrzvyzbwbhen\nuuvjgoiafuuacqj[ccihiuugtipqyyve]xmtwktbgcgwvwchsseg\noldckvjhhtvodiljhx[nqcvjxjohtdbukds]qsspbsmfdcamiwwr\ndzilyknpfbgtdnvntf[fzelzighvnvvqypxz]ntthcasrqrblqsk\nhphpardvfoqnqncq[ppvkmutvbzybiwmmcuz]kgfwazxcanccijxdxr[kvvrehncwizamjfbv]ptzvpznypbvmrshiq\niteoprxpltaartmz[mnybqocmkusetlywx]mxfikdltxvgvklaxzqt\nqxldpbwuuyarzvlokm[peamzjnqawztknvnssx]pjacikdaebekzndkqbs\nkswrzqhftfhqqgetg[bplpppimgpytieviwci]gfeqifrktgdqxzw[ylzjvdvhoocfxoijb]jhullyfbzrzbtiujxo\njbyalllemspbiba[fihpzyuwtiisvalzl]egftfecpkrowpxz[fwyjugfywhzgpbgxam]iuwakremprjkdfqep[cwjewifgwauyxaqa]gfnznfakypqatvp\ngtdsifvoatfwztxsgmn[lrdwcnvmfiuzxuyad]alnsyodvmgpdxqk\nffyhycigkhlyiopmdx[yuuvtuoepntnqhkof]atumrmkzfhinoqq\nwrkcbbifeyemfppiaga[msgxssztbxvmdii]ydxtnokgvpouvcuk\nxivexjhdjysgmklbjp[scteqtgrnyuxsonvbx]kzbopsageoqsymtcfo\njtsjoerkjzurnysfnwe[jqglomdcjmtvcwvhir]rozwrmwjuehpapebmgz\nqnscyvubszfeloscaez[povhdeeifvqfpyd]hdpspdtgtqpklhwqjec[xtqeoudrdzirwfxrowf]dllykbtfgrdwdlchn[fsjzptvngbbulfkpkh]nvyonktuxkjzpsciihm\njzrrmwegexitufpbx[orlvlpnnuklsapk]kpwkwfggbcxwdxvp\nhfvhjwieruryoqk[qrtlruplpqjtwpuhhoa]ddbsdfqczwrmnrpm[hjjqrsppkjnvxmjq]juvwgpsglqllqhrc\nwogxentwvncxpjbntf[lunrnlkbjpkqcxprp]yanygvijbyhhpohijj\nkjwqxolclqanoyfes[oeasucvzznhjxkzlqb]bbxecjmmedvyfzapfif\nhfdiajyktrmlfzfbv[vdnyppvsruscsgvji]opwnmoadgirnedufn\nmrkqlpkzkhbfncol[huvazflnaswuhnv]pznbrubmgazkzfvkltx\nlfqfiunlwragtrknwpx[quvtbwmfgutkzaeng]kcdzgwyybqugyfgf[mjngrfgzmtbehzxzsbg]zjvpmzakgijjfyz[ghpyxsxuycqgdipdua]bjqtbqlzwyinovhnmmu\nayagxnelxjvkqkwhax[zlimrxwrtlqtkvdny]nosfkooohodpzjp[hsrgztcucnuagedqoz]aujduldshdugxgbszom\nwkeqhrtgnhyektefk[afuwzaqdvmzzzgnuvw]aaisrnfyhuifpglpgp\nkpqqecovarltptjfdf[fwpprvpqfsntlobpdm]dtnujgpbbrqwqdyzs\nalnyvjvicoigistbmh[ueworbfuagjnech]dpzdovbhhbguxpginqy\neiumooyxoukvaqoiv[qrygigmnybosyay]byhcqoggajjtotnuw[wpgsucwktfgcuhhi]hwoelhsxarzriqxtwao[nvemgikmzntrcfr]uguazrjfisipwrhcbn\nghierhnuwvmisxxa[cmfxbenynymgvcrr]oknavjpheqtlsvwabd[izrzgzwvdgymivghdpv]fbqrtbvhcjgvbkwjs[ivdprbnygkhgzgaym]ziwhfgnbawgtpmkswvu\npqcsccgpceupnvtr[bzfagcvmbelgxyns]uxkvxgveigehxsugzj[oojovkdwhojqcbilwvh]xeamwxhelypwwefsabq\niltmsmcvjnhczdxoti[umsmolikbpmqnsyah]tdtojhhqszysiqkfqr\neubknijqrihrbulq[hfmdunzrzrgseunf]qgdasqmtmgoacfid[duazrfhejbzxepx]apwgpewymhnhxsrx[judrexlgitldqqlnrpb]ynfdtcugmjvpdajapon\nlqwdkmmktuhdbawow[lsrovmkjyktyduf]utmrjitsbijombwo[abvvufjkwoxsthzbao]wteqdxfhbqrakiqenh\nphudxliosbjdplwzx[wmreutzkdlbxfksjt]onwnwzbffksdsrrvxuy[fuklieqfenqwinbmf]ckltdwaxzrpebmksn\nmldqsgldkmerpwqlg[thmshstolghijyjy]xzhkcpjyjuydgxjm\nwpsseyevqcibokcb[hnqscfwtkqckqmao]jsnvfanwiodlasx\npomqeoawmwhijaq[ejtmvzlmidqwcft]hkeetgkruqgmnpoi\ntwkcrdetwuxaxucnjv[xffwyrqfcqouyxmkrro]ezewjlxapphabveea[jfyjgbpkflijwvreer]nesuewscsclvwiwkn[xxjkzrpeonyctow]yclvbgnwgcarcxos\nugndgtdqyxtplkdz[worxgglrocgtypfvmb]lcziijmkjfdpghkjqfp[qomfivwilarizmq]dnglkuyyinegywu[batxtrembnirlwr]ovrphoeyxqnhcvmts\nzgtxjxnktlvldrxpul[rviiugbdqcysxijrc]kyktcnhhtompktirdjz[bkusovlvbbigibd]airrtdvywvomcfrhi[xgapjazusatwmnl]usdiffjsbadtdonojs\nmimjtxkzfsnijawjrey[appuokfywghecatbzwo]aovbqviminrwaszvo\nkcmrpjoggjmfzwezv[onaeglpwhoxczbw]totswqmklmzrwmxdf[befvnijunppmomoduhr]wydkdiejzzdppny\nfgpjujczabbtkxwvfd[cicmceziihzlkcwdwhr]sicifccwrljuhteondz[qwtxzkpzaspfynin]scyjunafukgggpc\nbuyslulsiiwxkge[ypiuwaxgxsqpbqqx]dwsyrzemulupybvx\ntelsdbhziecdqvmyprn[hqpxpfnttkmchynab]wvopujdicijhmttrn[orfuzixnlfdimtsc]jzvuxsquolwwtzr[dmiytgapehniwib]zylakfeifdzatmqpb\nklvmlkigwhcckkyx[qxriuexxfsmfcpgvlzb]ygklxunjumjcmoph[ychtcmyhbyipspnnsr]pjqqgfbcsqmmrxbtj\nugulusabrxqyxbvv[atgfhjdhplritht]glsimouvohndboxh\nfatrlhuimyqjjobdq[xvvmkavirljwcgmkvx]kbesaoxeeabtywsxcwr[pmvliimbudlzabbz]vseagltcmulcdib\nvowrlwyrxwivzacnop[fegbzczrceczdasjr]orroaksljdcydlk[clwvvrdfhommqcn]yqigbtlwvklqxxiors[uliodgyotgxdymyi]lqverjsyuxifpjoru\nwevsnwwlgslgxsof[eyjhzwdmvusnuerbqmh]mjzmgpkhaatmwptbo\nhljbwkfykqbnpqhkfuv[uirnlrjpryuhtqztz]ackmzmullgwefgug\nlmumdzgnhyjajoazd[yksltxstrsvugowym]xcmwqzbluyzdlbpkfkj[sbnktloqdabygsmyp]pyavvgzsxokeecxh[xcoublhmghnexnts]sdbkqumfdezjvqp\nstnccrfzofqwbcafssa[toskkshmnjeywtuq]kbkyxwghqfgrtxs[myvqujeowntxqiekgxh]dplyqviwehtzoxrrix[covstbqzxjrditsf]qxyocadbpdqqqpadl\nevgjdjnbnzmbzjpbfm[cxhsxvxtdtdowbd]wceyuozkwdjdsrsarl\nrbnbqreygxxaufhws[alsptejilzoslxfj]xirgkoxgpdsolbhqiqb\nkpzbxjsrsdgzstpc[jnpsoqmjqnfzkfsgq]tunpisxseqxjtyfwij\nkegehkcwqdyujtyv[qfprszwdyjylowrl]yqhpsvfmcofhrfn\nusfdjspdmrsmwotku[phpquxkrbrefnesvoig]vbrbyhzjjueflzur\nahcrumgrsucgvcvs[zgiwqzqxdocenumve]wwmkejymlaysmpr\negorqvqrhdxdcwglb[pewidggmjfdwchmpuxq]vfpginbbwnzhzutt\nrbwgxniblxrzdux[ctmqwdtjnnoizpfxkb]cjalwfgvfvehdshc\ngrpqqrkmvatjnpe[fpuzplowwtztimw]zsebojrxdfyouujqu[jieuliemrlsrrhaaral]vapfxmifbvtdzjpqfn\nkxqzgqwklgxylpccai[scugesodkfdyduxfgpq]qeoajrdmbkawsrcde[yhplavixoxekedvoq]oefgpvukotfhzxvdpt[vfffrlkuirbixakjbg]shhslgefljkjhdu\nxltaldprsvinvsgfg[korqzbyuimhrmxg]pamxettjpfchnwvxfb[secngupffbmiekzfewg]jzqfwquugmanazihei[ldhzfrgdbneaxjjndgg]toefzbwrdaiqssxrbqh\nqgiiylhrxzzvniaegfw[vfxiqmehxnnjheiszxb]txrwpqbqkdbnsvt[voiphlhjwxrkcyrarwt]lhlhcobxijaoosyx[dyqmagxqryuyfbat]oovkonlsaeiqnil\ncwxhidoqdhxragzpib[hjmpsaxbqpiwqhy]csdontizglsbbeh\ncvqlicsscacfmuugq[eejkmtnhdfogzpbhygc]hsqpgofmanfemhido\ntsbgyswofaablrj[kxsfwmoymlmvxujvqc]oiatufqeigamjtqj[lbnetvjnhlmvyjs]aeeetvtqgykzstpt\nzikurkodzkxzvjucknr[eeldigjdnjetqzwtl]itaxybvtwbhjdci[hbkvepoewuzexeg]ohfbodukqdlanpa[rlxoscpwxfbemxvye]ydahcjuodtvinta\ndkdquuhvndpmvudwjx[hofzlmhpteoarpre]sdvnkykpcblbaardmf[hdtnalxmijwrorx]ixsdqmnoqrieeqn[tvyurwrpjzolmoqn]odvpdodyhdjvcaqi\nleufyoljrgauyshjmdn[omwkxoqtffghqvn]iqpnagprpvmlsvo[glbhtzdectgrymdzxf]dwgpfoqsivjdvpiidzo[glnavlopicrpfkc]nnstfkiqjxccqrvmg\njdpqymeesiieeeb[iwrygkpzdjttxuz]qqrbobabyedbigesuh[tmfkwpopdgcfuydhukb]mzldoxgjdeckpdvu[obojbnmmlhdwsman]nssaclvkjwmoozuissi\nupgpcxmqbimkrcvcmp[ivnacnyueiepraljdh]vfagabifynlpbjdc[dobimimkhmytben]pgasxhypmszdnvjwnwh[nvcvwfgrqenthqcqlw]cdvvgepmrqskpffhw\nfifgarfuqaoifkymgx[mvgawkhnxvgaqdmzat]fuemwmfadtlaxwyslr\nbcbtmtmkhecpaemtmec[apsgtrjqwqreuntmdyq]qecxvrivzvlkwwnzcfv\nvslhwcbtvnnkfge[zbotbapnldktkexac]ieekqwkifqtpzwsb[wjjwgvhvnqaqmrmath]aeauqxrfhwdlbsqx[ijqqcgxjzepgnbru]uycbebwrapkiobz\nfgfxlcgdrvbwkhf[gcdnlfdqppnocayj]kgluimmxtrnrkxxy[ebmozaizcvfxamjfgfl]zxjsthsrjazocerdybe[uiodgjwmepojoaswdqb]gsywzobidosuauosihp\njocqkcfjxtprwzxcol[jomzitpuxjjstqj]jyaupzbknhzvwkwejgg[frkljzosjvpzzffe]najjqpukuhkyseux[obvojkkfdiawyysye]awwxmmkvzedenpagx\nwnjitpqtpbywfdfzqb[zsmozjfwpksophbzrp]ryxeuskjtgqxlkqinbl[jbenmfsdrvwdjfxhibx]vdwygykkkqqzoueisnu[xgnqjjcnbpugkeuaon]wvyttauvhjmdqcbmfqz\ncjikxgbzdupqnoq[khvayknbckfnohcbc]gjsqdwbzsjnwjblbe\nsknizlycschmfbcbo[glptboptcwtmwmyj]hmgkwtwaifrmzxhee[dxxxiulybtkhkstynq]mjntafrkgppmgisnz\nvbijkdmufqxhuinw[nqkbpwcxoozkrllibiu]maiisvopemncukdedg[flspngjuzwaveawgk]lqinchaieoizrwr[tuyuxyvxkesiktilna]rhyincnkvnnqejsoxp\neehvafmuwihwbizcao[vnktgdjhjeatxeshjh]taoisnoyefbphntft[pfzlfnftyvfkkmau]gxmhcurnvyqxgffll\nytdqzmfcxjezgvr[yttnwhebnitzkmpvg]gnxpxseopkiwdwq\ntiygnypqepfcbcqasq[qoiylamohtllezrd]hieijornlrltkvvf\ngcolxjnzzqtozkqlo[gwiytfqkewszkddc]mervsuxdbxtqkclwli[zamcpapgayrobsrnros]skfbjychckenvdnk[msqqgpdtgzpbdsflgo]hswedrxeichgpbkt\naoyzbbkhsyzouhf[yuheesbhrurspvkoeoa]icwrvttxwvrjodooy[lclcdnulwihttoo]aheoekyzcrdbtnkdn\nepqxzqeqfqquuvaxut[rvniqevejzxwbgdj]mdozdllbtyxiessvou[ftmdtfmxjktmdjrp]rbdfhuqvdzpiyaw\nfvfozofyprhtptnvfvv[cvjusvxzqhknsrfuw]wwjlogceospgxpoq\nlboiooritgdlzti[dcvmycwryuiwrxuf]rgsvwmbouwqweusdsrb[ncalmljnmldxtgjyn]digztuhetumfrmzwg[jxhgzioinwtdfvsczf]ormtzakkenigohbn\njjgkkenzhjxreujjury[oqbhgbvyvybhznj]lzzpsybrpvmfxftasjv[fajchcbbxzyjzdmzju]jbyovxsryhenhqd\nkimqpwhmrecjichuf[biclfkhxsptyasun]cykzrmdsfvyszfldtxb[foamaxeacbbfukrav]kpdkasbbrjuqndsjf\nixiemjwdwfauydlzrf[ehczcannzlhrpuu]zgmsdfleegepchlbml[pxixfrfqusymnyad]wynixqpqilkigha[ujtjksmgswjsqlt]uabmyxgfqtqxbtggvoh\nvvxrjenkffmjasf[zxizrnxsywrjpbsy]danlwskfpxmwozazt\nhdbwqsphlabkzxxhrgo[erldraphnhaevid]ynkxoezwjpygvftw\neynyhfzlfnvsrguftv[olhsgnhicqlhqcopiai]azubeqximmxxruopbcv\nixkfvfumxiagjybsn[frwibevmaiibyzd]qzqfzepjziatdpyqmr[onsezbgebekxybzzqzw]yqotbtwhsuxraexdfes[sqyxxukeslhogqaftl]kpqsxbeawasfnbwm\nfbotlkdfsscgahhtbvr[qzlujuyglqbktek]fitzbfribrvygprgssx[ytfthkzieycghddhs]twelmrjujaidadamq\nnuxgihsikrkmrydy[awvlrjbdobngseyw]owlsggrmwypppcnkmws[ipqmpwdvbohtnbs]nutezdkbigrjnveau\nftxpxuuvsdipzjvmy[zfrkyfvducmhwzfdxj]ycyrhdiyszpbldrqyqp[pdhfnaicafoldftflv]rskyllsuaaxidlokgxz\ngqnlikldqbizpsceti[skfmnlrtbwyqrwpi]ubwivkayvgbhnixj[kmlxwcfmudgamallj]tfwinixbevrrgzozw[iufudfqiwsyjcyqrs]ujixfobkouvxhmvcql\niddngjedxnwlbcxhkw[yqwiebcdacegykn]saybhmmqxdoxrrzced[bqjiuuqpbxczshymt]qagtwkbyyslughgsxrd[wjjqtpphygirijzcnun]lvwqqctdkjvaatovttj\nqzarsgfojoaqkzb[jiuvvyihogymomqddqs]ekacrjmxsudjuvjd[dkfjwxmpbviqeuiotlu]tpmzbyfqhelgtpic[xcankncgcyaixxcuaj]jsieyimscyfvaeduf\nepqisdvjvcpyxcwxuu[hhdspwfhkosxunncv]iibgrkioklsoktfp[kjvjytinytggjurws]oekjstnakyoohller\nyidewjsqwykhvakby[ewhvuvpzmeexvwtd]mygypbsbaabkccvslri[dgaksoqgxghazflkn]kpdssbszxhpltdxht\nijhcdyyvjscrvhh[fpobanqwzccnyev]vtvztxptbegfabvm\nfcicsnaoileyhlta[ivnthhpicibzhtyfaf]agaffazyjidivabel[zprfefitivfahmsx]jxfvpjrbftgokdclnw[vfmlrayxecyduau]dkuaarmbkuqqjuva\nwjhhegqxpegrypjlpvr[orhbboezmjncmclamy]pckznmicczddarise\nccxnbhlsqrtqcbrczci[zwbnllwffvdsmmd]wdcyuartrmykqbvmlc\nshpzokvkrrpypaohp[cdbxbviwegleqizw]dcilynllhnasdzaku[brkdsnedgdlzlhxzlzg]ygvficcbzjonmzh\nvzdkvwtqbqsgxenb[dfrsswrrxxxlpxpgp]lheiqkpbahpgjtvax[lbfhfdztehvveioipoj]xkpbfwdxvkcndrbfgya[qvewltgemzljlokhjxi]bufpvhmvhrndnkmjsjr\nmynfnfbjlwljwoqbenl[wnuganfnmpqrgcdxvn]kpcfvfegyibrhoeouiv[tmquruuijoivdluhc]lnspgmbphvhxlcw[slrraibkhqkaupb]vxwczoqsrepmgzz\neaeovlebqlahuiztd[dngzrklmortvzksk]atunvakfxeqeymw[huaccbfdtygotzubrj]poeblqeqsdqpcbqd\ngzbgdqlebuwepvx[qpajreszsyyluwi]hymkhgxqpabniqzells[zediljwkqfpvblioz]zguladbcmloyugl\ncvkyjumasouhugvvz[dtidgtxbbufhwyvob]pdmhzqubmdreglyy\ntcxjcacxysuimczi[uhflafmjntxmsaf]uexrhinqroupcbksrsj[nocrykejeuzzigkyqxx]crwdvpjofxynwft[fmxkcqrsrpdfxscabs]crbnlnzoihruuilu\nnotkmxwmhfptgfpvntf[ucdfxyikwxtsumebhj]kjhhkgtruhuqzsl[nyiklbrbfvreipanby]flesvbofrdsclfvm[zghcpgxoauylwmlzfl]vwotzewzjzpyccl\npjrbmasdillqwdkjfni[lalstrvjalnttmwr]xbezkjpklkrnlpzjjn[wbpwhbukoixcfsqnu]xknhkqjktuybkfnz\nykvyxzavfcirelraq[itraxkxjwslzkxkigcm]ndbwcybrgayecrpjao\njqwujyllrskoetkbz[akunxyvvaxrysiygb]ynqqotupdoqbfwncn[yyszfaxjmgqmwxrvdx]zeacfwrreohtnzvobhj\nfsfgewroujqwaek[mryrrkeqgtpibzn]vlmavzfvsadxbdiph[tdlovgncglhaoqafic]ziupjyryletstrull\nfosmjgkqrqvjjigrtf[ejrefcyognxkuvlwl]bzhpufedodqwsztzng[rgxidklqahcldewgfrl]eodokojqopkrrhfpmmf[yqwaeuztmjkelpwlj]zijgacsyrbtwkxh\ncehnutkhbzhfouyk[pdiacmcgcdpmsvgvkmp]uaslakppkycqbzn[ldbaomdftjcnpasl]fgdrrrzumavxzlojm[iyknsyaoypsbqicx]ggtbqnjftvmqkmiu\nnmezigjskmagkzcsyhb[rfrggycsxoxxnxrhyb]zjlrnpgxzgljzfw[ztdnrdocidkgbqmmqa]hnuqryossbzlfaivij[dkaufcpwgzsxztpqsk]tzkdznvnizjtbrnqosj\nzcdfhyoyrbwonet[otdhxcbmwxzgoyoo]kbkvqasgmhmuynqth\nwajbfmurouvueehl[dvyueqwzbqcpdvbjfr]vkujmhhlqbdaqcsvomz[wlekuxdiumhnwms]yzgtuwxfirpmllcek[tzipbxbzpxcvzxzmtr]tynktoelqfhedvavge\nhueffzriwkhilam[zheswsymmryugjawlxy]rptwswnecdpsdjujnt[rjyipvpqzbnvtugvi]xkicvyasotmrxvqj\nrqbhugeaozfjbqm[blpvbvcvrytbekhjfo]twsrzdeuojhqpaa\nfymuqqbklufqakg[wfsqzzrvdqcubxbdr]yzvdgnwitopzvtha[vhrdzzbmubhgovut]tfkcybfbdsxbxaxnmm[ruvfmuciecbfoxbummm]ysaeetmynjhyegk\nkoqhuxoxhzmsycbr[vbpklymhqueodieomz]jmstuovitaskfbay[mpccjuzuqwkhvnzlbl]jvdqgfkbyzaaeaxjfcl\nsbryyigqipvwczxty[ypjxmlzyfjkfqxyxibv]ktqvnmbdtykqyiu\nvivvjcfrqdbkyopqjdd[wkpuxloudonlcsutb]wpcbavtlbxcojarsj[wxihbnghmpfppwqlykz]dpyadzmpvgwtjoiz[jgagjiqugqvjnehajcv]tvrrkzjwwxaswbaz\ntkpkdqijrxmpddkkau[yljmixrzauogowt]yngihfgazktusprrt[ggqtnksekzzypkpud]rxvvuhfakfcxjieaa[spuvyobjexcgobltmk]radfcjxnsgsntezrerl\nhywcvnclwvvcmkdk[teiryduhljxirhrjbt]brkfilaybgtdkdh[zjqmovlmzogwvfmmi]czmtshoirukgjgeug\nsdbxirgqauygushqq[itvwniqwuzmpzqbuug]dnrxseaisdgklwodsgq[euqpdyvpyncxocy]ggchswamymfpxaiap\nnzteyxnakzfebtcszx[uctynyhtavkzfcudvke]uasdfpeleelxacxq[kyqsinbcwbvlrmr]zelddmnaqlkhmbsw\nttzhosgzkuxfwsy[carsvskefzrusoihqw]qiuobbcgndqqukuvbmp\nwihzjoazedelgsojb[ftgarhsuahimrocy]umttbzcrvgzroprh\nitojzylgycblvbao[xgmeltpmzvzvyfnso]kuohqnawebyjdrerwty[oslthgekjbgpsnkyk]jifnogopgpnkfdrwi\nnvyowfknauliiht[tskhxdgvaggvgsbk]blgylrovweecglu\nhvzpbfqqlwjennnj[vnmqrqlfiqeqdmg]hfofuvqicttlcxka[ievkgdwazpamrdzz]aoofvzixtqamcvhbh\nyuxckarjmwgyvqjl[nvlegkojdyybpty]hvkrieawbpkcjit[tewpyncidhvdtomjq]dtgggmzwogtyoxrepi\njobfkxxyhcfvetxwuc[nreuagzglpniuwkvui]seztmibtqvrdepqyt[skrxasyhbotymilzgzr]jnhqwvcpirmpnltnyn\nhoqhdburqwecnzksmd[gnegphjoyuvflxlujbs]zhuvrcztcfgorbwuc[pjxxfqyqmnhyopaeh]ewbvxrexhvdawazw[kbngpgqwtgkzuwupwj]kmatbuqigzqrzmbq\nltjrhusfbjbciixg[swlhqxnykjxumuifqdd]romkzpszqgaflgbjpsp[lbaqcvazaucueltnp]wovkfmiuwjdqxovf[vuundonjprqrxakp]wxeulnkckdufqjy\nxkdmgtutsfumpzteeh[yvkilakqbawvedm]dwwaexrzzsyjpzsn[pxitznlnnvnjyrs]kcnhpbkzicorrgncowu[ogyvmiykolbwdtv]vjaksxdrtpuuyykihe\neyzjheolvkemumxpo[ipwxnrhyldvgewl]zbrzwobnthndxxvthe[gkfleabqwkpjxbtdlt]wywjazwwxwmuqkpwj[omgsyntzcnhjvsu]asknyjsgbofzyfte\nkxxpalmmgdqwahfxs[zwafxcjjypzibafhrag]qfnbakvxozjqgbnnizp[bqhtnoqzctknrmmh]zvmyctoitshakgx[dzatbhonulhknbio]eufzjykwmqoignzm\nbeenkdmzqibirws[majntndkzawkbfpi]biygjiawnioazizbt[yonbljzgueyiuirtv]umjmhspfocrpobmrfu[dwegjekvrmgoaqc]dorpbifeqhmtglavx\nsstlfeielfmztngzpbl[alzfrbyqiqangbkwi]qcomrirvulgipuk[mdvsghpkpisxplgit]aykwuhadobubmrdtvvj[pqdycsmawculwsz]oemcgayshwppgbwanxk\nqwhfnqzudzysqxwebj[nhsrdvugubbtuuseux]etcjsefcsjblcjgshh\ncgagbjtoxvwwqonb[crbqhpfajsdwtudybm]dquyiuqtarcupaeujhk\nqjsqqlgdczcqarhftri[rchwsuodsdofjpd]mrpwnlqgetejijnwnr[lwusdojqkioapaxwc]ioumfyxtwspuyztz[dgncyjfldlapoasebgz]raelsaeajwuhnabrgw\ntihnitxxkxjvudnrj[neqbqspcfnldrna]qkkcggwjgejtbmggemx[ffhkzdeopnhrdfpbrfn]rucxwfyfiavskfahg\nzralvoiqdvpvjkkf[ttvdslqoxnlvnyyskq]joucwcxixdqsagu[tulodbmorpbjnzz]qkknyrgruwgrgupgb\nfgfaohmvjameqyl[riumppkgphbaziwbfcn]gspevtjsfjazlolblh[sueqarjummrmwdgzsr]szmltztnwpqshlr\nlgcudszwvsooaxhuz[wpnexmkikdsfquxleu]icefstmmxwsrzqoiki\nelrybwwbktbemldjqeu[moigtqyrbfwcdtjkm]cfquoomooaqrsuomty\nrihnsvwngkabincos[hrafbjoluwrkoaqb]genyvelnsrwqpljgdf[ytnarqybnwaeawssx]bdhppadoofmwwbcbl[acnqxbqukongbge]tptnvsrcborwgumweyb\nsesxnxaikeytqds[groytsrabjvakklwp]jzexhtzpseseauk[sdndnglavrmhzyjdh]mpsxlaxqnazayppc\nozkfwwrdoftbpnqwa[mvzpilxwrdeszungggo]fbjxevczxrypzzegxmv[zvzaovlhirczrlwnvk]yulsjotokxaurjibuk[hygvqlsqfygujup]ijtuoskhnrvxmmnety\nssoavardlqlejqfndz[emljlpogavcsyvavr]izdkqsihedwjaxva\nwixidnoyhmsiuzwbm[jgqpnkzbobknrufgif]yaarbsalkqgscyv\nhgcggfqnkhbjlhhipc[cgcrrzyspqlllhee]czfvtkjhfgnrwwua\nggnsczivqxwhungxmb[foslhzlzqyhcwepvhga]qgqnwrpvfjilhnttbv[uhuhvuqwbxsjxqbmqfs]pvwkiufdudmyabq[ffqrrfjgkmegfls]pvuflwvnbnllckrmdas\nllelndaczjibswzoaen[dzvunuujhpmgqdyond]slkfwoyxpgohhelexsl[hvtucjohyvbuihbonup]mwatlwbwxntozpiymy\nepjldiafxyinaljee[zfgytlqlzoaauszrn]gvyukiahumemeqnsy\nvldhkwyfpfssriaiwe[yuluhcsjdkyumyhnd]wggzcfalpkmnsudzr[qisyeltbpzmkvqr]kmbnsrdjgspckgmwfj\nqkxpyonwbsteomlyhxz[wdkzqjywdsbiccr]ojkvswlubvbbskvnbdw[ejvtytntukhcuuad]hspfdjitkfetytyb[hlgziyjqrulvyaoco]rfhwusvjmkzkpmjvrm\nlnmjprwzvaboyyobux[lncninvpqfpuaswssjs]vodhkkndlvixtbsdfph[gdufsyhihlynxuluvx]oyczgnpmusuvligf[jqtdbytmuyavcyfaia]mcdloputyodiezffqpd\nawulgpuvbkountidkgx[rzatlqccygoyamniyaw]zmkfnkaiuzjgdsxd[dornnqierejrlxbitfn]qyhlxykziurpdxpz[fjaesxiowwxjvoxzq]oujzxyreqtbosriwkl\nhcycycsytqzpijy[pptcwgiggnlhewdwfa]aqrsokplrsmbzzovz\nszlezpesytqglub[hlmouktdjtcglvvb]wgcrjqyvabgnnirxs[cafdqrjgmugvsjarx]uomjcavfgggsyknjge[syhraisenfpvlekk]voyezwktjlqoirx\nltjosfxwsqmgdrnpyav[revxajvfbpuqqscgxb]pnjpsoikmxwrpbk[frqghuqvbomoddukohb]egfbhndnpnlxjhyv\nydyzmmgkrvbycjgeheq[xmrcsrshrtogjfez]vberqebkqhindvsj\nusczwnycqbxdrcfr[papmzhuxspnfexyr]pwsybmexcdgfztkc[jmiatnbqkxmarkaeer]whejsdpzzxkdxgwm\nvfiswfowhnwcuusmd[dhhjzfujepawktlh]quzyrwoerrtncnnxup[ekhrriqhoudhiwiju]exzcmnyrtbnxlchf\nfmobpaevmkephhfuu[pjbpnzxkqpvoafxj]ickqqwfifesukyx[uzfultsftvuzbipz]jgvjewotmlkzqhvvc[fhfgcekzgmgxosyuac]gwbmgqtvkhyqidnehhy\nzbwadipvxkyqwsaassl[wcojcviexybrfhdfc]euliyskdckqzozfnlpn[fsvqspcvigzxlzya]vzabwryzpqlmvns\nwavahkemgrtwnvbocse[hnzvxqcxzisfehcy]mqvssniqlwekgowu[cusnrkcbwuichekh]cfvncmjjykeaufknu\nwvtptjerlrfvtbywes[ciopqzpfjdoclfyxxqy]sleyhkequxorssls[weyxuuiigtkjsmnugij]onxiowvkwaaycpv\ncsanwgypabdqhiinan[gujzhrxowlgejtk]mkczaemurigewvqw[lsqtuuxcsuphogl]acfqrkiewfykgnx\nennvxqkaqdppzmj[litdmoukvydtepvji]hfuqcwyuufmxcxy[bilbdvnquchtcjquymu]yjndoqqpyzrjudd\nvhkrlicuffddtktngy[opctcwvtlypwglpaoi]iscxtzlmlkjdgty[xadnwdasnszzmwwid]uijlqxpfgkkcmwga[ykqorpoxpbjkepibk]dmuojdumobwfmkvqg\nwgcihfnjvadtczgqbj[psdtqjwifivgbhp]ocykhmjfvbppiltqpvv[ermpbuyieexqujuiji]vjioxemsjslsdxso[bmsocpaehaeadsaqzbm]hqlzlnedzwgbxbcacf\nreesvrozyerxeid[ymtiurpepvrvnkf]thobixnwiqrdkih[uipdwllkuudcydjinew]lzpxeltetaixzfjxvf[ewlhchkdiewigxy]wfeiqnngnifjzbpikb\nrxgukabwlgxzaxjxch[ljrblzdmvcwcxdoomq]ksidvuwcwvwlvrpe[yrnyjokakcbwdxh]nertnqwigrzbtdmj[gxbsdsdmishqjeswt]dsgnhlagonywspbr\njjdfvvurvfljscocvr[ueywpzuumfihiocoe]lmcrxdlkqsouhpimc\nqgelmqtmcfsdugg[jpbrzcblivebxazpamj]jpkxrusyqkjnndao[nqcxhhmkpfgrcwhsoyr]wvigixehqklwvrscmz[xutrclaofzczcvfnxll]xsyxrvfnovmohxfbt\naqhrsqbyxtxhsvmnz[pfpclhprjghikyngp]krgiznxuehpzeiy\ntrqnrkulbvipvmj[mgsdnaqnayymjyp]otecdnzhhcufrly\nillmnsgqusbqybiso[fxddafnnoholnqjotb]uplvjosscbyhwmw[jsedsarqbralzbjmyq]sdwkyeychcdpqvfup\nzehmutjhkodiqpi[usuretqrbmggvlvr]dewkdjmtingkzuyq[pmmbbozcvplhejh]jzasjfqvsusgnkfegad\nljpcpqtpcpcdttjo[qbmnhadshlheoavsbxi]wnwuahdcagpellgs\nayqxaqtrqzbxyhu[wkplzaetynfxqzhtkco]jpgbztbvmojlflc[ojmgjvfxdvlyzih]levvkelkzftbzwzkow[fmszxqchzjhxtwfm]vihmoqcosarkzsad\nnigshquyfjlleujdtw[qmiqiabzqiqafambcv]ywbltgpjxcwlkyahg\nvmgyovkavazsxwed[anpflkjsqieufhscn]uizulvgasvsstuhfn[ygxgsfldybdnsleqy]tztuatotreocsrfevpy[yxqmsidajmknyrae]whoydkufyieuqhmqv\njyhhfbftixtntuozgfl[ffrzhxpaezbspndbo]sbwvaoziercfpmeo[tzeluvflupgartnyjes]gqfmzvmpieczbjdsr[zeenwxfhhxbdgjkr]ojqxbcxciclzwthvqyv\nolhruodhjmaicslbgw[upvujuuazyolckot]gcwfjukdneuxqreeg[tnnnlficumlgwkdsxus]pxrxdntakudobpo\nvdowqzktnmpimsvok[gggjvxecgicglrkuvfb]xtsuhbzqpovnoqhnbs\nhxvziijhffbzjnjvgoc[sealjvjgnjnkzac]neuhdwcgtjcvpku\nqryaqhtnjvickffebwj[hcgzffksmwbqqdm]zrwihiolnfuqzqpkxn\negbqexgeqnqsaxdi[xghkrttlbmkxgfj]rpulxldvweijplm[dldqxbqxenksncnwhxo]steqcncxfskqcfwfnbm\ndhusxmzjdacdrqor[tzblogyadgggzbi]vssexeogwduosdoeo[xexqnjrctzlbkfri]dqppelyoecnnacs\ntkrkjtgdhxdcyapamp[gvyyiztulksqxosp]voudpakpaphmrlebpj[vghkfcrqexfgoguvbxv]yronkwfpvrwilnuegkb\nyiuhvglusvqtzvngzuc[mfvcrgjuywuthtprxe]vjrrmtbyppmesvorp[ucqdvtwolrvpjyhiolf]eazedskopeknjcqx\nsegabhonjryukdicj[zvjqilxyvwjnjgjvrnf]gxibvkxslgkpfdhsn[tlbwwiypungvwcvwngx]hhgglxqosunhdvgr[mrjgltlfxwsznpnmdox]bqsgftffsibfruyz\nhrtiuksavtjzekgf[vaagjkvweeznlshs]ntotbakgpxpcmqanhab[pqvkabybndisouur]cnjoxldhauoppnqqk\nyizxcouxlbjqbijqmj[kkqvlcusdkmkbmuia]pidiunjwlkapojzzmf\ndfzinzasgtnjdbdh[wyguangjweruyqm]jfpqpyqydvbdtgqpqt[eryvzkaxiahxekwbp]sywpjhgufixvhljk\njkmabkiiltlvopaxec[utofhywhxjucodwke]dwxatuzwebnyulyt[iajptbioysozunsws]nmfnmtguoqipjmigsyn\nyxletutyrgisbrm[ljtuifjmgxupgerhuhb]wpqnfedngiollocqbfh\nzszqqoahkvdvpezddea[defewzqptytvhnpzcdu]cxuavzeyqysdynnr[gvmfnqnjwrjrjzphei]pelrqmmykeiamnh[jrjqavultdjecnghoc]ekxawogufyfdmltveqf\nmorsvbgrpgqiqeplgg[giswwkjoxkgkbonav]lyhrrcwskwjjflawgs[ogjazoccoomohhalb]gjnkzumbxtojtud\ngtgotbovcctgtwwc[owthnyvlmcwnctlkilj]eytxalpmzywmwqc\nikznlwbayqdbhusm[iqstwodfolztyldh]amvvpwqwlswcnut\nkumjpojktwxazwtg[idtisckrbetbaye]mgqtwjxlbdpadrnxg[eourfrbwgoeoqrlvhv]gegegzbxfyzpbij\nmxcepmkacvzxddcpnsf[jviddcgbglreegewbj]qmqdhescnuuswkhpvxn\nltsouowwsvovkbie[huwwuaptbopxsixrb]skscogxrektbbmuwqu[niaczcnnxkymnnuu]sfczdkldegoynqw[mrjssleiutncang]jkfgyuzcaisvrjekiwe\nmfqowsxqmywlvauv[fziifhafjuiwdizvm]gmaxzryznwavsaxsv\nokmehkbnqsegqinj[dxddmmglnqftiunfuea]todmrlalqdfqfkbq[vrktligspzyclnfz]jwdvkpuvhpwffrnyxw\nmybozskxkccdsuuptc[mrlkqwbdhhktuxpzjxi]xrujoxxkxwqcthydsw\njupphmpmynzxsfkr[xhvcemrobysjizesgs]ijjlrwbpchbbiblvr\nvpabzrcqfzsejjgln[segfzwfyprsfqskhop]gksthicdjyagobs\ntuhzaznrumhuwud[szqusyzaykegklbcdoo]prwjxzrwyrgcouehrg\ndfvbjgrshvnvfumqxh[tgnhpzveumwngrnoc]qpntyvcxxoofgsk[jibdpycgwklugip]mgkzhcifwyzxsbuwj\nmbdpghflpcondfk[ftzfdsbexmnznqqmfaa]xznzgqjdfkmjzvwni\nojjaanxihagtezp[pxqpdgygyklexhrpc]lapqmhronwsmwbbf[rzuhtemugsniacn]apixdvsnjpsplmjwvn[iwdpiqgoztjamenyyw]zjyidlwjbvevovgf\npijmbdkeyhcjzuwclu[onazufaoibbwzepmbr]jhjaqudvrdoqcvobs[lrwjikvojmgdtkwb]gfxgoeihxughdfbetm[yjhxesdcdudwszwv]hgfdxuejwfuedpdu\nhvdutkvozvxwpvx[beubpipzuwaclrev]lqeylkxqdqmcdqd[oivjrkpjzrjywzrxely]dcupjtbrltnguho\nesrepqjymnodspvjib[kwdoleplnoxmntjuip]lvrhqceegktadibgh[yfbqpomfldnbpxsaoan]cheitjzmqwdbilm\noakpwuuoizfcsfo[csxawuixxvzzooah]dafrurtufjpuetnui\njmmekugaastsvdn[qoasgnykbkodsgt]lmfvbqomdghvicry\nhqznrdvlwnamiushnou[iufqiqjtaiejfqwns]xsgjmqqsvbctpwqcgz[mvpdchozogazbfywqd]iqimztlwajwbxhr\ngkeetoqftvsdjhhghre[nspwxohslbgkpyyhdh]glknqkzyfmvjczau[zrzurqfppidpckhmxu]rtawnnjhyjnbvnt[deisyafkjnxtcjas]cshchafpoiqptus\njpkjyjiucudsgjz[mppiltmurhwxvmv]sdhrapccelecuctxq[cnwlmuvyistotoykn]hjzxzneifkwmvumg\nuvzuxzcnipyfyuesvna[ckplomuathpfkndodxk]vrqhbliixmzbefuh\nionmypunjczxhry[bvgmqzohimrjmijzkwz]qfzsokgukugmeso[uarvxrewouktpgnghtq]rsnccdtstsegeoudngq[hkvkymbbgdyncilyf]zteoiyacrtwykwzbxy\njnyydhrsrkeujfvj[qmxzqkbwizhvcztzdqr]yllidgevuektldszzjy\nnuylrchiwpfvhdumyet[hfgfzmeldvotgtxqh]frzcopyhigfewcnb\nsdcvojpgatiidjvfy[zhvymqejqxllelyux]ektbysjcypxfjrsor[kgfvqbereoskymyfp]izmdymjhwwtelesjr\nxnelfgdpnrfhdombqq[oiidietkplqnygwsgo]jiltmfqqavrjrvyui\nzyuubhwaovcbnaxrmtv[yefoksxqkrkbmbm]ainfhyuonvdvcyegy[nntnxqkqdqattwt]tcrtyqjhokntxcb\nhxkbhdfwcraxhdcff[umxxccphsddzavdqn]zsmmtgneghqsrwfauw\nkbdughqnourxomuiab[xcjayouykostteh]enwbjtpxpyzaeuhuwb\ncpmzhwxdntahvhl[diddnwirsnqchwr]etsizyoarkawzrpfidi\nxrruvcmbmigmutacwc[owhorlqlgqujvhos]iddgaukpxlielcko[gawcwcvuviuohmda]bfdceclnseehdeyxv\nvlxaputciirctva[qgmwpinixdixaiut]kkoousbfcxganzcffg[cikwetvrztjgefpzsks]jrsyfxydznmupwapco[ooydsykpjwakdep]krlytknowykzzqaafou\ndnnvcszortmitfv[sbnurvnwxwmvbdpawa]ewayhapxdfxplpqudro\nfsiehjchtnyenvmjfw[obnlguwjqsgylwveak]hupypbuggmbkeqxt[ljxbmifxgorvriaj]tkttmzairwztsmn\npnhgjwzyqnjrkkw[ofyifgmztnzelptkwho]cgnlnrfdgfgjvztpz[wemrlhyskboycpdbzr]azikmfaudvrdhvfvt[chxmcbgineaycjiwy]kjbfttnqgqhkefoolo\nkhdlanelfapgxqpspe[alrgipfwfdyguqtk]coxffjtxpbqmxig\nsxobbewirkvducqxd[ubfbqjccnbtkwpbxqpg]hgsswdjiudnvmvijt\njzbqaqfubdsfinobsdu[rojkizavtvueepedxw]lcsyjeoyieqjcim[nszibgczunpslecxo]louacmgeotayemh[zvpjwwpeyjjdhjc]jidkptxmhccryujojap\nrrofkfoljuossrced[ymvijcmdvrzhcyh]zegkwrmeneexpcnrh\neniwjwjnmgyzescoz[semlscmtbagknxpbvte]ysqfgrshborwtgnwtr[bossxfqcyadppdflbr]pyiuttfsuegwjwcxzr[yaymomeitxwdfvsr]elhifdegwfstqyniqta\nxauanaojjnhdgcpuwwj[ccitjseyrwjqvaljv]ebbwxnquaqlhgqjsgwc[jybietxintbtpzncpw]wfkwxwffzxwqucjhyvs\nipmxdranyxbmwlo[ueimjvadwbdjithwn]ifmvlcsneopyffsums[ejornegszbqxtosc]iucimozjnkqkeysden[vvtdfnvjnzqbxujml]klrpisgrmdbrqbupc\nevolkocwyejqtcazj[dzleqjleocyexjivik]zmvqrxiqhsjtoezm[sskndhlmxrucdyqvop]murrraduofedtltbtg[kuzqpodvwnewwqdil]otvalnjnbexltsbitwi\nppqnetrairzkzlt[hyydyimhgzayzgnxqn]lwubwuvowsyovjjfgp[xbzmifaqcmpyuev]wtgcnccsysrfvbtb\njpecpgdrvunkjfrp[eevsiosfybfgdgalp]veprfliqlxmoctjx[bcfelthvqqxthqwpuoz]beufleuquitnnsti[aslupsydyktxgqsolq]gctlsoauflrjprdn\nyekfawwakhkqvpqf[cvenkdpepuyimstwmnz]fphlenyhtsxxeyst[yohciybbsiokzajcwlz]vtqcjngqpamsvrchix\nougrpfmoohiymnx[gorlgyciageugmcbony]ozmvirifntorlvzz[klsgbagukrnbyzsez]rdzhlkpoucggkcdqm\ngfhrcutoyproiww[nzgfaaccfrgdbcg]fcrtnobfhhyzmadxjv[vlbueztcxkkbufljse]gqpnxtlrrhclwuaj[sstrllihglystknh]alxmlywxfjwnynbwfk\nopeacxklhjwcefmwrwg[mzqwxyfltfqyepcgnym]cpziqpjettzcnktrqi[mbnwwhyxebbececc]tdkduejetkrqwoxrsoq[ncenzwgjnekbobv]yxhgzizqxwaihedda\nsvatyxdgfofrrkiksjf[mxmrficzxfyykqekorr]qojleucutcqxqryi\nprrhfrigzcmemou[zkhokevqzcspzoyt]tytqcpuucppiwio[mogedxwsflwocpkdh]kkqnructlslbaked[sslztcwiwkudgtji]djssvabrpmygljeh\nbtundrdlcsgtilltpue[jiunnaqqzfgxauqjes]wtdxsfqroorcghqk[qvyzuidvkzmomfi]cgckuokezrtxrgdlo\ntjcpdjzfllhwugiy[vxypwowarlatqjlwq]wnpwefpgpfcqqwwrsq\nzfduowqkrccccgggmbl[iwwfgrhmjxgljwqf]cminvjjyetivkvhvkdy[ismlcjjywxxvaehvhhm]eojlvocbfkftjkapzs\nhzkrcmpwhfnbwlisg[wxwoegwncugpcfwywxe]voktthitecybcfpnz\ndcsrtgkbstmkwlzy[pcnwmgmcmpsiyizqx]pzjcivraubvgbkdahk[yydvhvyumdzfmjuso]bfljbkwodikjenu[toxagxhnvgkwcivpcuc]sanysdrigussqum\nlpcxkqrspacyzrqhbhr[vdcbkamwyjnxpgjpm]afxbzzxzrtaacbypq[ftbpiplrdrreqesthw]tidlvfojrlctjkfel[iibzklhicpqjvzrnza]bmekkyjigxxtegqbait\nduchvjohwoouxgmmxds[qscgkenygikbdrsqc]iovrgoggtgiebylbu[iqqrytrhujzcywwq]ybgfnnhqwfpfios[dryqypecmskrqux]klqhpvydovzggsqo\ngwgojmuthbgcalzvdxh[njicnwbqdckxtyxkj]rwyptcssdkdqthiydea\nyokzqvwcycvjgouoyw[starlvyjnijeacjseo]iehvlergdbswibmzci[ppmriizuqubzfehcz]jartjkmqzngigjvl[izpxafhxdmckrcuufu]pvkldotwdzdluoubpnm\nrogyxrgfqivkovtna[xtahrogngfeygkasq]kpcpvtirxettedux[cdlnciogkcsaras]bupwazalrmfnjufn\neaeubxmpmymzrfleut[eharpivgddyokps]wimaximeayrixnts[paysmyvjuzpjjqr]fcqykmkzbcbyrpy\nexvlqvnfmpkxfjwbhol[utjaefsandulqaw]xjrjchxifscadbld[ifrckhdhmptybkhrj]ykcqgygngiwzzyfnxg[plfhikkzndknbpdeeu]siwtfnlbcxuqkrhwj\nljihefaqagbmffbcr[ccmafzhpsvluglwsgh]jioaeefkgujinzlgn\nrgysyaquiuyvtojxnaj[gcygzkwqdebiqsr]icaeuutjodsizqzfvj[qapmsqsaoniuinsz]ppgtfxsblzgtqtaiiey[xlkzyyvcgyhlmvnzrpr]htorgwwkbhasrsbvemq\ncoiurrjhxxkcplh[nkusmllwtsuddqasyc]vyxzujqohjyctyv\nbriulribegnliapcimw[rgawfayyoopbosvc]owgryasogyewgxchxgr\nsmseegsurmfktgmefhw[paopyayrwykwdvcjjhp]byayaatpurrllyzd\nmvgbtjdigbhhywarz[pfrhqtizabthnqrvvw]azdztfkkfizbxsy[jozzjtzkscklmdt]ucnptpblgcgmkeojpl[nqsybfqdphdncqgigis]yecpixjgagdgkbz\nzyuzikehgrfaztne[oaxgeczbaafnottqg]kuuggppqtgrncptm[tcfnyqvqcijfcfdljh]pwntuaixpqfvyoatk[mowgvynrpbvmqlpucq]vgopzmyigjbqlismti\nostutlkruoevsjr[qnvqsxlasjyrdyyz]klwvhuhmvgrlcdy[tycmevukacjlveu]mvxcfqojmrijbubfm[rbodtpwkkidfrnhayj]jsbgdcwbfdfflvupn\neaiframmiukbcixxi[bmqaglfamrqoswuhme]lxvkwmzgauwmabu[kxusdngtifhpmplxl]sfccogjqnblrahch\nhcjmrcnzrhznwvtjby[lxmehjbnudevzmhx]ukfmdplzriyztnioty[lqjesrsxjozxcgfaknm]qifmjftfaswtrjblzf\nxmhpeigrzvrgknc[drornrcakzujdrsbrvj]czapwkwkwwnkwks\nsfdyqdpsfcxebamsf[vehdpjffaqhytqhhbi]urolmsuobvbecvcnv[toagfgryhwfgfwxmvs]btjwiwdrxnpzxlxdsdi\ngnjmrczrqiryaodop[etlqbnstgjysesf]ggmbohbzrtfbapbjg\nwwkqbdcmlkfwxwdu[firsfuftyxwxpcicu]cntzxuydyjkgkkfvdl\ncvcsgxflnidiwtvy[hhzzbmygwugzsfnus]evzlovhsgqumejki[btikqitubnwzkhfyhh]xwxvlgyojlmkwljv\nbzuxzgeuobcctajvva[lpqpidtuzmrrnnlgkqu]lhyxsevugkrdimm[umbmngadfcujqpqr]nizwephuepdykbgj[hfheiymxxfgyxyl]zlurubnhkwxdrwllatg\ngkwahvrljkerohucrty[lgxqhorgrscmkjqcziq]otxkbzuzncbznvr\nhpoehzfotnjpnhl[yrkyqbolznetbgxmy]fblwkhzfebmzavscyyl[lxvxgdkjvtoxjpu]oetusxkoxlpceierbt[faylwjcdxicxbqr]ledknznfnaiaovejww\nxifdyajgrrrhakdqhg[qtzmwfjraqbrwstiibr]juciognmzyafmai[lgbmgoxqtjngqpqkwt]zzkhrunuborvoajlvul\nekecthrkwdbjhsy[klxbdnucasemwhlpjj]jbvenwrnvynlfyjybm[zgfxxurrduhtlmsbelf]lxuxlahnrqvjssffj[wzcpjiesgsbwbtnlrs]sofzsskbviyfvlo\njscqvqqdwvkvrqcb[vzfqbgopfnjcekjs]dmspregwlklxptp[lsxjobfksvzwshdre]yqfwrvjrykinzeon\nrbtqjtepvufhwpjugj[vkdhjmfkeocnauedxp]vpoqmfpnmjdpcxw\nihhaztfuasflyghkndl[vseslcbeufhmrpyfqb]mtcgpfjhjeowjpqc[cabeopcrmhjhudob]fgeutfapismkdwqxmal[wldzeajldxlxpwfrb]rvyuojjnauuitoofgcm\nixrzwptyltfshve[xwlsfazypzeuauxpozt]nwfgkbpuxeauadrgbbm\nvppgbcdybisarvokztx[yuykfmzxbgfwzdohup]vlkdreyqjihmdksxih[iysfrpczrirzbeirih]czkbhrqlrovfkmlu\niaatwbohmiosyiqfq[imajfecefyujhwg]aanaybxebrfpdfxxpgw\nqgomsuglksqobwhaq[fzcrputgufyvnesoqwe]ipziztlrfmlaizts[pulgtrdydqegbymu]pxcyeozdofdghkmst\ntlxidzqdeqchemiqdsm[hacfdsanbiffzhilct]jtclxgjapfmwhlkn[ieafoftblueqcped]lauckblqborgtjnj\nupkkaykvxwvkgwgztzp[jmotfixnvoqrpwsci]wszntutpsjljzmwqpgp[dbnlosuwazvekoplb]bmobthbbmitprffl[qkjfwmsronqjmylzcre]yaulmyfoixmkgjs\nzxxsmidmqxjigkbos[iwsufumylphrhyx]uqmpbcxmvhzuppxqopf[ykipifsdwkpzgmt]zzcwzmwugdzckey\nciakjtvtrkgrxvp[yhxuyhyxwytquzxujw]lrxibndatfiqyltehl[nnadhofokmcutiyc]vosxtisllkweiaapagg[vwniutthbrvmqrvik]aixaxvddxrdnmmt\nmbjsskcvljlehsxc[cknzgxghehlmats]eqknrogpyfcmtfhso\nlcbrfrsccsbhyhurc[mheohludmokwwjx]bezowkrdzwhssgbvydq[kiwqvuebvywyegmdyy]ioskcrvqcagocnnh[zgttakbraxpcsqsc]hmmqufyflbmjlcciqvn\nezmqplezxylckxcqjxn[pdzarngoyfbjgyxqxgt]yokricbfoocmehi[cffrwwrwhmilnyf]uaybztxphgccfuu\nxnjslvbmmapiwwpq[qmuxemavopeoiwnebts]xmrajpgpgeojtabumm[tbjjrgipnfzjafi]hcuirvleolclticur\neltfnqblogwvtjgni[bjfxnnmgalahvpdtvku]eingohwswwabsbtb[nxsqsvleqobfpxlaxj]gfsbsvcbbnwtuktuw[wrgcswhmdtssvxobcu]wgsniklaxmadgnjd\nkxpuygixzfwrwzpzsbw[uqxqvvupyvvajkcysh]scshpiffohigsgm\novchugxbmthhhijq[fznmygfcqewzomfgbc]qczlousnoccgyrgs\nimtfinjttxvhtcll[xiqmbmrcqdxlvuf]pybqlwqezwrkvikns[usjydesemedszquseso]fhcgyicfbdrmgcnk\naqnavkllyitzewgs[cbbqmbtgufuvcun]iugpkakfufksfitigk[lyqiierbjucxbvaux]szbwsttayzipkcdb\nyetucqvgffnvnxqx[pvgczfwkehnfqxawz]vfxegwcevafevvzx[ukcwxvnvfnqvxhfa]bdciuylrvfkmxyi\nyvachrqguvjhkrbe[rtlpuvvfdvmtqswiln]jcyqjdmtzndhrif\nrphybwiwiszwkkxm[waiaqtuthjgfgag]ttlnqhzfagaregyo\nunsmoewlzxuguuwu[dyqsnohyqcommmmov]jipyewobyjdzkgkgo[yphyanakgkgvybsx]pjtzynsvtltzzajc[iweuafprefmbuekk]rwelzzbkbqjwjrw\nkluxazqhqmcrvldfv[dbxzgwsfmxettwmgj]rgvfmxibxzbajitnud[vtlbsgrkhnfpmvvkp]pdycyraaqooszqa[eyliotjigekmtov]eiopplzmedvdvmwt\nmlozzkwmfcrdlvns[wsdduzxzfvlvldpjvgg]ywqncwocnslofij[sakivxaniergaouc]nzmhdlkxeiehdpuok[zfwtadjlizjcauurkq]vlvtdicnyhseqbeo\nssfmkfdeguuaqdbyqub[nbobgowoboytefejnz]fplpuipnficejfsuid\nlljnuuistrsmsjazzy[vccsskujvdwxypuk]jhqjqhfatmuedugl[hufmsmgjutabctabusw]zcoiiovxkxtualjx[zdxdbmbibryrqaubxy]tyayojdxepcpmwi\nzursgksbdkuzemouhl[sekbvoxwlmumyrdh]yxafewnovnxivyp[ajjditfeeocipuvdl]ygsuxuhtqervumd\nsuxzfxizhyzbovsz[dtamgkleqiesxemqkgl]vjuviztkxzchergyx[tvazaqnrstjbdts]wccoiceucunjiuus\ngongygcedfxwncy[lxtpoagiqvgiryasha]elmaiygycycdtsclhpf\npkyqsmcicydbmdagw[ayulcaspxpbtnegeoou]welxvngiualigfefv[veqtcxgkgzveegxckee]djmbhovzjfexqaedywl[okzphpgdqtpicit]mistlyyaoyphetsxqxi\nuwrxhstckbebnlw[yhflbfhsqhshieo]dvmzzqknrjcnwixhgk[upxuqrlwzvvsgpa]bmnfpjynunfbwunupiv[mbcmrpoxtbzcbijmmu]icdxewwtwcibjotjf\npscqchwjixrhpzprdla[nzfglspgwpsaiph]xtypkrtleiujsfmcso\nllcxlfghzjvyhgill[vtqyiyrwujkovfctkk]arbtetvtixtnyavydg[ozxyyroceqktxhpv]maekylkkwdbgwgug\nbzagcsgcadoffot[demvhzpdjthrniiuvj]nwwrkguuemsdtvspi[sququtlqggtpszucm]pqaqqxpssdgniycn[lkdwrbxkrkiqdxjc]bqngsdxlxxvxdvqww\nwijjgkptnkbnzpqr[zylewxhygsxcrlyi]nanyoaosbxahyvdsett[kojrflwbltrombqxo]lfdpaptujhwfgrrnf[slsmmogpspgpuwnce]sihedfdnqnejevnw\nnutyeltkszkulqpt[cpgdmqleitivdtr]veieyzmfjafragrcht[nzudyhtmpopacznkq]dmywgwmnrieiohcuf[ctbktcgxznhoqoxczzf]bqzffvqraxpjdcvt\nakgmlcznqnhncjknbp[bwdbsrdxqqmaavngjc]cwyygvcrkagmmrciout[nkpzkdmflljxczogs]mqkafcpxslquyrudeui[clvbdgnkrjdpptqwq]cyygmkgtftxvsbbbfgc\nfxlpnkdskynkosqpp[efnouhxslwitteqrtx]xjxojaxrbampbcknga[ugewjlmzbspxhtejamk]nrtflumsbbtkejw\nvzrzmtwbxwfhyjvcmft[wrdvmieyzckycagwma]izyptswwlzgivtgyfd[jaujtzdzregakjk]cjdnelesxnhmgkqsgs[tjcsmxghgtmstejjhb]tzqsgoiospxadncn\nokgjhnzaxrtektb[sleqpxoqckdrsiwi]jzthxxszazdahvhq[mgxzdqnfscpqdoykr]doyvhvnmbshvkcib[jtrsntjktunoxxn]rmejgievrkrxaziux\nfodknkictemsxiicght[tdltamcatgnknki]hzdspvkbgipuvnb\nxhhmaiussrmwaxcpoq[agyegtzmrcgdrqiiv]akuxocgoidnfmkffroz[lkkfnmgryejzyvjh]ozdzcbsfmllaiyclho[vseayejwmotjhccg]qfqchpalcnaweyo\nimdrphyleudnvhc[lzqochrdcjotjojk]cwsqzuwoflalwatlsd[ctefovkyinrjchrwdav]cmnbuqveexpaxmhi\nvckjhzrdtpyynzbdsad[ehjwlyfbffzszrx]aizjcopfbdgrrtei\nvfkpxnrqufijmniu[wnwtwpmgtjonykmcsp]mhehavmuivmxhdelxa[spyybveheykroybw]bfzudojcjhzckbac\negipucceijeltfoz[jpyjfgsqdywwjillf]kltttxmvrepsures[asbzcnwdqvfkfkiqqs]usnadxpcdxpjnifm\nsvsbijigntdtxph[fabzbljmijzwvjlac]kieomhcpodzimrmqoc[xusohhfobyruazi]wxkjzzpskukqjirtjc[iwqdjijjucrslihqpo]faezwwmpfpxenvp\nsbjgcnwomllqwavkviw[pxekvxjtjbgjuouft]puzjbrwmyzsxclgmqsb[vtpnaljnxkgwlryjo]lhqzwvnpkzsdndp\nfyfyvifiocceoozl[dmjxamblfosaizav]smoyhjbuffpgqdl\ntlbdacsdiavtwucvf[npepgjenhdkgfavbn]hvbffufjyehpsoa[xghicdcxptmipfxlz]lvducqyymcqkket\nnuystaihvpelybkvch[rlqyflvholahkcxw]gicdfjzhwwocfejthx[jpeuakotyanntiw]sfsavxuyyulvuluyur[asngaxekprpfzsvxx]rliayxmjvsrnizh\naxquvvjwulrntbzzf[fddxxjwbdaecbsderd]vjtqwpjlhbdhxjoh\ncgeyfvgczhhwbdz[kgsqgnalsysssiyhqp]wqzhbjvykeuyjxgfzgg[mqkzclianfnifjdql]vbeyhsxsfmoeanpnipa[sxmzlhgrezqxsxzzcku]gwmgkijugjwtutmgj\nnnjlbnnasmuhskqu[shbjjccjlumeuigoim]ndwzzmbtazttjpawtzl[cnkpifihvkmsallifij]ccpzfojfxszmytbd[jtcogseximfojmjm]bgdltwjrqciyqfifkh\npkdqnzhjzcttkackdba[mucwutymaybynvttts]nndhioamrjejmibag[fndcrctykpehoglop]rgxjwrpzlqapjsv\nnccuyvrhzyszqnw[ogdgzsefffyfoenfh]jnqnhnyoyrcnrowjmpv[wmlihztaoyedgkg]vneeegnosrxphish[uwrmezbsmqbxjpx]jgfoinwzlhyixzjzv\nkriqecrnaeujvuzw[lruowheuwnintaqqxcl]kcopdidcqinihhmk\nvxkblgxcmztnphdzf[ysjhxgovujrpagndi]ezgjwgowcdkfcstfhr[hpxrabjwpymyaolp]itcthqpgksvedadl[stfrippovsfrwglisp]eodicmiszqhwnuymlgn\njznqrbdgjcokdqdlser[xemhfhnwbftgxgjukrf]mhcovplrxcsixrh[xyswalpqqvgsvmqvx]kjeuyxksnmydfkakhq[zcaydzhceioawvrlsm]wzezpqlhvwcgzjzigtn\nvedqtirgwrgutas[eegbxmhgykfrwrwy]pzslegjrbmdmeub\nlespviexybwomljka[dxvrexedlclnaurw]wzevexsobirvepgpmt[rseoofjlimvxwro]cyojbkugwdzjlxsqd\nfsdyxosfmlqfwoqpy[mwypxaxulrbjsfi]ghywyebrmgjsrshgc[lggfwxlpovrwthxtlln]zmtqqhkwabuhvtnabwh\nsmsgvpvsfaxhocsyz[hgbjpapisxsillo]qsgxbvoijxlwhxpt\nfyfpxellnptlqfxvdn[hpopfkwhgcbjoze]sopowsrtqgbpysjfz\nqenbpbnrikfrnwpq[nmkndzwogcgtzhm]zhuslfffixielmjaqpb[dtmldnpqizrcbxixto]wpspaoprebgbksq\nvhjgpbgdoeoljigkqde[aqojnqwgpiredyffb]vmlvnnohhbwzouwi[rldlmezoquqcodxghov]bhwnyaxsnyyihhgv[gjjezirrmfvkpvfayb]uaxxuikjcwppslge\nfnwyhfrnoxxjpubwe[rflutoqwauqbztk]tmbmyhpncgpkzcqvv[dgksjzbgbuzlozns]psdmkqjzxdwvllstru\nvnrsujzctbuqnbu[glgsyfmfeuoloohqp]ybhziayoqxsbopf[vtwnbpqxhgsfguztg]xhgvtoqwouusyahedc[zcchxnllferklyt]avgtwloloznygrb\nrojtxmpwxsledhm[xibuxgovbxiejlegyc]xihwoxmzghhwlsthiou[ywkngtjxrhhozglwo]zfncywcurhmsfxxqjbt\nvxoojfqikhnbnrh[trdtiatykaontxlv]xenfwokorxaeweoz[itbylohijtfjgdtmkvc]butficisomglwjzaa\nwkofaduihyxhiyrvjs[deskgjgenvxxxupntfl]ralmugesymrxreommk\nozsnpcdvkykxguzltcp[caargzwxildtwswp]capkmhbfpfmdegigg[sigilgehfnfxlza]trtpmbccrrkpggioz\npfuhqwjjgyzbbea[yexwnbudioaikfsqlca]vaobiurftgeglgrzl[thjpurqfzaezqxfajme]seuekovcvvtdmlixf[mknpvkntvdftjhhhfgh]dlgqajapwlgdjnwybp\njbtzwsypehgrmzeg[gwskjuqbwedzxfcehr]xpkfcuejevonsinxs[upnrxgjqhohlyeyp]dsyhrudzqsibolxnvw\nskjjsxxumbobzsckqk[sqlnqpubrayffzs]hseibigmtjtcgbav[khvlknemnqiekxy]fkzvtfscvoatsfqrd\ndozlslrkuemgbykifp[bzvnluuiqdffwtf]tignkmwpnqrnmefaqm\nppxwcouehvqfwoenqo[rzmtyyvedmojatvvq]efcstfsjslpqdzvhb[tvmkwnuxestqxfockv]oqskydohbmayshfcihw[pfyulawxqbaiehqvmwi]wluhmctgrkjxqtlmp\nuvqfjimhzqboivo[buuulgcbqgfsbup]wqnbktwxwslvceegi\nmuiuadioyfirjks[xviqxaavhdxjkkccmrx]weauetgyttscsfwv[rzgaefcngzklpjqzgeh]jtnbnuuvbnbjhdqn[idjpczmrbomwipkv]vbgcjfvyvnxhdsmycx\nhmdflkjbenjynzdmeqj[ybyntwgyyptizunn]ctijqxbybwarmfzpit\nkhhocslzxicmlxk[xssahaneujvceofaiyh]swrjwipkknbnrrrig\ndvjvkhnqyifqzse[myleyunwsupcnfagq]tmtuvqikqxzdskqcgxp[lblzunblboznidegkla]eaqhztxpgjuijohkdru\nmqcasrzjqmhwbhbuyc[wkfahpqjhtwuiybqae]yzfcavhtmzofqww[goqblpzkmfxynuzm]bysjxjeocperndv[uwpxvnpxqhfnaalchm]lyfynynkovtmfsi\nwnczxavmjnfgogv[oyjxcsvrrgtpkponga]gzhjlzgxxjkoklgm[hsrwppehbugkcap]zayfyoqorpxefqenxc[apojyrhryhfnmksa]uwnuxprqfxnkzkhnbji\niylrycmvbhpowmdvwy[oepptahrmhsoiskeoq]vtqctnyinxvrvlpl\niauhsxbjgxiebvfhbw[mnjywcztqiajiqxx]iikcygxzeprjwkoniqj[tqycczkvsvlsjetec]mwrnosvszjhmuoiyzxw[klgtgkaxohfaogm]fsxjsgwondgzpdrbbcl\nbfqtwsviccqwndca[juqvrcznrlghmsiz]yttbexwewvvoehurkrv[mkugsxdrbaktcqf]yrqebvyxlcqjwcewg\nytoteijopgxfmiokatn[oppmfhkktlewhlq]erycfxfafsiicbtx\nxlwbkbenrohodfnmuv[zarnezgnivnmged]vyumskttvpderhzbimc[hvbbjegwdeeqtam]fopblbizbmbhzfsdnzm\nrgmnnwzikyanthhp[nvnhsgdymtjeqzurz]mbqxtvwhpggnbcq[apeorjqexywhszrno]qaxdcaysefnpyviduz\nvjaljdyyoihduumfo[bpufjkyqjvxoprdwrr]ccjbldnkbzezeznmkpu\nyhbnzbxqrvzrguxcbss[unzjeicvhgqtwek]obuccrvnajbvkcmkzh[futhsovnghajatalva]humwbgtpqzjgordah[kvxmlpebzsitmnjfnz]olxhcyqkvfkqdxdc\ngsojkejbnpgptcgeubr[lgjcwaotpdouravq]neezbmtkclvcvkqncw\nqqdvpngddzjwase[rtgandojrzcpohlpknx]qdnxpiawdlklkscmpa[qtpzakubrncjzbpr]efpxwdvobcigtpu\nboxlzukkqchmqrrpgk[ggylyipkjdmbjfp]dkckhhgapbgpmygpa[yfetxkcehafknkmk]acqmjcsvxzptstswuj[atrjixpyeqordilgj]eccoowxhivjiljegqm\nexjgzzncnnehrto[qnhzvdfprbarmtdpp]rcdxdswituqgnsix\ntokldrsfwqqhetyw[muqzhystnflncxm]pjpmtwcamluvvvdsu[mpfvycofrzebemw]mcyzcqfngdrjaioxzda\npqhnhcbjoqjvgqh[vqkgnojpmbawemi]lampvrpcpvxludprfuj\nvbdpihaehliobsbciw[cpaudttavwxkfpg]aidtxeypckfsagubro[fpaiuhpggzpxsctw]danwtjnlhrbfipgfbq\nbeoecqatqkztrbevt[bdqoxnitxmdqunizj]lgquhovsnjuxqaml[vyfylkbhnsdjoezm]ediekdjfsnsodqep\ncnaisicaronpqbihlv[ajfhzrpysjdkxqpql]dfznlmsbuozjlqvf\njbgsemiqgxmtwmdulu[ulbyoughrbpthdlvmvm]dyrxsdesjjwwfmvmkf[gogkkkefuecieipe]nimswajpymtzyleew\nhaavjxuwhbfxlhfx[rssbpwlffrpnsse]chremerememjcbfuv\nlosdtsrwrdvwzbjf[daaxdqsorbsgznm]miovihloamfmovzruxk[horqrumrdnjorfw]shihudanlgqfzjf[kqkwshgnrpwudohanr]yohqqtcywhqawfhi\ntrrbdodxpewxgcyryk[limhtndawxliixkkq]ivxmixrjddqlmounj[cfhqatncyqijnvjv]djqfccmuvdnsylo\nyfdgkwopvrudzsww[gnyyumqxrftncsfuaaw]zfiekmyvpseaugfwss[etzbbabtbkdtgbwf]djmbswwpvfsowmqdlw[lpbkaarutdlovoptrke]ukztythdiepqgemm\nhuwfnhilneqaecp[hdcrdcipgcaxtbfouo]poacbxvuqwkcilkb[dnpryjlynwgzbrnbc]hxillsnqqraloociaqc[uoyktvkfxkdkdopnbk]qvjeuapououufksmwse\nlfbrqypxgthlyxqzywe[pcxfduxttmzaxtr]gidsxacxodigyok[qyaamzuhjqqnpdsii]apgfypwqjpygzmdtpj\nprkahitlcoynnubnri[rqthrhhudrvryoea]urkuwyabxskqbsyfgm[dyagznreglcdincwie]okvqdhlixssurnd\nqrwefbcelgjgpzoe[aedkjvzurwcrhdimb]eaxqgpvkewmjynmek[nmfyhryoglbtdgq]dfnecedmtcrkfyq[omndbxvzczgnojpl]trcocwxxczcxrvjjce\npphzgbbfbqmhbysodv[znbyvvkjlacgjrwlnkr]iyjpdjsjryyqsoblbyf\nlziqyyfhruzfpwy[upekwttdqzjxspfzcmw]ptdaapvzenixlab[wvsdrswafuftmysocc]ykzygszayfmgenk[mylrsdifhepnnsst]tqrbrvifghuesad\njwfyweiiqvjfkvp[gsmzrlbjdpgqtbjakw]oofharmppecdotcw[dencjxxfrzxbuku]ygflsusvcrcdznc[fmcercvqncnxcbbwcrn]lkxshvdqjairdnnpz\nmfspfyoqeyalvzx[zwdzwlsmnktynntn]eeogyyanaydeykwd\ngvwvweokjzagobku[ixdetnocslayahccde]juncfldivihwfpee[mcpxioooaydtjmojwm]satqvbxfkxhfdrgoin\nyncjgygznetzrrh[uzkbwhtbtkrcxcveik]gehtfqltpixmsuami[nqhxycgquaihujx]ndtusluyzjwufzdh[ppvannvzrnncxpcfbyy]kgitvwtucjasvtk\nfeushnbxghbeqsu[utnmthhouoazgbym]jmplltesvrbrllei\nijwbtaksbikedfm[gjckpcivddahwkp]kubvhiqvktkkijchj[qocdkdejflyyzwukfrh]qlnixtictiubnfhvv[ygbwjbjxtvfevjug]dclcjonutlwyqaxx\nvqtafpvexofwcfssx[zmlfsfqivipeumubau]moqspxvivckaesffn\nhphwnfopanasosexay[ddmqqktxkrurcry]slvhqigvbwonriydzb[ynanjunpszocqrjqm]fkdtvygiiddygcrg[jgumgpiumyhktlhoeom]dkvwoureblktplcjmi\nskxhzizzzfrfausiz[nakguftuobnmkoz]buzexokukfscgmmfru[jhpsafmtolwlhvkhs]hznyqntiienjmspy\nccxuwxzdxtfwbpie[shhongtetcwukjbre]nufocpasneteinfkk\napfhilvripbjswmig[tzmvefmwonqiqdyt]szdbbwkkgaqmjkhpuu\ngmqjznmtepctxpcfnx[eezqztmqxceenmds]avqugeuarwprizij[uumhklvgcrkfozd]goypuraafiwdcvq[zueuogjqbnsqmjfmxbn]ahgjvoxojaumver\npayebfjnonvscnr[nzubpmedfuvkiwqkycu]cvsjgdyfvzippxu[gmiawxppknjjmvm]spdngdktoclylmo\nruhhexcfvomrhibmoux[cjkryzqtfkckieyzuu]vkwptpezjrouirxq[sggqhkgstdzqikfnxk]zxfgbatfizeivfkjbl\nqqizwnfaajabeuskjdu[szujizggsbdhvihk]wxjmzdiqugjylejfu[dfygnnvhbvghhyuzo]yeaepigfgdcxbav[schlmqwlcifeqjhixs]ifaxsbjyirgfmwkaott\nerxreojjauvvlbsxomv[xaneipervgreexmp]itfaxjxrwueyrynk\nlgzbkiqfbgvdnyt[milmskrelgdjggvtmsv]clolytrsgczyppvrhkf\nryvrtxkdydhujxapwjw[ohgtjdaeifxzuhoqc]yflsxucxibqkcpft\nsrtfcyyruyxzxum[ygeoeyfnlufgsjxjm]ifwimooynxbrsxmyk\nrqbnowuwuernuxpim[zzumupyxvnbnngmc]uwurpinkjmkckxx\nikzheexqxrfttoy[uwegndkenfvosfpm]acomhjgdgbuelap\nsrookpxqmghokjoegi[lhpppxjenrjqiri]mjlixhnrirctrsupv\nonuiajxptpjwixyvp[otlnjwravarqmepwyd]hmnvzsflzeyrlxgpwwh\njmpskqdlbuorcpwpqj[sxwomhbdyomudfaisda]nvzxtvytsrqqxbsug\nlohoirsglnfzmslubqc[pxhygduybnlqemp]eulzazwozzqytmn[joeiaeuczyygjtg]tnowqyhlrtmumjyrkp[lidmrorxkpcajufzib]ixxyjcoocfdgzjbhhl\ntmixfdhagahaqeers[ruioctblczdbnusokt]orpjrznwojfxnheoqbj[gbgyexwumyintxi]tznnvbemvedlpriyu[ibseuzmfqmroeeawur]tkggtpbcgdthcpo\npsnbkiuzotsmeklinng[qhigmmuxrpjmhuhxt]urvnxarbhbsouap[chfgrdkbxmgqzdccv]lbopbgjsbykugbzfp\nqcneczsyljovqwlnjz[mntyylfgsuvpjdp]osrpdqguiouevrdq\nxvfraxzgsypwfmswwwu[oyrmndtdginkvlzdid]xgtwrddwmukzxypxl[mcjxgiimlmsnizirzt]gliezwdntsgoxznesl[vwypsvpvcaeyzivjo]zigujupypwjqljxaie\nxayweakpavlylgjl[hxjyhvqwnyixcesj]yuhyulfybuhvqiinlso[eyopyetglenvqzqhnqr]mqcovyockdqdqvfer\nsovuasutixukkuuxn[jlvxhosfgqjcxnlmxql]bekpnvhdbyhmmvdhplp[xohnfpbaeqpbfnfi]eobpufxrrjaajjd[snnfnhoikinfhioa]syhkocukumqrwcgw\nvhgyxqcvafubikvakos[jfivvuhbnehuqbeyu]dwezavodqhdmujzc[naepoqzmbtiraxhskf]bwuozbexnzmpukgu[zyzfttszjkatnovj]sgkrklrsnjzduvvjans\nyplxqjomjxguqxjjix[mvtzncrxfvzjofx]wlhvxxzsdcfptbse\nddqjeqgctjkvwge[cbgnejudebflhpm]ryzxhqqixwsoztz[hxszfpgrjuxxipt]zuvvwbmdvqbqihy[gjfkxykdstapfhu]bzprrjdyjlljxnxb\nxbnilldcerusgpejs[pvldiyrckxtgoesbti]ljqvtntbhxrryxcka[gdqkfyumjhgbzzwlvfi]uekphsrzawxriyei\negwrxuedgpcppavzt[mbblqsizmrxdwdrio]dzozhiodhtlvmrjcygh[gdzijmqhitlbhfw]ewvkussgmsnietkiv\noraksmkemjiapbdvqxc[vvgximcdecwxmpbjsr]breycrlgdwgnbjy[oqqtlhrvdyqesttwieg]dksvmqwavamfdma[fndgywlwmsmaivduv]mfweojoshjwolwla\npqpeytynxunxdfyxrmr[krtrvrufaemrmit]kcgnivmpvqoagjmharc[pvkuwynulvvuqkif]mvbbgwnmngtralbe\nnsacyqfpikkoqqxp[jdcdddcdcylpjiled]jstcntnjxszhichrkw[vzfusiwojvrjzhevjm]lywsheganczawtqb\nrtcpdankaboogxhbqj[vfamnogaxasxdiiizk]whpyanngpggqutan\nqlxjojmpesvehkggt[flysjbaoiorosmpzcl]wgpxurstlnopucd[ewkgadgmllrewtwse]icnqidtfsqjurnkw\noifarludgzqkwtdm[jvoeypeqpfivakqyj]dtcboyxnhejlitz\nnpkttburtggvbsfuiwo[wvklzpiffhreyxkz]uhuynxjezspazaudse\netaapuxqbavybsp[mndpkefjvjupccx]pdcnnncxtrzfvlnmq[ioehzamymeougocos]hcuxkuwhwvjvysbwdo\nfjrsuygcrtpzjsw[rhfrgfnkhajlqtqdp]hftckgnarcgoyfkmimd[hkldanmovhazpcpwhl]qomxfqqhkcuqhibrl[tpbrlhcndgbxuuzdng]knqmgdkpbljyufzazki\nzydstadkygzvjmxdhu[qtgaglwyzqncfbds]dqwbpmopxmdtkkcj[dcakbjdwzlglkpndtb]nijwetvoulkydqukzn\nhbxhybosbnopyxpnnz[juewibpcgkchnerk]pvdtzqclnvdbmwjk[wmtpskdcqiiythces]kbhxnzcnjxhnkuxwft[yetvomdrmxarjwsumqv]pgumogczlkgoiyn\nzaeaejxwpzbqtjiutt[eqjjobopoyuoxymtvb]glxzffwpiwoqcciyul\nrqrvuzjvcgaancl[pmxugkapydtxezz]lihcobqbdqenjmxyn[aemdyhmkusmchckzqnp]tgiijsdtqtqomptveju[mvaiexukertbkyinjc]pjuulfqsxhbpdiy\njjygzflwfyeiecuztx[yrziwmbdidxrjsouxen]bqkyguqcejsvrkn[hzipqxzodrnsozfmta]xvtakmgzpstbsivyt[ieiucrjmzeupsprslje]iquppghgxqhosvjzc\ndwprarljcykiecn[wvdjaraappnffzsih]difkjyzhcyzgzjl\nshsrycjlblbrcpv[drktygzuxbooshwhute]fanflcwacerdevozor[feybgvfyookhlsoivd]ixzfmefkgvcdnxqvy\nrgogoobzbggsbeynx[nlnbqvcwdyzkbaa]prjegdbkocptzducz[tjanhuiieffrdspjf]bhhziiqbzdlkdmj\nyslioeknctqgcwk[szhjocwzxxkbdoykvjj]aowmmepratdcjkgwjhe\nyrfhkqrnxzzyvrocav[rqyqhvtneezcivu]hunxsvslxgfzevsvvw[pyyclulboseqorxoihs]akjsixprdzbyqlbupi\ntcapvmyxklqgewra[pwxrpoxdptxemahbrot]ncwuxwfzukwcatres[ftlzvkapguezyhnsgl]ermejyvoisweiqvi[wynjqudtjghztati]vhpdjconbhhejafgfu\nqkqbjylknnexhcziot[lwjbulvorpdzrhddlm]mvvmstxnwigtstskoo\nwncbdjbvzjvrrunb[riirhteyuokxshfmxed]sdcpacarelkhxkt\nxxcromhxgxqeokih[xxcnkwhvsylkpfbsj]xipnqesaslmeqsnu[rmzahgumualwizqnf]mutxgygzbvgkimvab[jypnhvoztklxkxyzsr]qhuxxsuvigbloux\nyenrilcccypxerlso[dttyspegodnpefcpg]mdhfzxgyoxozmgi\njndnuwbhvaciqduyfg[xoeqacufaixieedbtnz]mpkkivmhxwxujcn\nmajifpotxhylyshir[mhcapgzvvwadphfid]rjaoxsvqlqyvqgtxte\nimhzefgngckhvgqcjr[zysfanhwbnqzysui]zgogpzkcgjeigcwpv[jtxumxvjpotihpmb]zuuueogbabahhwa\nijrqngygldyukndxhqw[xlcwaqfuzjigxddxjn]mcuyklxezeidilnl[atvcyujrcexfnknulm]txxgigzthrbbqna\ndvhqjqbgudpghndlvu[drhjjaxeomuoxxnagyp]dbeymfmzzevjydlzk[gklvfdcdfmnfvfslpfn]kssctqoyxognwiem[aojhwzwnegpnydzywor]eyrhiouwbqfpeoto\nxznkczuhsgldtilz[fhdcsnfixqbysff]ppbqiltpbrlhjliz\nzkfgueqzataygeavus[nymgcgakmtuwnkidr]ypuhovawsbnmlmpo\nlnjbdjnhhqeifmi[diompfqeocwmuqi]kdawxfqtkschlgnh[fsmxaerroipesmywqa]vqpxljxwpzudocn[sffzifosvfuytvdzb]fjqfwikuqzhzuthxzq\necyyeabjhjrfbdqy[xpqhxzehjkjhotrdlk]ztrkutdijjkmgzkuci[hwdxdsprkacxjrjjtxw]fbhbrjzwubhgjdwvpjy[vppgvmthaqkgzrzva]xuhyvaytyufxrkgeb\ntbeqtxhfqbbdrvwn[juqpksgrfsbsqdx]znceqzwqsfrhavmetys[khetxkkpwfmkmlvc]hazxybkgkzrmbtqshz[yavtnkwhxppnqwzwj]hgabdrxubvyvgniz\nrwvvgwyfgincgkurooy[wxcmmmkqpmtghmmltt]kgtqowxiyjbepqnkiyu[iofgybnjrqtngltajvq]mxsbhbkhddqnfowxw[ptqpbwojwfhhqyv]ymflkhgfnlagbxddzr\nlybbfxollocxnfxfeba[tvjolzzkenoxfxqrocd]vkgswdtqpilvbixss\nyurvqideiuqwekwop[gxsoytqhoasfouiasm]fyhiugkvhkbcfcshkzb\nrurapcltqwutrslalpe[wsqprvdmmtohamza]xmkzqeajamyurualky\nbuprncslromlgznqper[xjefyfgkufdkspph]wjncmqpgmnjzmjbqc[miovfouyxitayfs]gtrmwhvmgcliwegeg[owvnsvmazybubxfrp]cdjevcehzrminnc\nuxhqucibxiemlbtg[dyshtfhtlbjreji]ilgubuujgmytfxeqzrh[zahfdfyzbhexldxg]yohfxkodjqfdzqe\nkqcxiuftivavvdv[rbijqqjbhpdcrtpcy]dijrgcyuoqfzronrfps[knxiljzdtvauitad]hohafhoofjhhhppkr\nvbanudfbhmhpqsdpdgw[ksrnxrccuenustesws]bgiuwlkckvdplqygpi[ivyzkermofckkcotkj]mhjspcpkcwsbisbve[mlmgilflysuxqmzwp]afixxyabstclpunrya\nmnniaptautqeenvmog[wfqrhlcbcwqhwzj]ccouhkyhrvdcbilshrw\nzankwrrkgkejsfiwcox[gcxocohqugmgpfoea]cfpphqzxdllapiaxu[ckfcklaedfbhgino]pwdqreudlymfoif[nkaiutnpwnsfrbzqyuc]mscstkuwovgypqtta\ndhhvqxovlmkpzsg[loljkdtjkdhgawrpi]ggnnhvbpshpwoloac\nwjepglephkicsoti[lvcfarizbzsudio]httbqobbfjoomntye[rrlwtyngtpvffaanlpw]moqdodrnstpwmhjrw[ujoowvjwddvlqqbbzbt]alyeqayozgbhtpsni\nokuneqgdkcjggazki[ebqvcuzvuqlvptuoqf]wvcvzlzipmoamnvjt[dncwvnvagpitnxtjo]oadxpnnqonbrrarqn[ruogikvmdiporivvzm]vicubwgqcblvvop\niqwlvhjhfrfeayiclzb[mkafugqikswvpqehb]ezlojhjvdoyzwmggb[mncadipbeamkzbndk]kpewfgsurwlikle\newpiriwkjrgicwzfxck[iazlrpnsiynlmfi]srfoarhvphakmcyke\nfaalgogxxzuylnk[zsgporpeqifzknzz]mjkbrrvswlbgdwhmlgd[mxfiiekevaaosozya]klhonreqfikygbmf[hhgfoolpnquxfxoazy]vcxscuxdbvevulug\ncurbpzpilaczuowrsi[wmyxdecknwrspllfhpl]quuvzoiqziuotvfl\nkugdhavlhuperwafe[ecuvibachziwzefzn]oyhrdjgmqqauqhhg\nkcbawjisdirrwzv[fugffzgwmricsypdz]bouoevvlaykmgve[glivzpgoripmcnqv]bsmuvtuxrrzjaxko\noyaxoumybizeabdg[quusffkxbmxajbni]lxxqjhqcajdkqszr[cpgzcteolyloguchf]zxowxsyvudncstwk\nxmlnrjsanwjmizgawvk[wlyncljroxswzsmd]waxcvfcwftjxbqxpmvr[spiqjeqpfxanegjxf]sxzszkcgibvfkgtozy[nmhjzcaophbfpil]nrwfxurekvqndbzw\nxunbkhekkwyvgcerevv[bgjzbkihvzlnnpptr]huqryhbrkspzxusu[dmrytcqghtbbhhzu]lasujmpjaobcnfj[ebofoyovhhzsprycn]belltiuhimwgwqek\nocgmydyjloxpbsyj[wuhymkumnwwcdprxc]ncmkmnedztlutaw\nlyuydomeinqxrex[gukhcsjakylfwqodm]hdghwpfhnwjtmafqt[lqwtforyrybxbbh]fgyfkgvzyooifxa[kgxkzeuijywgdhuryra]dohlilkbkqzjsbx\nzgckhhqwhgctoun[ajftizwahkaxzich]wacumictegcbysyn[zzxxwgjdzicxreegal]pwquqtaijwqpkistf[vbombdxhjxwlboqdbqh]hfyfujedxzoceqewhgt\nrcpaadoewdfxoksbiuf[cmcgotvayrjllxgtm]pmkfrygwrzuobudsah[gonfdimjagiyayni]ctrukcwixqczltol\njrehwmakkkobozzwrn[beoievlwkmkusjzangv]djpjbtpjpdcjsmopzpw\nzsgrycgmryfdzqyfj[yipsuqvzrujoaqga]khjrvsadupzwwoasmp[bdpwsunstwzgzawlu]wxaqnorkgypawanoso[iknpjxzhmqermgl]zcsakkbrkkaimtnya\nuyuzptbpmmukyrpd[vmbrbmpgvxdxryzcpbb]ltybhrruutchwbuuicv\nddaeptwdykjibuffjh[ufzsfgmcffyxyyywdu]vrdexhgwtdlczpc\ncsivzntivihwomh[nprwknojctjnkov]uzridiquzokufgzgjs\ngcpleovxfcyyeme[crpzfylaxfpuecz]zoomnthfoptieor[ycybuegqfkhlupplwb]qjmvwbggqxwgeuneph\nvwqdvgzzotnnsydivip[ohjqzjuzxyncdbenf]suwfgrjkasvyhzbtfo[qfalzqxllbjohnzvgj]mtkkcwoapdjaysfyono[yqdgnieatutxldqyosk]debyxvqoatdeibyy\nlhljheobdtmdowhx[lrxkzhxzdjmemintrq]jecllyatwkrhfxru\nhowoydpdchixptjqapd[nuwrazvltwkshpvlg]havqlubvtfkhsmxwxew\nuwapzmqskzwiiqx[xtyqrsajsrljaajwedl]dgcalrxxdsfhqfdie[svghimwbcbmxqtqhjn]akqfoppjhaadsdbela\nslbymelmqscfinxle[ahjtgvzldgftnkehsr]vaqtlbhritaotaxvhpg[chcyoduevjsyehz]jncoccdngssgteldzq\nmmkzxzkatapuuwwv[odomzyzveadmmicfb]eiptpqypfvfroxu[bxfgwaezkjrbpim]hvfvtenhpyqiohxj\njetnikaiyuylckwz[vonvdfgbgfxrvjzluaj]zpmcyjvkwghaiuxic[irxghevzlcccxfcrf]xicbllnxpzlcmqbgm\nchvpdcrevaqnstnw[sofvzfabefeacnniokj]qdasdxrscvlmwcchq[kcpxsnydjsoviwwy]bkdprrvzdinwsfxkien\ncwoamgnaytsfeccbqb[vyysuocjjhfoixrtmpr]junwfwadfbyukyvnw[lcwtmcbwdkrqngvqi]vevlawxbwoqcibmtk\nseboazoqdqpckthgk[psehbzatcusxwqa]tiwgrqjikjzwabuufp\nouwlbqhczqgbljktjy[bubtiannyvmvkekhwbg]xvrlrmkjwkhzjjlia\nvatnmtxixznyvdvt[ftzepafpamiqpjulci]izhqwdhnqpyppuqiv[mjqocpfxdfcgpgmk]yirocnwnrzchhvrbfb\neehvjfqvnwplppeg[mntocrytmuzmuvc]zsfcohpjfqdrtfbbbh[bqhzekffwgpwsbxd]zlhxmhjluxrjmpwkyc[imisxjdmeqavdvztbd]tjlwasbwbrddpqpgwq\nygjdaucrxaqjcjj[zaunyucvccyhgomr]ifczoiwclbaryopmfa[ihkdhvovnvujtbasuip]mabqxvuzswimbitoy\nshzlhbrvjjzpyxfqgus[ykurcdmtryyccnysxi]sypivgjjgkngrxs[rkavyufibjkqetgld]foqdqcpatgctaehxi[jpnwjyafgkdytef]apehakogeatmfyalzr\nkithfcpkwdhgqjohr[vvpujusooxkdrmbcoo]tuzaiinsycjujjuw[fqdhhizbifrkpjxgyb]rddsmqvmitgdywh\ngngbozbqsfrigmuq[euutspovzyvfbgp]gobfhihxxwpndpaggx\ndctfsuzvpvttqpgppw[dnilcstcsxxkvwdsu]zqzgahpihqrhohqdtst[eoaatnenejvvuloknf]xwneniznbkjolnouj[gslnbvbmlwerbwvdti]jovdchklafrsncadr\nmdgpetsnkaddebh[gypkuqwwtjrzrhi]eyfbmxbyafuenmjdfvs\nnmkfscflwwiyxhzgzw[cixmvcvloqdyuikk]jprtrqwqtbrnksnxh[tngpiloomzgdmpryl]gwvmzbcftuthxvyqutu\nzkpdrykxtfvqneh[pxvjsvutuauoeducg]iduhzedqopyfgxjwpl[tmzqjdffcpzytkg]zvwkvgwmfhbqklyvai[scusvxtyjacnqtkany]xqsylxxrbgvudrdxd\ndbgodepvweaspcsam[vnqcsulaljbjrygsgv]gmfdwebiufbqkaofraq[unbumchixaeviclyqbn]ekpfqosiklnpdjrjq[nlcbhutxymbumqmwh]svtcirskdgbhfjr\nwpvcqnrvyjvfkfpclz[wogcckufvzviggf]oulptksetgaaholu[dwwcwhkktrhgkahbs]sobrvezzrrzvlihicw\nxlcqxbbegaulczmzw[xcllvvmlrdiamavgvh]fgipexbodvwutyt[pwhoyusimtkyswrc]mxtrsgpuxsjcqmb\neuzbhyalpjhxfawzyj[kqcqpulvktfqwccr]etzsqjqzeosiarij[kinbhoflquwkkobs]jvcmusgezydgutda\nlpxgexsvlfylfjva[wnzhqafvnbcbcoy]wevgfhsjrkdgvnbta[mvmabgghwicirugb]ctcyjxzknsnpxixkc\nhkkbtbsnyzrlsuyhwov[iurtqidtzfwtfhiltt]wokyylscmppxsdqtnns[swtohjqkqnmzxon]mthgkxltaceszxm\njernxnsovguhkpljxce[twgyaawrcpjpnxp]rvjtstsecwlieaeblp[tihicijqmcrggggrjo]igcnuyrhtaooygb[ntscsypsxaeatyj]aslpawlvpctyjzwxhw\nxoooyfocrwvsumzzywf[rdovvrfjqhtuiro]eudcowqfnmcvpkdpv[hdyyadaesuxiykkiztt]ykgxpvfilimofxfj[ittajdlxgptkzqt]djtaivnjndcktuvd\nusxiyxinxwkgmdmjlq[quaspjeawvvlagjmla]sucqobcfnryoftyttwk[knzzgsqjkwlybeebxrg]juprtecqapdfbkk\njsbpwwkgsmydnreqkd[abmspggfxrehkgk]nzhjbpwxrvuwrsnilmj[qqtarhezcecijunbk]fzskmnquqoivtsaxym\nmgekjguhkwyfdcse[ydcdycgmcbzvpkesg]yuzqagwvmncdcia\nwrqntmycrllbddv[fzewvpbxklyccfkqsed]czcxxkwfeberluvi[iupovtrukptjstnkex]sukvpgublggqzbecwz[rabiytcgypowllw]dfitoowyhfxjteip\nwlqzetmtxlrkydh[dbgzuittqekewyc]vsrigjcntogidwtft[hscoyacwvjejmwxxv]vpljhuinywgbjnynxhj\nydpusekwzovghcojdp[dqycroxflpnyqpnai]znbszhqqfkdbrwzrxr\nuzfunassiuljodnjr[tzrbcvrfieeocdcn]bmsircirorbtgydp[wcxinsnngyykaaavhk]xxqbherleuhjskfyu[wfklhczmivpuooytgz]fzxxivrumhumdcdt\nmshsdecfbmkjmbrx[fdhjzahrcoydrvqg]stkkbwrlhhnjzts\nnmbyxmysrbuejutpzn[ruyrvzgagqgybiqsn]atkbnawkdkildlbg[trjlpfbjomgxvvmzowo]gbmfxqgecnzrwowcm\nrtiylcxgfuqngjkyny[mgidqfnevlylaukbwts]vcejabirnbonrowlea[cancfhwbwdlklwo]ifsehqpalixvinbsr\nifyzslyhrydfxbsb[nigcfrqizdtzetpncxt]svvmxecfemwefpgduln\nrtzslwquokcygmdws[wvblnifrxmomsmdwtx]scpjyfputxvatko[mffinnpsxezowdl]bsmsjqeowsoobewko\nzllghkuucklrmwy[ylrocgxqrlkdkotl]gmmdzctugnusdsrwwhq[cllevhgqwlszrhlbv]prpeirpbwoapvocm[urvubddgwfmmkoyu]ygmtwdiwvuepkcw\nhnqlptboqzzpksz[axumkjmbmyxfokki]oyassusfzvnzhlobbme[vbnbcjaiiuqptfyct]oagongosnahrlok\nvgsfvfwepwufvvqbo[pmdxwkxldxhlqlqrgp]nmkpknxluiphfrfxm\nqypkqkfcicanneyvvr[hrsgqfwjegdzfmyt]hmsppdjbdxxtagyhfkg[ranuabbxvhlszpmlmv]ajsbmdayixczrhy\noykuwlbsupkaaaioxnb[cemxnilkmxflpnwp]vuvzxrfcfhqvmzlzl[hnvnqhipzparrqm]rjzhvguxrwhwyzc\nmdjjwbprbzhftjae[clpvjvsxatcbzsyybw]thsopmeuzvhcfppbha[hwbfzhbptymaaoywwiv]ybsfudfmveobwaqkul[argjxabjvcalkomgp]nogtearwoznoinj\nngsqrfixojvtgzmfx[dlttfdsvjeppwweu]ydwjjxycbpopceaj[anlhiebedcpahqihhd]gtsexwhwnpmpqvdxa[qflvviiybebmusv]epuouytlbtacnsnz\nouccxvpsqnmxezei[vmifqcpthebiklhid]tszxpvkgldobdjl\npauvqtezlhvjejl[sczynxdhjpivcogula]llemqpnanorgnkmjl[xxtooqiwqkcbvmp]anafyzhbzdtpcxcad\ngngdmikcpsuduzdrd[fchropeunoqkngns]rfdquwdpxtlfxscvhzj\notnuxdwoeqotcogo[jxyhojuczdysbfvp]upffjmvriabbalmlqmx\nxfjrywdooyrkvifzub[ygubulhifdmoytb]hjuvaxnchbmrptw[txcsgcehrbszmnzl]xlvcnwmeztfiyhlwtrj[twopxgslxaqihinrefq]tnbdtvwxxbichal\nbepzmphvahjuibuvg[zuoplvyeupxvzoprs]qgkpflfygaoxuriy[lgugebpiqnkxxqhz]kqhkfkyiqigodfq[hvaktogguzjumlga]gglqsklyzznufpg\ncnzflcqxgiepnsmpxt[hqbdhovnvyecljhzx]vawynjdylprjdky\npxhlvphiiyocalr[dfhohrjqchpblygac]oqdjtliamyneclgc[pzanjswflkxxwvnzm]qbbuqtxwodofarbbl[kiqrgquowfurmiqlqy]kppecttggvnsuzaarwo\ndkzdgkqnfjkadwk[bjzvvzwnbuhkinvc]xhiswkplvojtzwwvyph[qroekqfwzfqeqcfns]kyijvgidcjeeenhgea\nmqoqfigmgtagmxjt[qojoaaqyptscsfmd]zkpsvrsxzwvllxqpi\ncdlfgkthideaizn[klvwdqakbyaunqfxt]egotktupevsisej[olkmccwoqyqzsnuv]szxkfqjshuwyqewmgm\ncaanbkvopjahzmqch[wylutkdesribnllzbac]fjpryexeaxbopdjhhu\navulisxpjwlldll[tueldewuwemaihrw]vjzctwcvzpyiihnlrzo[cjdkrvxhmsglzllbpl]gcsruqwlokbdtgucp[nxubgtwzjtwhtdvbjuq]dpghqlnwugoywuiqefv\nrcfjxvabpkgxhlvzf[ftlsstmreroxhmuw]gcacbophluxzofii[vkkogukgydicpvdqbzv]dvalzsrgykitiqy\nsufacmzxrfdwlivdngo[kthzrniwspkdawxz]rudbmasvirscdpkpr[pcielclbxsbfedr]pneagajkflznxdrkejk\nqtvidydakxhrbrli[arccjldfmvtskqtot]uxldrdgmtilrhob[mfqcpjzuqeibckk]tjubrbrdjdakrdud\ncbwxzgidmrnjqukyl[uhenxvxtomizedkxwt]pcpeskttqdttvibym[egwkoivkdehfrlzz]pjueedjamrhpsnuulj[ccamvzizqyunxwbojum]qguxpdkjsvkuxiskx\necwvkjdmndzmmivxnsa[unghjtnrlreamcw]fhxvfvlthzqifvftbo\ntfzpfvojlegclkt[kdwzmhrpxckfknvmdqu]gnpywcujxlgishx[mhxacejyvmcleasixmm]ggmuguvhesyqaijlv[fcyzsosernhgawagft]rmdvdnkuaworthwsoi\nadztzinzrvazerolcl[vypxttybduwxgrd]mggcsuuzlwiilaav\nqnamzrfomzqqhozg[zaoqvddnqodpztm]pqhditszsmuiakyelb[sfknkiilewablfnt]mdzzoowquvhayznyl\novvwrhkbkeqeatbcke[wtzdbpzbnlkuhwqwfz]tupytpbukmuqytc[fpyravdsbihddaubymf]pjiotvegpewlpke\nlubqiczycurwvqozz[khnsmjxfeogtewtodhj]xhqksdbozycjszipd[zeptjnsjluccoiuxm]bhvktxgvqjkufxhprr\nzflhauqmcaiwnqn[jhyeagjfxbgnzkdr]hdwykmzypixrdykd[zkqqugefunjmuhf]ykufgfmmeaapnag\neqhnlafwpxhjtrif[ixkfnqexzmbmqencp]npxnxbzhuvwqnxn\nkokxqtbaemcjzlrioa[ujvykzotvzlrnfg]couurswwzchjzbxq[ympswhhwlvpohjg]wxcufycbxuvmrqekgq[wyljlkzgavafrvjuesw]dmgjejauotkmwgw\nmgxyddqzqmprxrdizf[clocszvenjingorxku]zsuqrmnlgyucrgboe[vpenwatmulopddv]expnuzinwtlihej\nxqhirwwuirdapgmyk[snyixpqruifdiqekwiv]zogryeticrubznbumf[yisxpgzptlkrmeevgqj]qrebxwojumgwfnf\ndjlypifibwpydcxrd[swxgzdsqfgksqwxjxfk]kbpzzqheozbjjcdpor\nuueutycrzzvuhvniu[nqhaoxpjrlvrtbahncz]tmxvdfxvmctcfzoqiux[gevrghyecnzmkrujmeg]rcyqojjmpxkpeulzl\nquyrwpchownternlfj[qijougzkibnhwzvjk]lmrfvudpzxhshukhpn[jvvvelpjnyxpwvo]ztuckjcxyxjvqop\nueyerkamylcyhgszgme[kpqbsxegdljldwjdxgp]afoamkxjljqzpmyef\nryrrppctsvwsxjslb[sbmyepjknxewewrqfsa]gevwiiwpwstdkruplv[ilkxpskdrntqvofj]srpukrzanrqhkprnu[jlujnhxksrytsdazgyt]fcxyuaotwykaosgnvp\nyhjojsuhfhujvfk[nhdemperlpgxpud]pdvcrmhvfeudrea\nmerahlzkjieamdkyky[yeygykydcucbambmtz]tbujyhneuvzacymtgrd\nsgvvjpfdcsriacwuyy[rqhuwizydqorikmqqlo]ozsalwkmuodygrh\njfzfzodtrqrrwvlr[ukxwobjdyhtqrqr]qzmrpkkjzqibwekne\nxbmixvpzovpzydwprwt[qnquthrvjmqtpzb]utnmpbzmurlbpfuaqu\nfkfzgaotoffusnte[ajzqatzkpajlsge]hamnzapphynrppmzwm[teysbhjrdgatijve]aigpcjplbknziprba\njfprgbpaubcukcmp[kddnrlcjywdjcud]nwzsudlamqhzrwlkh[fuavvscfxpynlxexr]szgousvpbqawlkpcd\nidlhdjsytmzcwcu[lgwbpjcyvpnecsqfhr]sjkxaancdmlpobiwjr[gzxmhvvugpuywst]oodlrjlodknfxde\nbplasvzaijndpfkr[wkvndyztlfkelwckt]kjkbnawptptvful[fmlqcligysmrzes]ujvljnzkznjvkgmsvqq[ezpnsnwrujkrbcmggsj]eghksoebyyfnptgqjul\nbjwqelavjebvqjroszz[jlfwuhjucugbvczdbil]xxuinqhddmsrpukke\ntgbvekwixowohur[hctpawxelfhbtmwc]axirbbtolsqjclqo[xcxiycbryxmpimq]kutifmilczlxebzxwjn\ndvxlbiymdfdrnnfp[nxrzuioymgfxqwxo]qhydikbrlhqldbq[heutjkmrstetknylg]grzklzcisupegmbg[mlvaswdotnzowpqw]inmxskvrovknbngkp\nrpoicdzdnkcxqtqule[gcxezbuirojvwliv]bmnlgvtpiyfhkukpj[gtqavwzdzdmqufnce]nwnlyciquxxcwpte\nubleorakkrqlakyr[kqwacjjutlifarh]dgijscrhnsrsxqhogb\nniodmrcgcjrihildfw[pmtshihgrssakbouvf]otoaadrggvnzmetmyds\njczcvqxamrdcpnjl[pitcvywsuryykynqxax]zmojzqezwxdnwrcuif\nnbmlxeosjvvtihmwt[acformsggoqxslahuma]nmezephkdzghfvhiqq[epizeyqkmseenueefiu]alkiffsdvovxmejkunk[hiwyudbbuondtsqjm]wjioowmqljplehwe\nhlcllqbyvenlzcfgz[tkddqsjxydctcrcuhq]lnqsaupwdmxeptzog\nrrkevyquvdogauq[lxscinoclyrawtkvr]mbiscfistpoutkc\nlwkkwxlifgwimrupndu[kglwcbuugjkujltz]rrgozebmyxigvxefa[hxbstqxfjnzvkco]rqpxaurnjtzymxkvtiv[fgbvzthgqifdqehisw]kwvdvfijmbimizl\nyejkpafozbchconq[chghchxxcybtarwkel]ensiprnejdyegqiiu\ngsclugkgowknjfkewxn[pgzgezavhgcfjpi]wttjlezzjwqyyzgzc\nndgluxoxlnekaomi[hrrjyflrxyetpub]kwpcbjgszdjimqfgat[ofdwoxrgxjrbxhgep]rdaebrkfchddavjeqap\nvzlsrismjdiyfqzcieb[fylncgldcdlrqnbpw]hyrajwsfckxlkhcboe[rxqyolmmgairjktnk]xhrusylermeiiolade[ifiekphfwfzsnrb]szyunhntoeymkuhyvru\nekgeyjojapzhzaxfzhw[nmmzpmouaheahibz]skhvrmqbvgkbismmmw[lpohwytpsrtegazzkwg]cvyqhgsyodcdoyandpp[rntevuwuoyqnhkmrr]szsrcjzpstfyvlf\nioykyddusobfdscqkmy[pmuczfvmkjokvnoxrz]osyjyicdpcwzxvwfn[gimnsriontvxypcxnja]rgedrrsbgienkkwy\noktebiadpwprzrv[wgprjpksbgdyqidklkf]xhhjmhfbhpszdqu[rxjenkcvcswchak]fxqrycgufsqtbxx[pyxvqyqnctpzpggzrq]mmncxhloifiifjpnitw\nxbqdzlpfxcznmczfqq[tpfsrcmbflynynshgt]whfhtgfqobzaolpx\nhfbetzccpyqauunfsq[ihzoakqpjosfmeff]xvgsqfzcgxtranek[zbtxsvwatcplcseik]vaidkyuhjnsgptupyxq[vprljemlqmphnaau]vfgliasxcpdyayvfddk\njetotpxiincpkjxqmz[sfwjrlxbmpafwtjuy]rasahmylsaswogm\nipseqmdzbeeqjsnvo[qxgatjiqzhwulhgkjm]syofcufklnbeobppx[lbmkistwoiolecjh]qpznlrllrkhxrnyvf[zbhzvyjqzywdpvh]thlrfwmziexkhxgp\nuqyiqoznpgsjaaftzq[bfmkexvilwsavbrnwo]pwdssrfyvkefanxnlfr\nyijgsezauqoevphn[qboayuokxuaztxd]peepgblucrlstsln[rnifdfjhxdmtfse]qvymgyfdvcpezxdgmen[qyorafkexhajsha]knaylffgeufjxogyel\nqlydmvzjoavamnvot[napvavoknajlvmdd]wbjkbdpjhuhxybgywu[umxthkfbtbevasmekcr]adnybcirbnsyplp\nqshfqvkxfhgsysl[tzlddkjozqzcpcnx]xjkhcdozufunylwdzs[smgwthhegrzgufktc]myfufzjuvrafwalrnn[jhsmzagnqmhzscu]dbqonhtmhhdshdyatcn\ntcdybubnklvamrjlxqo[naocexrxejgekonegma]hlejmizxmhxahxboitw[jteivhxwxftlyhl]kvhbakqlmukgslgvgx[aueqotadcogcmhqeeec]igrfisukejhgfmdvx\njowozfzspexprygzplp[acahqiqszrcdhsylwwa]ppdmkmcrzpzbflgeld[etwowmhcqhkjkkipk]gnilcosjuukihcwyne\nynmgkfpaiocmkybwkz[ztxveuhtztuioruvqbr]grhetxxldtoepqtm[yrucewbvzbphefuf]idcnnpztztemlywblpm[ltaesuehnzfrsflac]bbarkjzutumhskhf\nmckdhqphoehsqgjzpzi[eiretkkiklgmfvohgvs]fsaipzocdnrwworpfj\nhmdbweapvrpdkhqhr[xwpfkaaejitfikqgy]atylpiafldvqsunu[dwvoqhxryfpiegidm]dyvhcjqkgspgnpw[nkabxwemccqznbpdq]ripivpqpjrebswqspd\nxdjfwlhvdtcxqvfzrlh[kcjkplfasydesgzkkh]ilfrxwwjtpmshhcy[gsobusiljqgosoih]dgtehabeomwepoaaahd[gikvtnebxclexmsc]nkcvdazorstiymosjv\nfjjpjjjikuarjinig[ytnbvaleddhkesaoaut]eorhszwghtnmzbjipie[fuwkcamkegyilppagl]pipdvxwvkvvvanblh[ipiaupaojxfjukjgk]purmzuzammwgfyle\nqclqkkcoimixsiou[psabxyezhvejtdodz]ejzppqfiokslbdzoyo\nhrrdaecpdytoxkwdynw[vhgsgzqlqemkdkewg]yeqaoolmodchmigyxt[whflgmjarkpzbitpkl]jqjtyhnxkklkzoa\njxdsjmkuplrowpkta[uzwnxgrrcieqvoz]vtwwzqgvdeornoqxmuw\nigfbnfbrrkfiyngqux[aajdqilzidsasrthcnc]xmkzmvqsexhkttcd\nbmcwxzeodkxlxclq[zvmqvljaabeakiei]xzujkuxdmumimotsaps[xuhocncyjxiyavon]hslcfclmfhfxxwwrln[dfmghezypyqxtwo]wxaxiadxkpvuwdl\nxifaalrmhugjejbl[ioovxgzfgpaqlyt]uayfrtjeutfeprmb[fknrvsrbeucxlyzauy]geowvgcfjnbglmrxp[ocnpvwnagqhgbcvoupp]inzfrbwlliwgcsqgzb\nwccriqkjssvswvpgx[apoeqvsvtniwgbt]wfrmnudgajwhkcy\nmbyargqesqkprhbtaqq[tpxvefsyzwxvshmict]dxpxmxcluamxmfq\njfxpcnpdgytwhkfb[kdrqmtogtlmxqmv]auuyjbertdteoho[tdendgogvoevpnevzdx]eicpvtgotdkcgwbd[ygcvethlzayahhialf]kytibwtgzhuvvsjw\nwfdfxjuqfxjbnjpt[mmaupydmuixzfwebpjt]kssauqawybxkfmcu[juevujxyjrwzewzua]eladywlrkxglizgc\nqtkmarqccnxwoqr[vzmovjwxsbhtnmjhqjh]zycttmgyujdefxxfs[tsmxkcuqircrdwtsz]uhqtftqwcxreyvlvff[kwsyvatwweenxdvqum]sjmbfsnprqixqzx\nrantzkbrnpwuuvqbqn[qaudnwijvntnxlj]tfdbqbdepavxiewo\nxwjmsobvbyejpyjkrz[ozkgsxhxiyuejjr]etkvofiicvcusmmlg[rmkhfcaxfbdltnpwk]swklpvfmxmlfhls[iexmcqatbamzyvxft]djvoysjwetzhocdd\niixngfiuncqysuzf[ehzeqdsqwwjrubb]udkdvfkdtxbddruub[hktknkxemrlnbxwz]qfejqmapclbzhhe\npmviizplesuakfc[woqzewypfpcaiotx]xatiburufdzajqrv[ydsakwhemrgnxgqyli]isubtdzpkcgsoas\nxxsqvodorzrnrbzsvyu[apejbcvdjuyujpxewu]kfrcogbvnrkuykpgx\nnkvsmhvlyyweggw[yhcjceblmlzpgig]smpwtbqsnklgxxbssz[aiivebyzjnbelkphux]wnaojsgmpoiaykznpj\nxcllttmboowsgodsf[dfskztizatqovmat]gpzyyqjotpdkdemcjon\ndrhgljhvyonmqzkr[ohxhjhvlrpodxwy]mrrhedvtgdxjhjv[golpxgauowhwdoov]rdmuwnfurqwssgth[atspndhxuuhzadog]qgdswxcwwahqnpx\nuvdajunzymasgjc[onqeemcifirbxli]mrmpwnqojidvwexxrjg[vbpwisdwqtiteawvdw]rpjzhfsfhrzukstel\nowbdsotbsjvrwvdb[fclwyuadozjjeyvkz]uzfygewxtlgjhmfpyfy[qlnlpqspocvcpqsa]fannkpftifaoeszzu[pvwpbdancbljmucxql]tlzusxlphovfyfflj\nmmtmuzzulxmgxsmf[djwlpuwrkdpcbvv]jomhrdgighcolvayu[vdxrekbfbxgdluj]mwkcqhjhlrehesmwft[pigmugayjtdhtpweyo]lemzwycbgzzhvin\neferdgkfaasmkyi[nopnmqjuuhhkaclf]twwodgunizovyvydh\nbaddrprmgewtmypxsp[yahwshbkzattrry]tjjmawkirxcxcpkbdr[kcptwlmozcgjszalueb]msxrkbrbcfnflgnqe[amwmeanfnbrpznz]jkkxzruebylcrqkvyvk\nkjagsescwfjkqrykx[sefltugsdwkybwj]jmebeveaticpwddxbk[ktfnvedmpvqufsi]zxjysrfpzfhngjci[yifiorzwyumqotxoch]afedqtkmzpfwnacb\nlelwtilhzhzslvzo[ehvnqsjxemjrcvbqyf]ovygwyyazlsulyzhjja\ngluywzrxutecuauqi[vyllygndlfkbmgaoefq]cyucodjkxwauafwfxw\ndflaghirjcyhylbcenw[dndkrtbxackpdcphny]pnhqmjxdzkjycmdo[fryelfouoaesejoq]tdhcacxuqwfspqevq\nyjnumjjyewzjnakmnhv[ulycnyiyvszhifgscjr]xheytyiiyilswfhqywd[jxrndqsxmwcrpwrfu]jquhfnyxudasmomnpx\nrspuvdkdzbrbajkj[dcfpcvzpbodrxtl]xbskonezgtixwjfsuq[gubkcjizpgfwqktcc]ddjzlszkolvwqsrnnc\nmoobncjrmmfonnmp[lpbevkcuzvqguwzbzb]pacppeefawsktrydyqd[wayxdzsvisprqutg]dfysmjhwsvnavpixfl[aphusnjjnvygqikzbz]qmvbpeopziujlsmgx\nwfujisugotfsymh[juvkyhewsnpzualwau]ljyuwiidwytmvinw[qicxeddblcxrsdrp]khdooklzguadokmdbd\nwdzzexnylrbsniulyv[nbehnwkwkrrkbwirh]ymyaqhrhmbuolmtbz\nhsxsderrtdvolsms[yqxhutbtoodvausgm]eufwcczbwgvzxsti[gqewnssdahkfambauv]hrnsadgqtzcegnplnce[fwzpwvfptgbgaahdn]hlvjzdqpvjezifpbh\ngtnyrilnfgmslzfju[qwahfyniqetvzpb]txlwtncptwapogp\nxblzbbrwjoudimv[grtjaoaytdyffbl]jojuhhvrrgbymoptzi[rgpexwvtgbswbzp]ysyfhclvndltbnnzg\nggtkfikxhhzevnhpkoj[egndynfnwwogwdttwg]gmdytpspodusstki[zokrsgoycmxdzrni]jjtmaoztqkdpsnty[ishkqeyrmckkbcug]jkkfuvenjvphkmbtk\naprzrupkmqzdgncwuq[ototomaxhriosvx]zftevshbmxrjingy[vkrildlncmbvbfi]wsqygjuriitkbszg[ncmxdegpxcdvtgau]iauwjlqoidqpkzkeazx\nklbfjwxkpqniguvq[wymwprcxjujljrexcg]mtjifypvknsiogypja[tfbqvlowzqxqefia]azvpxtyghflrgdo\nxfiwnyfpxzaizzzhp[jsfakgounppfocql]gcgjvygypcgzvnu[qmwugdkvhxjknumcr]ftgvxsqochhihwnsb[acnafcpwduptldm]zcstejwdgasnvehwyot\nrepltebkzsojvhxy[chzhbjyllumckfluof]lhdibxgatvxzzhzflz\nilqmrorgodzrbfesczh[udnwlveyxsalbxf]pptfzbjvkxksoarpy[wffmfpwwxmuxfmrvmg]zatihmtjlhvjbzdwr\ngjqtwvpdnhhqqqvop[hafmfvvzhqrnugo]xgrpicypdmzyjodfv[vtykgzaxumptsclyf]medyaqnemgrawbizrdz[ykkktuzmryicpimqgdk]wyxwdmdtrxcpdqhsrli\nhjnariohxtbsthvcwj[jqplvjyvfwbbphien]yyogxtzdtzodxceve\ntqajsqqmgynvntqf[wkovdsdotmgxjmmgmoz]kyffakcqgknonqj[hvuefibelljpsvaa]santzrmyhmmfgsac[xevdggsuztwdjllvmod]osdymicaxgknwafiyhf\nxgangxswvkcjsek[jrvhyhmomvqblucr]mhakwjcqomofhbdt\nvuuruhdlaefeyjtemtn[rkewcsrolbjkvgnjur]ajuzfefffkgdtzfmfwu[ysqkcwziamybbcghjb]vnyxgeftjtrxeokaqk\nytfkhfnkxsuuddh[uorumsswhfhyjhnoqe]mlmhytefajriiwzln[ivgrtejpggcetxry]gtwlsddrscrxepv\nzhsugwnutzaxunnfbj[oenidjfrxbnbnevjwo]wnscklrurlxquzhuwf[fswcwqtoexgrdguawj]knactvqybzyjdjdkdkd[hwncacnowaliolgzmlh]xcqfyvhkoaxjyrxggg\nvfcdutbbpmmhmpty[glvdyxliujvbdqr]jyavmvfrqjztetyn[rqngwyfxdxofvqwo]xqcpmtqhrkoctux\nzfeyzggpwatzvvr[mwnxvrajqdtijeqm]kyprmauvxauaeuntay[ivwbqplblehbbhi]xfasnjwliydlrcyk[jmalyrxoozbrang]lksylhfvgbezkcf\ntrqdnrlvoqyqyvjt[ekkkwqklawagqqprz]zaojypuwvzdghwkye\nbmnmbsogxhtpved[zffxeokudzgkusvk]qcuxjdhqclszjnxdhd[rsjdhjczxtrghlxwh]vpekhuzoamazdzgufb[bgtmhavdkyhtwlwcqmk]qucpatddwrtjztpxvi\nhwqfyynrncmhcsmrlp[vlaqdzxwrpawflemknd]kmvyzqfvlouluxelul\ngnzpgjfxtsaiknapn[rganasfzfnrvxir]ooatokkxjxhzxlpmb\nmpedacmqtzqmwqyfz[dcofwyebgsvctomzomk]vpqmhpoitpubjorx[thmfofpuparhszqe]clvrtngjajielkxre[mfcjhfugpyymytri]moqcfkrpazshwvh\nfxskejrgulaixah[cwshxkapatrgudllubb]vgykjzaukwxoyeucosg\nmgfyakavdeymyzxwa[dsvhoxfiuxixxva]jsxfqsnjgroxbmpiilm[kxkakjvwgwflxnnu]denqicbsmzvgtcxm\nzfqnynrdbdtqblxnww[nzbnvcjtsxrdmasqtn]yoganlahispbjdyxqx[tuqafqcjrxnybeksh]imhkfmqdjiyfoqp[oennqnvdpveoija]vljstbhqatpwvkbg\nlpzjqfcipceweps[indnzphetquilkxnds]oxyivnjttcuectlyfy\ntfhhmfeomcdyuql[ioclczzniueodbtpbrp]wuiujzhxjbgdlqbm[iciypydykxiyqies]ptvkrvkragnibssly\nybllxqqxzjlhskqi[ytsvahdhxgwnwql]pzfzcnbxiypkpytv\ncchwtoevekjgyqqs[kizgrwqwbhebxlscmj]tjbuacerkadppftxdpn\nnofeoaawaeoepwekxty[mgapdpmakihrfzlfvpf]huhzkicazfkvjhgdvsp[eqtuybajdgdthtz]opgdgjzkrfejgawxn[umbakkosxdtfwcfh]dhukvukdwsevvcmt\nnhzmrmtfyhjpvbsi[jghcdhdrxermnhnrg]sasarolrztffxrvh[tafrflhiydopcqrx]hbrwebrzutugjnj[ejqrvlcpqxtiuqho]xjgvbnuvoxjdcpx\ndkizkqalwbetbepak[detgokxgkgyhrqzzbqq]rmwrqwolneotsyvq[fpffqdefoxfczyfb]dxwsppdngvyskdpfnbc\nygwbidlvlgwncfy[ouryypomwfwmnka]axlhgqfgvrfsmbs[zavmkhmkjzvpzlxpkag]bfewyvdthrjzmmjs\njwyxcjasntveqmblff[mudhpflnaxhhrphuwy]yyvtbzbohccozqj\nckfocickdlijiur[fejgtsphnigervnza]owlznrkbwqhkskgebbx[alnbdcgnktmjlnhig]dpfomgwzkqrpmicih[vovjambzftywljbxrgj]ihljubxxgrxrqpn\npygdmdnnbvnjlkacjfz[xwefajgruywjhysd]soepimqfbbhekifv[frdrobvsbwwkcytfv]aszgyodinewnrfdhh[wztqipflzlrwmpxefga]bxviyixobyldmkln\nqujnmepaefnkxgrrg[yxdnlyihixwasibuy]qtmnryswxwzkuqw[ozuwcixlzlbiacytv]oylpudpmjaqgwfqvsb[wljtqzfawkmrnkgkvla]kgdvfppcbpyazklfdk\nijkbhnjcxgsslwtkuca[pxpiyixylcuudtwbt]ooerzoxehuqynhzmhwn[ynmgxzstfawvqihdhoa]bdrhyquybjddpuroto[fhnnpsgnxlnoiiqcml]oaibnvvqupilprgcyiw\ndfqizqapoxvqvqixvm[mgrrcrzvjkncxlmq]xqcxnymsyxbtfebdgy[hfdfaxiuiexfdhy]flyhvoppwzigjxlytu\nqlakotkuqswwtqx[xnpcrmswyqolvyp]limmsdyvzescvvt[rrpvvituflyuhyhz]amdxfzneiggintiyzuv[cykruetmmqucsbwjrh]ymobjslroztxtla\naiufklgicgwxdlaefc[ofaqlmhnwrwhjlleyt]dixgrgkhhbyopqkzmt[zhqupdyazgumcagdids]mxijcialempjslotrgr[lmwxkdqqijndgoiv]upioecwmfnndajajbxw\noiwkroaymbjtugfvip[hyqrpfdrfjppatm]azycyfsttguvudeq[czujqevgflhvskaguy]llsuolaevinsabqpy[sivsqswxfxlanvod]sswhiwoaxhqsjnynidh\nqipfjqqbxflvnxgv[cnxuwbvnxndkoxcxjl]atoznchumwauytpqmgk\ndoncjsebymuefbxj[itsfdedfjxzxgvj]wpxzcoaybnzzzxz[hfxwmqbaiyiajiorh]einnvliwbxhjzxx[rkeenlrteubkvgrpmms]qbrpoghwjttgawgstt\ntyiexegppbtbxzovpb[yljnqybbavpwbwmvg]unbjhlrkpjrqbxrtpof[bvbfvhvgtawgpydlnn]phdnwsbwbljkqchww[galszmgwroduckhyyqa]wgfbqlipsvntmnspge\ngmnkhnuwwojgyybh[ivxthnkhjaevliiberd]crpicsxuksahuebnk[vogumtrrqupdjhtvmi]pcezvomttzmdgtelfq\nkwvkuklbkgbxoyqo[cckuhlseweoukudp]kuvdtzbjeoormufjn\newqcguiyodbjoxu[qgqtmjabzxbzjua]twmhfdmuudjrqjpge[xexjbzjvrungbvvmry]yuazblohcojrddhfzg\nirustuljdmhlqrettvb[dgsukspodhlhcqabx]auntsiybdcfgxjmsiqy[oqscrcekuibymdwfcy]dmxibunjfmqjoeajyi\nppvngsfdficcpbmbze[gcazeiyfowcmezww]wmphalytgunmpjqatau[qnhrljcdkikordx]yqrsgeczwcwjbqfhfw\niniqgrqelaihnllono[cydssebiyefnljxfdh]ljpqnievldmltrpp\njzjmjfifakcsixsg[zmgaofcvdvtziindqe]mzodtodhvkiluhuzf[gqjguyslrtqvcesa]gwzpfqfyfxnncsemb\ngdnmdicwnjwgpjqdw[odoslhoqgocoumxf]vodkzgngmshtzwjpgbn[rrhzqlqeixvxjbaldp]xsvbscotkujitex\nnnewsdtgggcgiawo[kmuweskiapswdskgosj]avjieesxujtqfwpuis[tvulfkzyslzakco]sjhbzevzvglgfreyc[wzxjjpsqmctkyoutau]isajcfzslakogyuevtj\nbrresmfifuolfyc[hkeljqzezcsvzrcue]zswubkhczxziqxlty\nxzohgybxqdxdwxfbx[dqcorjuppxguxgps]gltuxzxhdjujuro\nhmyrpjbmwmyzijkbljp[ipbngzbreqoqcisbi]ctdmsssqkgrjxozcx[egmuzsmsaiodyyt]ugjpwtglzvshohbj\nsnumfuurpriffdvj[ojmagqzaktihjmwriyv]rgnyhbobphsfqgh[azucllkylyxgrlom]vhtysupgjwbwndwrgfq\npxjdxiuhqmvwufld[ktpvbdokrtdpxrekaf]mamfsijuemlsyio\nolcpnpmilbzxxvqsz[ervozeicgvqskuenz]gcxvfthottngwww\nhphpdxpbsbmzshrwmwt[sapciwpwuradyvko]dnrhabfjqorseajgr[abhgtcdijsqfndmney]mmsvtcxmoobkkaeevz\nrtvrohugqesutzky[sjsvmjhonskkqwhis]pqjtzpfnvwsigtme[ckthdaxpibfximcq]peoffhphnstzruuhze\ncazrddymetaqdtlwn[tqrvhfevxilaptinubr]opnhppmmbfscporp\nctclntnozqwmiqz[qniikhszzxbcatctip]wpoexzkaxyealqhcg\nsuxvexjrakvhziolw[pxjlsfocisjmwzl]smoqdqjoczuyiac[ojpwtuddbldiaruiamd]upfrpxzwnthfytv[xvfejrchuditjal]bxzvjvhoigqunomnikp\nvjuryymolbathzinp[xrcvcqvbklvqtjnpzh]wugebbnbnzzvdmpg[kzdlfbpqgvbiyqwitga]wztqfradlqinyzfzf[abgygmhhsksnvso]kntwamrohagtdrsm\nernvshbquyjfymdthx[jjshkcpnxftyopjayzm]yidkdkommeyieirf[zxxkwqqlsgxpcdwlgq]zpjrhkyjkdkxoufwlx\npnevxgcsnqcdezwf[mnftbwqkrfmwcgp]rkmeslzoffovqheq[vxdcnglifignqqx]xiofsoyrslgyfrxl\nbjehvbcqagyczepreos[swecagoxtwhtmzsjxt]ihbrujlisjdftzpfll\nbdczzogwjpcdwyq[jptlwjoskogbhfcdu]sbfatvcosbvikmvm[njvcfwokqbtynugffu]qwhsgaqfunpacmimzhp[mulicnvulazcycscjye]oycycatwylztksmrfh\nidpyubomejrcwurt[idytppqynyqvdajevmk]mykbzkihnmfcnfg[ghfxtsrfkqppejwgen]rsalcongusjamgcltti\ngutkiuskjqzvbau[vqhivilwddgfrckjc]gpkuhglnqnlzndpl[tywjgkqskbdlsvf]bkwvgkdcxvdlvplmza[yeqeuyzuoqbypnwg]wsqmblkggadabss\nzgirdbsohsmusxbiqm[xnuiyfzmegcwzuvery]mzjixtxtbdruckher[ylfmvkslkcukfdp]vdwcmqmrsnedjnvsomy[cmmaoebsohfrnqu]bzgstdhoneuzfdxl\nwimnreygvgbpvafqrn[froxfavuvgvwirr]avnmgyvkwfnwfgudiks\nedgbqmwalgtiurhmmg[vjzrrmbtvyyhwliye]mpykphdsaunzjkpam[qdcecrxescwvlxmpi]gkfipuqdcpcqodcptya[pmdbisdhifodialab]wjucsoipfxzkkzwm\nxmurhwryxntmdwwv[bveccegjmwnppgio]rbnnbsqzutgyoign\nkoftdywagyijtsi[amffypsbtekqlbvlli]avskrcxhiysqqgjja[ixrtkpjnrhljddqzt]ekluhurkjnhlzaudnrj\nvqbrbgtnvazwyixug[yrmuvykapxyyqxus]ehhkvomrgnlsofbd[mgwdwrvjwhhuynogqv]nyjsgnomdxwabameuss\nupixiwerfsjxjvecmo[lhlmklygfmbxljvptf]qnlxnzoekmyoggtsmtm[wqvqbaemhanfxldq]msobqxpmwqyauii[khuvobspvluvghjhcjm]ysvqvfsfyanmyrbuxnw\nxeawztjrtohpimzkw[umvqxdfhsyyxsimzj]kyhlrkyxcnyupqmp\nhqzlqinkcowqqzp[vhdaljgjjfqhlrjj]gmsyhpvpblkaxiox[vhbjqxseofvbvzbshv]ecirxnvxadesrbvn\npuqpygmwhwskicogo[lbkrenbngbzoljzuoo]tndvmvztkssolnom\ndbswyuxfrnypetkm[lyuajkvfqzwpuon]oorgrpkhwwgtpzxc[guszbthjnajqffsofme]vcqjstfdtrxcuscz\nclhtmgyxqbrzeipksw[mwuhcxpahefneke]bssxlwoelrrgsqcicz[yyrkfjczqdsglltdjz]xscwwnkcwstkpxto\najsijhedwsivzvngsr[eqorzqparxhrbesw]lyvxgqgqguifrpuj\nsqtxgdsfkbhljmt[ndqljydrgqwwqjayc]lttwcrsejwxgxkuawgm[nefpbdmgtizfijyt]dcxacpeeyuzkemb[otnbznolvwiervj]hdcjffxyhtqdjmaipj\nkvohguactjmqrluci[tefqrqmjpzpsazfoe]ptxqfezuvtxphvy\nwmawphvozqxqtmq[qqtumumswsrpsnjug]wejsdbswswrjitmq\npdzwixvmkxpsxygxmp[zfxeglxxoxtkkmshin]hxjmzexyabkviollfnk[nfitohyddbdfqekaty]poexvcemyssklhllw\nwyyiqymjavixnwcnxu[xnhhsqavbnggdqn]gymwgjatpsojwfj\niqdkuwpqylmwhfvm[bjgqryooacvjmxtrq]dqhwmcafwgedohws[ucnjhrhnvekrgjefzxq]opvzmoismjdmsezvle\nommglribbfvicgmugx[msedauwycskyoios]qrhxlnihnwmktihzp\nlaphdvdlixghsmjpsq[blbjmefxvnjnxmmc]hnzsqzhaenlzcvoq[ppyribixnyeucvjlv]fdogfvnymyznuuxa[pelyyutyolblxzp]fqgcltvxupdobson\napnimgsoqfmqlgmjsvm[rdpnruzylevyuir]wwfenkdjpmqnvyf\nltskflhfhupifhf[gwtcqaatnfjdgywo]kvguorbhzxfqrhxnij\nkqaeviepbnrokflimj[zqzevrvhforlozy]orzvxhevxtzorkch\nuhsjyhwppwarmrfed[nsfzcvrwjhfuwjta]nlthyhmaeghygqdaxdj[esqbskelpkfswkvwmr]stzggiejdzkhohumob[snlnvsgiktqewvpxhm]ahojfbcfgxqmmml\nidlikoogcxqffrufcqi[vcuenzmwggmbsknfj]peoviabqngzwiqtvri\nrigldzvrvmsmyakcjb[wwsutfoucqlgorxnu]bcuixkbifegcmltqibo[szoqsqlnduhgvhlza]pcvurfgchanmngh[glpfevaugptbhqqrd]vpndxitsihovocvong\njwfhrlvcglbtbdlix[vmhtfcvzlshpfcii]gosuawoykketkzdhw\nbexfthnhhppzzutg[ewpudndaewfnwaht]wlnqstzsulregcwgmzw[atroqzyofendnnp]idtypgwyeatycgpde\nldhjuqeykeelckq[qrrabgedfafkzize]tfjpjpzsafansvygor[jpuzbjptblhydidkek]bbkncsznubtpoiahot\nmqqxpkguxlmvyyk[vnxxtwxblmjdxjkhecj]shwgynlewfeegfwo[dgybavttexfiaod]ruobjihpitxxfwx[frpidegurggjllhq]kcfnatekrezeqoqnpqn\npfelcxohsnhpzjnrp[bmnzwycytvwquengc]weaysvdqdkhrprcpmw\nllmwiwxeyezezpt[densmtrbqpiuwryg]pbgadfldspoahjimq[ugideashgoighvpiwid]pdvxaqoufmuvtrgs\nynviititdvccfewheh[phaubuotpzjwqfcrm]spytehersqqwhac\nktjvhepsakhdtvgoq[bnejcglklonqxmygyn]kbywvhkayojcufnwr[ipiujgjwknxzefdphq]zcmnmxqhuhjwqiue[dueiqqteiuvgyggtc]rbsyqjqegupwxbazttv\npgnoazapsklgvmejjr[hjzazneywdxkaki]gfwcgiyhuaovsye\nqorimqvzoheryivfi[usbcrrdgseveupnqadf]bvedishdaepjjnrgftc\nthxrgxhchpeczth[eneefpesxkgwuxpnyb]efgidnpfdesgcmkqllx[jglvknahzvxyegxxedi]cupoduyjkdpyajhirg\nltabaysmmffenou[fiqduygbghbczdsjcs]drfpocohdrhunajvmu\nrklvlmyqqxbttuhuzos[bihsvfaluvhdwqwcz]gbrlkbxpivsdykcjx[qoudfwhqcnbrmru]npquvyoxliacxpr[txyzvzsszqedximgecr]srcqshisakuwljrulf\noiiruuqsdsjguri[qfzwehlhoinyhjv]jwayjxoutcbbsxquluz[kbgrvqmxzsukught]bgspboampsgsivvuwe[swvxxnjbmcpffrayd]txmyfolzjpxdvqzdtq\nresryrrtzhhnpbdrw[hnirhiummudhyylnky]gmwqolwapineiokcl[iqptxfvtgabqyxex]npeatmzdsfknpajsub\naqjfwyrtqtrhnxdmfq[xacmscejzrlppqhlziu]bxvptkrvkahygexqsub[vrzjqbhlpywxzenkod]lqvsohrjrymprniyn\nobdgtytdzpcbnelm[scsrytqyknxdmzugidh]fpbpxshhnyxedvvna[fgebgketwucucajqip]cdmbxelnfsomsguvxdu\nyuluzhzwsfvngixjn[gjmdiyftbqimhxiv]gxjmpelluljxmuhz\nicsqqjcnwckhskoc[rhanawaofgbzenhxtfl]vsvuwijhjnaurwlb\nzbqzykdfeunfcwslv[fnqtxugkwojhjjqg]vetgfnapdhvbdaiya\nuxpnaesrcrudsmuxvk[zmffkqaufmoxgoelq]jldwuldydprcfgod\nlcaqgsbmhyfmfszya[brvxpxjvmtrdkdmfm]cphjfsilvnsdqmpxob\ncwxycngzriigcet[xltlzayrmdowajvins]rbfmarruugyqhvegod[nbyobbfqprdigngp]nkrwqcyinzutnklqb[ajhqjuhqzahxzjbk]nfyrxcupuphkbxjqlai\nxqwbcunarmghbsosq[jrmjtqqlogscgojnldm]bnzhiagvdwgwhuawz[toxpipinabgmkbwhtd]uxpgoorspsohkmd[dtadhrgzvfownrufn]xslrmvbosoeoeaewnfr\nlllhkodepygrzesxp[zeohwydmclhucevd]hbnsvtijajahmkclbei[byxhckkvqixiwtg]ekezugmyyavcwxtilwt\njtjbuoavqyjhlaw[vbjakzkppzloxxfx]vibdluddkdsdexqnwl[ofqpidngtagumrk]kfoqunkkvyoassxlgg[ngbosgdywnmslnszsa]hxpciqkkafpdgfki\nnenfymvefbgzvag[wiqscyftlldcvsnp]pchooarrvfpzhwvcjpl[wtitvzxuvfufwviff]opjkauasyyfyspzoufc[pelszbarccpqtxvawi]cmkfptidaetuqkwz\nhitjejomylbutupmkeu[qdzbydybpabfnlkwkv]bdlbevsgqmwnbolnhfi[qeujppfhpzjbtafrgl]zvirtzxdzoojcwfohx[ftgmwthtcanqrxzks]bsafidxuxypaueoxg\ngclocruwassudla[imoknvpznyxchnrvl]qgninncvnnwjovnm[jwqccerrryoiwsqf]chcucyiszjrnobxal\nwqlihvvkfdyrhbqu[vizkatngyvpxuwhsfr]mrxbfaovpijyrmtjxw[mrkexdpmoaarqfj]kmnbalnjnbjcsdulczi[rkidvuivyaequway]jmyicruofboygakaozg\ndvyalwumbdjeaocae[zonftyvegiqiquqac]osgmsdmqoclweiqi[xhgqrjylvorhpfkh]mmpkmrsideufseuyaj[ogtngcelyserepmqi]kjezmzobtremfefqz\newovyikmmawzzrf[hcnunsbuuzhvduvyo]pdkiewvktjzzpqwvpdw\npwfklqtvnpsajdvtyoz[gntgytituioaybkpjqv]wteojggsgedrjqdi[xzvkngdojribistpis]xftjryqatcesygfzoa[zddmnkhceqxmznq]bssablulgiiovynaqrh\nztqjirnmogqbcfifh[vyeztcrzfxnegdyeed]redtifioqpfzykudrih\nosawcjcmfchcpgyi[ffwhlengegnjvwqehkm]rvtkttwkeoefydz[cokaihziodpeurmbp]spjznidsrkpqhsoag[mautcyrrmxsnrlw]dastqkwpjbubonqagfx\njctsgqoqjqtodkhvvuu[ylovawrcpwpnzkfp]xtjdibtsmpbidvvdh[mmaecjrzneokajhkzc]wbwaapxadknspjujtp\nizxxelepmvtrpcb[xwoxroumisiqgpqr]lvhyjhchdicledub\nlqvelunldllnngme[lomutagiggypbbw]hdubyftczrctokdhvbl[ymxlvpbfiojaausmi]uqvhoaigwswemktiu[iipvkifnptbwuax]nidlqwimfttkbnmms\nsewpymbrjgtmkqd[tldvdouashkzpbu]qjujogijyyqwbvzqe[xmhewesgbeyrqkbfj]heapyhfvnqovmlkz[sdffbynjptvodwocru]lwqkbkjseujzmqprv\noegfarvdcswdpnss[xgbroqaseklyoxl]wticmsitljjhgos\nbfhlklvvprpfgxt[wczpqxciyyulsgf]fhlzqdaxyerlulakhbi[xgklnelwoygvyged]ynhbzkafydsmevse[dfcrqsfpouuvsycxi]otcdmymmlomedultqa\npvyddrxqxuxvzfqfl[nipfbquzzbmecwuu]pxzmehysojqnpna\nvthwugdifklqusu[fmffwynjxyagyycbup]eaompujnjzaowbxmg\ndjekvgwpzkgwzwardaq[sjycmrggjjtzpzoq]zgagtgosiowypvz\nbicemnivninwfubpi[enghcgyjwfuwqvfcrh]crycaojgzeqgyxdq[zxgbztjljhdhzpoy]ygxqydxramuikbawdoz\nwdigyfqqrkjeseda[yjezqvkmaqfkcxgu]dwpaveednjywzth\nvjeaiuwrhweqviyv[twssdwyckfswwqg]bujjzsuffbcddcqd\nouivgjbmmsmiezanss[mltubwnsjkijprjae]dxjbngvqbuzmtnxj[actzjkmbxwewlhmpz]aeweucknsntthwwvkmk\nhqxgwpeaugpibuu[ftohsergcnnghmultwv]oobxyesnifpglsyumqx[wthgkfckhzdlzeh]tbvnqcewxwzutlf[dbsokgifbtstadxjlyv]hcagowbeupbbxvnnudp\nfpgthpsgglztrnrjvs[rznddjrlsjtdrnufotn]nfoxdbhyvovsaratt\nidauaxxyrjljwtqk[jtrvbiyczhqigjxfam]bsmzdrpeytyegsvitk\npoxzegvwjgitaomcy[eatpylidmcjifnbyt]pxsatbkkqdylippyjd[nuwjwmoghmaptwgm]tarinkguhfewrxedty\nwhrppysnyuopewxlch[tqeujwwbfviqker]qvintkkgeyiysbl[zmhfxkhgptetdsq]jazfxamrhsjvlcwr[ybdhlaudcktfgpjajk]vnedwkbznnxoegxe\nwmgrbjddretekijeqaq[wxoqrjnhathlpva]nqrxdfrjrvsaxzgn[voeyknzetkswzmonnh]qexvtsdihbxdwzeympo[mplyvliqtgoezpr]bsjrjqbvgcrxwnpdqs\ntxicytmsosvlzftbikp[hwjajoqvcmhmitvqnh]gndimhsqdssjugsp\nscuaijeujwpdvdlzf[byroacgumqpoawl]lofgfiiquoftdrrxnhb[vowfcxvalicqrtpvkga]vdehstpbvncodihewhv[tqrtdbglbqthqfjyu]loycwsbaxhkfanhnp\nqgexpbjlhcciuhouo[apvfnzznkuufvlo]njoupqjamycblyd[tbviqvflseyhhsmxz]lvpemusmcuajelt\njvrllpusmfmsnwy[yqlfrmtxpvwcllrfev]hpuqtteqblrjbnkx[puadngfdbecfuhuvrqb]myxzjgttaacbhzlpipf[gcjfzcrweoksbywfdc]mnchtfuqvmltrxakz\nywmkwcztiqykpmju[zmkryfneelvtwfnm]zhuiojbicjnfdmsdhi\njhgrwzznkirrskfzfbl[ftjkmxrdyljxzov]wcszeohqiseprjde[ngrtygnnwfandfuvr]lqcatjwzlsbuqnzyhw[hdhijvlmfotjdaaivaf]glgrbynrgpcxjihg\nujtcxpupjndfftyfay[wzspgaqtsinvgbd]oskncvkxhimahafzkp[tbtuibverwndjkyrbtb]vubbwzxvzotdhtvvx\ndgjxjkogwuxxgavcit[shbqapwgyduxmjdzs]sqmxfuntsqibnshlszq\nbyysjubuacsviouubxd[idvdypsyblnsmvvv]llcmcxizvdvtmksphjf\nbfphxfyrcoddphmhwh[xvbfcujmhltkfiqaejg]wxxbzpwusjrylub[vcxoevvppeirkcl]bmsyjsnoixvozodjpm\namhqkszrkzcvumwjbr[wgobbxkqavcfedi]blkqusznjzozcwyatzt\nchzanckbvfhvxoikx[jeyndyycqesiujnj]midrrqwphhqptlbgy[dcelctfpcmitlbrdu]wmrripumgjowiedxpcu\nrbpkmcggsbshhytszrb[rjftwgbycnmyxxockku]nrtwwneopxuypblr[hovauqqiboxesfrqqfx]ytyygtytusfdjwco\nytuvowkwojtdqfjtmj[ssrmnlgjawuaqqrdpv]ugahrlchntdmkwkygr[ojlgerllesmyzdbnvc]zaztsxmsddgciyz[jdimgvtyvojseeavk]qvyupywbpmhgoppfwru\neirfjumdodlaevcsigl[befivodoxdnhfmqwkxc]qjaeppumixfpezjf\nlqkzkupjsinhxws[oibgvhxxpewuebro]qbweuxvitezbungy[lapasshrjxcjgdooj]hmxejqpigbcprqregtu[pqqqhbjetacltithm]zhectfbzhtyyvkyazu\nihfadsstuwooioj[dfqkggnfiplpdcsnmx]ylmhqzhlwtxaxhx[yyqzppjaxhmgnlll]orngviyezsyopwfxmhu[pucykxnzcwdwnjzruf]axfmqcflmrxdldubnca\nrsaoluhtqbbhahhk[ursokfyrzqvmjsq]xlniovtwozkeahaydy[nyualslnfurebmbnv]ehgueldltahorrpbbyr\nlviuzeeixehupjezj[gzwzktpbujzeyypbqyi]ecapnyxygcmgfhgmfav[qclblpzrkfredwm]wcdfuzpoxtmzkif[okgiecyymbnmziyyke]zflgxeqtxzeezvc\nwzpeboftsvuwnxel[hmqswpadnffutphylpg]hbapzwwtxulrfaenb[hgsimoxqivllbthuavr]jpxhxohhxhlhlfemuz\nxbojluzthxlygkyzkwr[hjnkqiofmyuospv]gaglxxtcdnnbfvjubea\nuxtugntiubziynpzbju[onxffxfoxibzzzd]wineojjetzitpemflx[jlncrpyrujpoxluwyc]fxvfnhyqsiwndzoh[lkwwatmiesspwcqulnc]cbimtxmazbbzlvjf\nbezefpkmcyawtdlbnmy[yxmpaexxuojocuutf]gybqtynhfakfryzyoot[rzddrwizmjilbaevypd]wjfzotxmdlvmjcklea\npsehcauaffyyegx[pwkfxlhukfaavgq]pprwkzrtyyghtmsciep[rbobphjpqsmeuvgrjt]vlobomuxuflrqfwjo[nijmtbnuuzplcprb]snfbebpcogbvkwf\ncwflkfoevdvovrmn[xfkkrwrohqcdsdyuomb]ohirkxwgudwyepwtvm[ootlpxttypewmdjq]snhujgngvmxwpmagis[fmbwhgzljomkrdcph]pvfendnvzctahabni\neoczaktxgrdpwordn[rbhnrlgckthgxxuzu]htgvsgazuzqpkjoejg\nwwadqndhcahxivixrpr[byzxpjmhnwsplkf]zgwftzdjcyjhuefzynn[pvifqpqbtfpvxmhma]atwcwmmvncdisnmw\ncjbhnctazhwdvcvza[ydnxbdfkufaflga]tyxejwcbirwrznjbf[wmrholfqzuzmywhlx]yuglypghwrwzmduczd\nsucrzntdgccanozz[dbyodxkqvfamarbda]iwcomrnnifahrolyhj[lldsewtcmdwovjto]kxnjfljadgqmjmmr[jpceairekkatfdo]loulprskwdwpwupvlow\nrmkxvrnxpnlpgxk[ymfqtqhsulsvevgy]mwlnvrwgovdeimq\ncjytdtwgtpfaoqpo[ekwzzukvazymdgcjbax]qmhoxsmtmokxfyggfsl[ghoubcwbxpcflxaoiqr]mhzvuhnaesfygwphehq\nfjfuuxzzuifgatypkx[pqxsrnqgcfmmojf]drmywevzjvfsdwoe\naaltjjojczwavnn[wsduayllqabakudvkzo]lnkpzrwwahybafhnmlt\ntrzcoixqxcnlfmu[kxdaqkezsbtcrsel]aimhkjueidtzheak\nknsjvqpezxmhuhawprd[zfschikoyuarwrpvh]jnwcjfkahqerhof[eiezpktdgiogoghnyq]xumsccawinipdfbk\nqdxlgihyxpurnyesn[uoqazfufeeorudagpbq]doynfpdydwxymmbnh\nhhxsolxzfchrnjue[qibcadmwrkmkbeye]xydgasalivcqoag[oyblkffxdgogkbjkk]denthwhcbyimeeyyb\noomceudfrpdpinwaw[umnoeimbzecoaprmqr]vnswrzldpdlfoaaaxv[ysmxmvvxuzozxtkar]eatvxgtbqcoquhhzzn\nmrgnhaqqyhhvdfoo[brbrzbaajkxnrbkpsx]qknvrvpfabkczng\nxtvcrctmszksrojch[bqfzfdhhsfkolghur]dwqpjaqisitqmhpnkxb[omfmirdtvkdoehc]dgogacudqnrtshre[nudirbvfeacxjhb]igdfrdrqycnowffn\nvrgmsmohxhgyybr[shaciuypkvkjaqoho]dlwfavdhohiruaef[iowdifdsyckgfaixzbi]rbkuyahekeohyxnyxmo\ngiaemyheoijyiqs[dditjewdytotrevtph]nrcosaxnrsfnglxyrbh\naqpquczuuqsqfmiynf[rytylbwxvhzymqtqal]olufblbfhnqfhbdpjc[njyewyvnezayxeqkooz]yawvjaofjaqcpsaqnlj\nynntsleqhquylfosn[esbohqcciuuyintjnn]krtinqbvgjtfvdttys[cahezzmqcfayrtijrl]jlquffpwepfjhij[gsryvmkutwbfvekc]xwuhwthwkpiprtpn\nwcifpmwramdtgbyx[mnetsyvjbkzlemkkrj]ghtuuasxyhlhdiqi[oidnivyrbzficmrkxa]sshjteaabilnbbv\njpzlvsyhfjewjsp[zaukqnrnkxuyblu]itarroefggdtpkwknhm\nnxdmkipobgdhcekuk[edajmdcmxhcxntroa]vgrzzrytukuxdetf\nelfvvedwjbltwcnsbat[wlyogdvixiwmkxvshnm]cwhhqukydgvfwzkw[hendekbuynbsgeza]unurlefaaduvvpbi[uriiixudeogykwckty]tilfmprasfargwjoeaz\nehllosfwjnemfpzkjbh[paefpdhywomalbjjwco]jynaehuopnolwbg[cusfqbvxlvqtqbuxgyg]dnvunkjnzqnxcginfx\njfdeexfzxrfxleh[xqkthmkzmmfbesrfa]ddwxrlspxpefvpkhiz\nfpexyleujiphzrejgu[rjjuimrbnfxihopoasz]xiovbrwkxkchdagu[rssesjbgdfwwomrpdxi]xurzdbytoxjkwyzl\nwtudecnnxchnjhuz[ntnjpmwnwqpqqkcevi]xibzynwnkahwfizkxni\nhxvhhsyrupdpvjymv[jgionvwaxuiemcdtvn]riesyfkfymxxite\nndpfqkkiqgvdiciv[qwegblwhxefkszrc]ddticzcfwxoylaheuam[kyqomblpykgrsofpbz]woykqlgorinilldl\nlupajnaqxzgawmnb[zfmybtxebhkalxwfwyt]sknfwfxgdqpbnqebbt\nqkttfgfwmqxgpbcgqvg[zkftxwwbappqdllajhi]ducnsepawowmjggv[osygsyvnhlhkrzahzoa]iygudcaycsrtbkohbrd\nakdvrmxjbjaahjcfhz[nueiutbritxbampij]vjirxewhgmmwlora[uauyvvwvrfhbxituz]omfdcitqhjhentxgfu[fucgdtoxvryasxib]wyvdxqpofoszluslht\neorazrawyakawjfxdtw[bpyrfrsjhfualcoyfjc]gfgrienuzeifrfvw\nmcfhxjmwxlcreeloqkj[xlhrkjackiehnqj]iubxmjyssnwjolapvs[tnxnpotyzdxhqamjfu]qakefkzqtcahednybux[tosvyefshtbgasbf]uimrnuvlevqylbpkq\nemyfqgrtebopsxa[qwacgpmlcpoitzmdq]weqwomfyfqhxmkjalw\ndgnbvzkwdnxzuduvdee[palmkulrnlnjdyeavyi]cjgsjpbxpairrderw[nnoxigqxpkjzjhfxgxx]xdyxrtslnpmmtpotla[undscmvmhuxzohsdg]ghxcwnjphcmvttna\nuppsitifhxdcjbn[yiqjsnlktwkbfyho]dpftntebjwcyuih[rrqikyarnxteelpkc]qbjeplbraadbjxoicjn\nmqjlmaekarsttdmnl[cwdajzaopmbrikcv]vfhztmfwqcwsbdnyebk[puetgqkczejvdjbfqc]hdkqfycmizzpuoxumm\nmaldhmhtlcsjqyzrb[zjbfpjpvdszrqkpzf]xspijlrjyzjputpz[mcjmewdtmgfqutbah]hebhshxtiedpjpjngu\nhiqikcyyvddlcggnq[ehsopbptguatpmyb]wfayjslqiqivsbrhedh\nzriahyyoezygvjmepy[dujudufydhkqlbc]ndalzjrjswnjujfm\nsilotorivixpdydnd[wtsojgrfgugwoyo]pfihyfhusblbdodtej[hfclibenimixyexhble]gaglopphfrhqxikvw\nddejnfspvmvffpfyozn[odqqmwgalivbswfio]rbbkjhvnszgvfjtgog[fgvufpphptnjcmraha]adsajvzndnajmilk[ukslffqfzyvxyxy]njzcfhdqyrzzctmnxn\nehdmevcrfoeejfedbnz[cidowzljgyawbjmtzun]mxyjuechgccpwlxj[ynbdkyqvibsfwekcjr]qjilshucvucbebxmeyu\nwfyklfdesrxsopcnj[otmmdkdasnvomdhef]lpbexhubcjmfwlt[maeuvtcgzoxemnreol]qbwqszxalocdbfbtge[wbvswinrpyzjbfrsr]tinsrsxtrfkizkeu\ngrorjgszsijwlhxfrjv[hmjhqmbipfjguwkzebl]kgphtaonflqlgbyk[qxnjzdupbhhsevc]tyflwvcpxchibnttwsn[ukpfpknbyacpxmoxzmp]dxzkerytewihuptx\ncsyjgthhgyhnjuxxg[sjqffhahrjyoqxncjcj]owwprabojlpraeyk\nibcaffhxenjnmvrnog[shqpfncawueqmpyj]hawlfakyplonsim\nftaeqqsyebdeveutf[tnifrefjkddtblslzwd]cbdooorsorxwxugrp\nioigxerknwyrzoztkv[ffkgwjfeowgtoxnyt]zhkhaqrcdjsvxctdj[ebntbwbxzbbqrdasjz]solgzrowmzozovz\njfmlobddfxzipyzyaj[qghvghaxzmuhrpifyf]idrqkcfvatwsyom[wncyawwmennmgio]luzaexvwjhxbryah\npjcydgylusqdexbb[nsoyssffvolztzns]mntwrdacovyfxcqfn\ntagdiyuylrtvuyu[exjzdpmovyftjpxgj]vnswkkhaoldjfkwd\natowdglgkmbnrvyt[uzgadzquqpggiapdznk]snpqanyoeufutazn\nnltynylwgqezegky[rawbwledrpbduldc]isupsldtvjtahlwjgz[upmovvichcymgwuoqrc]gyjptxtuaqcfixjuanz[cxzbiosnqkeaxlkrxh]yglfdtzazlkxgmrlel\nezensxwulgqdgytdfo[ozlmpzteuyjqrxocn]crruxzecnvrcpjurn\nycflwfbhueatnpimmkm[tbcsifgtkkwtxosxau]vsnyspuvhhfozxgjbbp[adcyzxtdknieifc]hjkfmbmxkrnksewsqjn\ngffllhgsmlpxkktcq[wjqwhqrwepermblfolw]wzgcjyrpisbwyhnz[yjvzaqjsmdgazjuep]gregropoulmnagcvx[gfjkkejnxmpfbtecy]ufbqwnifaugffsai\nxfrmlrlrhxsownybek[ryhsyltyflhjbmltndc]agtvigglsugquzbc\nrshzvotgovlabfxr[sbuytwdobnvpwcax]bynmysulnnjmhkf\ncevbpuyyvlutjcuutl[pfwloktlqbxfcogrc]dflejqcyvpasjowhsj[nscuwnjsrzehqamogtw]scemydqevrcuvhwxpe\nnsbvubuyjrzsalkdwz[fooatkopdyvkxjgfho]jwojdgxqtlzxgna[vmkwusptfjbgmhq]xkzpfgkklnxunma\njovdewpqyfouyzpegwg[eigxaawljopqauy]cjvieeexlyiovsugif[wtkkpylnxtqrepkjei]jrdmibhhcftoeauh\nflpwanunpldmcnated[unzsihvveyitclcf]gqxlznjbnpmiojuunu[kxihijtbrbyhkzosvk]xoxdqctctmroxoppilv[equfcbnltdiwdmahu]sxfloedvbznwctnuqt\nwtktlikeigdndpyw[dspimpajtzfzmfya]rmmuigyferofztnuir\nthnfrvngjhjrwdatdc[vwmnddbpbakuapirel]qojpomziuupsfysyfng[gkgjyjoovotmjwwgvrq]xxfsycfupudisdbtk[hnieklknhbwcfka]qbanhtkdijnnfegs\nmazcgrfwolhhbtman[jokgcthhpopluovccrg]eybriinzdwjyfjes\nkwxxubruqgrsifrpuxe[pqjcuxzpykriher]rcjvrturrhxqhjndj[umqwgmhgidzakfnk]nzbbrgxxsmkxahvqzs[rnqcmdjyrldnzrr]nhztvrovbpifyxbcvti\nkgojbczgybkjpoz[nyemqsvkokdfxiata]lrstpiuovispfmuoi[jifgmwihkzirfnblzqu]dixnvdkqejtatylghtd\nowhhzrmvmuosrtiwaf[xvdujvnkkrunymvh]dihbvchdelxcqsmlxe\natcmrejivvyxxbsexp[cjlvkmfgfjslzeno]liavdjycjpirlux\nsnvgwihgkhrsgdzysbh[bbyzthwnbpquvtrmlc]cdwvzdogbisfoopk\nlccrydahkgmzirmjzfv[rkkdtcqmlfkxmke]xkercumbulkzrlgxng[deksxliclevazssc]yhidzcmnbvgacmdv[ucxflzawmxnmpxa]hrfaesdlnukcblbqlm\njdajqnzqyhcomekhejp[tyrtsgspmlmrbkm]nyfcgbagjplztrigokr[ntzzerjwsgafymxw]ftckmtirxfdfcqpi[pulepgarnqxbvlqmvog]qashqfzwglljzexbnsv\nkjvalulqegxybfhx[djfulullrbsebeknl]bcxpgathyauumxcrsmk\nfihxcyovovcmukir[gucbridfutpdnto]abzjiaponkgoposvhw[vpqwcnzmovnwdwwo]zrkqlpnszeioesnhk\nnyvobmkhkbenucug[dwpifbppiwftzokarg]vxxalauqmooacfmdox[intaxgcpfajzdwmcsk]brknzsnhuukxjuv[fkheyxevpuphuflvzkk]levqirhqhynkthsef\nuwdcywcarjujlnh[qvtowczbkenlghcmara]kfhcbnrkorcoyhkww[mzzwrpwwkrnnfavjxk]hcjjzxeynegdpfwdw\nxtgkbqtzbeptcxndjxl[jzmbcxsmcrtjtqi]wnhqmctldgxjbrtio[brnnosnckhalqzqsyyv]uhungebnygpsmpzmj\nxrqpqqsqazzlqcdglgf[ziiwwokpqiinmqe]stagyposntgyxnh[ubxzaskwfzlfrmw]fimsoerydnghxlg\nbdqtpixvllcdhgfqby[xurgfxznrblksso]wgfyjdmpjqirhiqvgg[pbgnckfbdinlepkb]mqbqboepuqheaop\nxxlhstlmqypoyhb[czlhqkifhucxqanafx]jkaaxiwxrnneudczrtn\njhcmhtveqenmeczz[rcpnnuwvwiyfjxo]bvtashqfjcnbrqy[ebgihcdcimvgdwochq]pmallgnuofajusz\nltzknsdqzdmbpxipt[golssizcvkrcmquotrj]nqjkcgdagjqzvri[xzehrntfgcnmgrh]devpsfftuonmevocw\nwgklxpmeoznyxtukh[nevjkmpvlbaulxjieh]wopqaknwlwjquxt[mxzczmngcaxharjipt]tuvwngrmylububv[ryewaqhshtogggdvc]xpkbqydbwshscjcw\nuglrhqngbxqtqmdlyym[ihdwlwfqiwnigvyarcw]miyynkctggbwzfkq[rqycaudamvwoxju]mmnzentjyyddntnpgxf[qjryduwnivawjepknli]toodveiqtzjxjvq\ntkgmnxgifkqzuut[csyogdborjrnygg]rpcbucosajyyyelju[bbujqtlveymlqesvg]wvyfimibeynzhsotymx[tqxldisulrhuckef]kgqjgtaluastnwev\nqifwiunabpnzezlmhh[ffwsncvlqpulttkx]wlwdpgntblnoubom[fksogvukjlzupwetlef]cfszpnemoifasqw[ttmonrrbhknspuqx]htucxamhxsoigvt\nputioshxpafnkcwdejm[dellcuoevwyyhvwurpv]zezpevhlmpzbevln[rigyoryyhoxwlbg]zkdzexpizgsumkuiuy[hycpaavxiqnlngrc]gknnfredhsmpofldn\neknxasjdtsksamfc[dhtgifeezlgfhlyvfdz]xfttcwzqucrtngdpcmf\nuyiazdptoxzxbzo[bmuglholukatdbf]ascjhcllcatoapyvn[isqfrvbbkzsxixjuqrq]ncwzqqgudgwrtxvzfe[spqvftdlddlfglgg]zrqbukmufumytpc\nczefxpifdsqjjkoxgj[klwshjzagbrgtpiht]xofokkhzlnjplefofcj[xodekgjbgraikdley]dgsrqzqxjxjqftn\nertbujoaanuvqskr[hsgeexqdgsqfkiunhpa]orgvxylmsdlzeyjzf[mdkgzwdnvtyoogulx]nbapgjckrfxeniiqotx\nwgywdqnvxooqjsefac[qgpmwggewotnmloq]bqdvbzpvqwadroh[bvbsnhmdurzcubvsno]ndwqyjenerqdupuob\npatbwuitsfeqvswby[htsntyfmofqldcbwgv]zolnndvkaimzdmevb[feyvwvkelmujnppg]tjajsdtevgjukkgrwr\nhoznvyznwitnxlvu[kigfxgwcrdmfwgsqnf]lhiqoaqezmswakdcd[gxmjrmvoxkdfmgcpqnn]ditkwvolcazfuxzfroy[qqlbrrwfedrgtrgm]iysjaakrbnqicefqxsr\nufrkrtywkhfhfah[vufpfwhtxzbdqnraz]kklboeggazttzui\ntplrraxhaaaoczdpg[vzbnososnioajien]dvdckrkfdetoofpi[bywkgphzoglisygthku]gxtnstjmffnepin[evccrlnwjthfxhhqzc]lisguwkfwswblzc\nlyluhnglmfippljtwww[wnkwnwwsasqbrnlo]nilnannzjbpgbjs\niknqwrvlcztavivxmh[vtfyhjzauqbyjchjt]zxmasnczpxlusknrmtf[yvfnxlrwgfxkdlj]otlivjvbvilezalha\nxbrzzccetyjzrlt[buwwhcatpcchdvhel]wosdwuuzpekifdhhvpy[twwoaezcowxvioqsrrd]uuygkhojhlcofza\nwqeintsbeqzjpuvx[wqlcamjmpbtqqzjcy]czhyqcurqkfnnkoltja[lozjcddygpevnxebmqd]avwqdpfxcrcvmalaczo\naecvebozlythtcfzt[uisdkrrjeboxpuclbg]sjxcgygpeuirukx[zeoyaxgdyzfkprewiyc]rdlnzpbwgztivpdon[sfcqbpfgffkchksmfjp]yfgrlxiixyurxupuoij\nvnglyokdpxlgphpw[bjnaqkjojazyryswr]bekdduuwrqabarzwzh\nfcggyliuipcvnimphib[adkvjaembjcqbcc]envpiocijefswhv\npgraswoweceiftu[khhpmbjghxgmhsud]axqjkekmecwunefk[pvelpeorryjcstk]lruensapttjtyxnr\njomdrazkwryxuyc[qolcqhwdidalguboza]fcofbrgowezhbyqckrw[wurpvelnhdewfoita]swxwyfynaymvrhleuj[icdlergnbqmowlxjl]vxcwgvrvpdejoybt\naxbedlkxkmbvwacv[uabrmhoepcgtsdmjjzy]iqqpitszpejeeophjmv\ngmltcuvpeuofwteput[eyxdpnceufobjelir]hvajyjjzgkyrtgvrfs\nsfyyzksaymsvykmr[xjewfmfhhbrmwzf]cbzjmltnzvcodwtytbz[ewgckbdvfnkkyxyj]dfcrjyoakdyggbsxm\nwxjalqmicwmwkzakcy[mothnmmvgypeacecvz]hbjasxlsbbgxpfdptk\nqtsgwqpihqjgmjadkjz[skpdhegagxxbmayy]eaojrccgpxovqpi[ixyljrfgswullqnbzdz]etvomvkwpzpxxcj\nmbnifyngahvfhtfhql[azcbyxkvcnoatuo]scgddcntikvavaseu\nuciiofzqjkhndnzx[hoyxdxfahorycpfcofk]epeazzccheaegyobu[sculkaizijfqcrpjl]nrvfdtpvgoqioomvmv[axmvmzytxnbfcsjf]fccriiwmdaveeyamwp\nsxizvuhprsyyxgfqgqx[zwszjxransryibshzw]ikquiagnkoqexlsqypb[zpuqrhaqvkuvhiqk]pvuqiqxpjtsyqgcyr\nsvjudmyxlshxbbvawl[inswkufalzfwoumcv]hrobewddabqsiuej[ulhptknpxcwqxjxanjd]osfyeygptwfjmvrma[pnuynwtwuulsizw]srhurplerqabvouelhn\nislwmbcjeljkceppiw[whvcrbqzgtcfbcuv]tcyzkgyzdaekgnzzmz[ddefwmnklcddlhow]npzbtwmzmhjtzljnr\nlgdjrkugqewlqxvn[wtvrzflzauwcxkyp]qbswluceqlesdfwy[kbtmzcvoubbiqfc]honrvxwcqsgphvkt[djuuancygxacmka]knseftjiunzuxdi\nmiapzpluxnmdfvi[edlbwflzitzghywio]vizzhfxgilwpwhr[ochurvodstmhiypp]rycvogpcnysngytixb[mqnrhpbvojfefcicx]zxqxoinunlkjvetkvrv\nspsecopdywuheqbnm[npwovcwlwooxqhyp]hkuizzsdvysvhvmlc\noqchahhsrywoeteaeg[ucowjiwrzkfhyebbco]efxdrribepcvduwjgf[nvyogembujkkmcm]kmfrlcaeawrvofxrim[izjebqewubrbvguzk]ngmugyprdvrbqskn\nvwlikshqcpgxqvqshv[izqveivxdxgytqgdk]abnvmprwbvwmrwlkkp[iffpegqsxjwfyvixtwk]iseiapjkgnkcepr[gtfhysdedzxwrhcgt]ktaeihyqegeozdfuz\naieqqwhwfwxpldni[huyxdcvpglqqkeyeia]teztoyeycqohfli[uqvfjzbsvttphqxsy]afsxoqbqvtxtgriuzjm[psumrbbtxdxlwpk]qwpuwevhjellemzp\nsurpbndlvplunisu[alnojwsmgbtaomke]zjyikoebzazpwql[lkgsnxodocsrniokroa]mrcipdncevvazafvkb\ndkszjaqhbkyxwvwj[wykmzcvppharrax]pvrqzqhabqtuhrj[qfxnormttaxsldn]kxjwkrjwvbiutgnfnw[mbspfflblosguqzt]nifozavfsfkngds\nuwafdvptgkfikprb[xhmrwxqxnbkfpdz]efhnfwvovbvglrrt\nkozevksryerpsrgmub[dbtinyialvlkgilue]pyqdyodlttsnrsmfvca\nmgfmdcxibcgzhrfmm[mzvyabccrdzlaiij]arnetejwseofkwqvxi[fylixbrjhxdfhiewbnb]wvndnswxdnbcktp[tetomqdkfmcndddruy]biuxgrvctlbbrqmxjp\nsnjnfgbtgpkouxlpd[vapbqurlxyrduxqy]meyhgdsbvkdadsfozf\nfgknedldithvaoxqpl[mihhhdrtpjmoridqamt]vfupazymsipoana[ngqkziyavxkyukp]qqysmfkyaxbuytr\nfugbgojgdeavlmrut[zpukymkjkapibmhg]mmdesmcwbhlfugkdiz\nlhhhlyioiiknkray[omilmxkodlmvzhkgbaf]cyftkgjpvjvdnortlj[ifljdtkgscmnmxsq]nxtettqnuaotfsh\nwhayrxopbtvnpobokn[jfbobalkbfjxcsn]jjucgwedwbcfrdginaf[atdoatealbqhiks]alzapbxuvmivqfgpg[qhzdwsbvcbtlpchem]pxxskedydgisthkatn\nxzreuonsdqobzpxr[zamxighfvnaxqum]olbigclentyvugtuvg[ysrgcksohtkvcqmksqr]gnaqqezdmnfbbnir\ngmmabzkwsehkwjnevvd[uuzdntitdazeykwek]aebpajrwpyknqgx[kczhcuveeawmdiwljzl]ugwigmilwkczrcqnfo[piezzmfwnfdhnlbranp]qhremthdwdegacvptfe\ntcqhlxasqmbwzuiuirp[kfqoequocdsfwqt]ikhdkpkmeezfzfyyilf[lrorfowgsqkflwauhu]zshoiccvfwohudsmdcr[zohspdmqcdvgagdknr]zabaqgsmrwkrtcuyct\nfzanofpykognmio[ladtxyissyfrssobo]xqpwrgdmglgqhwawqok\nhynipihszohrqwaezga[iqtpgjpngbwhpailzg]wfgimkpjrjnkroueh\nlpmrkesaqdojkqrp[dcgsayoowgpiwam]arphrffqpcdntlxsza[ogneaqyckrvdcvqxbm]xlogrojsovrzfzjtjbd[qjoiyyatxkwsrvldp]gffgmieinxlfzpiej\njaeayfunulncspts[stghconfjhkqkrxncwi]kcnaqhyukuirsaeebp[vynwfnoxxxbqztj]gddvegwjuryfnkgkpqq[jnhmbdpvsxreqhoek]pgpikslhvbnmbxbkbc\nlajiqiaxcxgpvsbu[bfetstragmoosbw]hzurjpxhecnadwosn[dquibbrojgurqiqd]aceccsnyrnfmcsd[quqxmzleqvspvsemjpn]noxrndgdrkffsdvh\nbytcvwxuavajevmde[nhmjatzolmbdfgogup]qpildujniqlnfbmuf[gxpgorlbxpqfsoreuey]hcfyjmkoywueuivrio\namvudustnspjqsbpjp[wdudhbvvlgzbbbwlafg]kwpyjvuerzyzmzft\nvwpklmfpzssyoifbb[bwtpxodxedpdsvgu]azathmhdnqkhbmrdlxn\niwzncixpjxypnmykke[wlhvfjbumhmtachoab]wtftbolwhpwnropnzv[zhfcmkbwizknymev]twrumqadwvsaciwbwoi[evodjtvrucrzgtwio]fmmbddkwwpaziycik\ndkodbaotlfdaphwzbcc[ldzeemqiovyqjgs]qxibabdusgaistkru[usglloxgycyynmp]aaocvclsocababbzxeg[liaacgfxytuqudp]jvvqsypuoduyhvraak\nbwzsacxgqkbjycgfw[dbnligvrmqscasutn]rbgybqqsgjvlonkut" -> [w10]
    tunnel: [w9] -> w1 mode=indexing
    stop <- w8 stop-if-true
    n2 = Match Pattern(string=w10, regular expression="\n") -> (before substring=w9:string, after substring=w7:string)  [unwired: 1 in, 2 out]
    n3 = Equal?(x=w7, y="") -> (x = y?=w8:bool)
  }
  n4 = while {
    tunnel: w1 -> [w29] mode=indexing
    stop <- w27 stop-if-true
    n5 = Equal?(x="" ("y"), y=w29) -> (x = y?=w27:bool)
    n6 = Search and Replace String(replace all?=TRUE ("replace all? (F)"), input string=w29, search string="[" ("regular expression"), replace string="," ("replace string (\"\")")) -> (result string=w31:string, number of replacements=w23:i32)  [unwired: 4 in, 2 out]
    n7 = Search and Replace String(replace all?=TRUE ("replace all? (F)"), input string=w31, search string="]" ("regular expression"), replace string="," ("replace string (\"\")")) -> (result string=w30:string, number of replacements=w24:i32)  [unwired: 4 in, 2 out]
    n8 = Add(x=w23, y=w24) -> (x+y=w26:i32)
    n9 = Increment(x=w26) -> (x+1=w25:i32)
    n10 = for {
      N: w25 -> [_]
      tunnel: [w73] -> w28 mode=indexing
      shift-right: [w72] -> _
      shift-left: w30 -> [w75]
      n11 = Match Pattern(string=w75, regular expression=",") -> (before substring=w73:string, after substring=w72:string)  [unwired: 1 in, 2 out]
    }
    n12 = for {
      N: w25 -> [_]
      tunnel: w28 -> [w82] mode=indexing
      tunnel: [w77] -> w19
      tunnel: [w76] -> w15
      tunnel: [w79] -> w14
      tunnel: [w78] -> w16
      i -> [w84]
      w81 = ""
      n13 = Quotient & Remainder(x=w84, y=2) -> (x-y*floor(x/y)=w80:i32)  [unwired: 1 out]
      n14 = while {
        tunnel: w82 -> [w99]
        shift-right: [w91] -> _
        shift-left: w81 -> [w90]
        shift-right: [w90] -> _
        shift-left: w81 -> [w89]
        shift-right: [w89] -> _
        shift-left: w81 -> [_]
        tunnel: w80 -> [w87]
        tunnel: [w86] -> w77
        tunnel: [w85] -> w76
        i -> [w95]
        stop <- w94 stop-if-true
        n15 = String Subset(string=w99, offset (0)=w95, length (rest)=1 ("length (rest)")) -> (substring=w91:string)
        n16 = Equal?(x=w91, y="") -> (x = y?=w94:bool)
        n17 = Equal?(x=w89, y=w91) -> (x = y?=w96:bool)
        n18 = Not Equal?(x=w90, y=w91) -> (x != y?=w93:bool)
        n19 = Compound Arithmetic op=AND(w96, w93) -> (w92:bool)
        n20 = Concatenate Strings(w89, w90, w91) -> (w88:string)
        n21 = case shown="0, Default" w87 {
          tunnel: w92 -> [w103 w113]
          tunnel: w88 -> [w102 w112]
          tunnel: [w101 w111] -> w86
          tunnel: [w100 w110] -> w85
          frame 0, Default {
            n22 = case shown="False" w103 {
              tunnel: w102 -> [_ w109]
              tunnel: [w105 w107] -> w101
              tunnel: [w104 w106] -> w100
              frame False {
                n23 = local read "Pattern ABA"() -> (w105:string[])
                n24 = local read "Pattern BAB"() -> (w104:string[])
              }
              frame True {
                n25 = local read "Pattern ABA"() -> (w108:string[])
                n26 = Build Array (concatenate)(w109, w108) -> (w107:string[])
                n27 = local read "Pattern BAB"() -> (w106:string[])
                n28 = local write "Pattern ABA"(w107) -> ()
              }
            }
          }
          frame 1 {
            n29 = case shown="False" w113 {
              tunnel: w112 -> [_ w119]
              tunnel: [w115 w117] -> w111
              tunnel: [w114 w116] -> w110
              frame False {
                n30 = local read "Pattern ABA"() -> (w115:string[])
                n31 = local read "Pattern BAB"() -> (w114:string[])
              }
              frame True {
                n32 = local read "Pattern BAB"() -> (w118:string[])
                n33 = local read "Pattern ABA"() -> (w117:string[])
                n34 = Build Array (concatenate)(w119, w118) -> (w116:string[])
                n35 = local write "Pattern BAB"(w116) -> ()
              }
            }
          }
        }
      }
      n36 = Array Size(array=w76) -> (size(s)=w78:i32)
      n37 = Array Size(array=w77) -> (size(s)=w79:i32)
    }
    n38 = Not Equal To 0?(x=w16) -> (x != 0?=w12:bool)
    n39 = Not Equal To 0?(x=w14) -> (x != 0?=w13:bool)
    n40 = And(x=w12, y=w13) -> (x .and. y?=w11:bool)
    n41 = case shown="True" w11 {
      tunnel: w19 -> [_ w45]
      tunnel: [FALSE w44] -> w18
      tunnel: w15 -> [_ w43]
      tunnel: w14 -> [_ w42]
      tunnel: w16 -> [_ w41]
      frame False {
      }
      frame True {
        n42 = while {
          tunnel: w45 -> [w53] mode=indexing
          tunnel: [w48] -> w44
          tunnel: w43 -> [w52]
          tunnel: w42 -> [w46]
          tunnel: w41 -> [w50]
          i -> [w47]
          stop <- w49 stop-if-true
          n43 = while {
            tunnel: w50 -> [w62]
            tunnel: w53 -> [w67]
            tunnel: w52 -> [w65] mode=indexing
            tunnel: [w60] -> w48
            i -> [w63]
            stop <- w66 stop-if-true
            w55 = "" ("x")
            w70 = 1 ("length (rest)")
            w71 = 1 ("length (rest)")
            n44 = String Subset(string=w67, length (rest)=w71) -> (substring=w69:string)  [unwired: 1 in]
            n45 = String Subset(string=w67, offset (0)=w71, length (rest)=w71) -> (substring=w54:string)
            n46 = String Subset(string=w65, offset (0)=w70, length (rest)=w70) -> (substring=w58:string)
            n47 = String Subset(string=w65, length (rest)=w70) -> (substring=w68:string)  [unwired: 1 in]
            n48 = Equal?(x=w62, y=w63) -> (x = y?=w64:bool)
            n49 = Equal?(x=w69, y=w58) -> (x = y?=w61:bool)
            n50 = Equal?(x=w54, y=w68) -> (x = y?=w59:bool)
            n51 = Not Equal?(x=w54, y=w55) -> (x != y?=w56:bool)
            n52 = Not Equal?(x=w55, y=w58) -> (x != y?=w57:bool)
            n53 = Compound Arithmetic op=AND(w61, w59, w56, w57) -> (w60:bool)
            n54 = Or(x=w64, y=w60) -> (x .or. y?=w66:bool)
          }
          n55 = Equal?(x=w46, y=w47) -> (x = y?=w51:bool)
          n56 = Or(x=w48, y=w51) -> (x .or. y?=w49:bool)
        }
      }
    }
    n57 = Boolean To (0,1)(Boolean=w18) -> (0, 1=w22:i16)
    n58 = local read "SLS Support"() -> (w17:i16)
    n59 = Add(x=w22, y=w17) -> (x+y=w39:i16)
    n60 = local write "SLS Support"(w39) -> ()
    "Pattern ABA" <- string[] [] ("Pattern ABA")
    "Pattern BAB" <- string[] [] ("Pattern ABA")
  }
  n61 = while {
    tunnel: w1 -> [w129] mode=indexing
    stop <- w127 stop-if-true
    w120 = FALSE
    n62 = Equal?(x="" ("y"), y=w129) -> (x = y?=w127:bool)
    n63 = Search and Replace String(replace all?=TRUE ("replace all? (F)"), input string=w129, search string="[" ("regular expression"), replace string="," ("replace string (\"\")")) -> (result string=w131:string, number of replacements=w123:i32)  [unwired: 4 in, 2 out]
    n64 = Search and Replace String(replace all?=TRUE ("replace all? (F)"), input string=w131, search string="]" ("regular expression"), replace string="," ("replace string (\"\")")) -> (result string=w130:string, number of replacements=w124:i32)  [unwired: 4 in, 2 out]
    n65 = Add(x=w123, y=w124) -> (x+y=w126:i32)
    n66 = Increment(x=w126) -> (x+1=w125:i32)
    n67 = for {
      N: w125 -> [_]
      tunnel: [w142] -> w128 mode=indexing
      shift-right: [w141] -> _
      shift-left: w130 -> [w144]
      n68 = Match Pattern(string=w144, regular expression=",") -> (before substring=w142:string, after substring=w141:string)  [unwired: 1 in, 2 out]
    }
    n69 = for {
      N: w125 -> [_]
      tunnel: w128 -> [w149] mode=indexing
      shift-right: [w145] -> _
      shift-left: w120 -> [w148]
      shift-right: [w147] -> w121
      shift-left: w120 -> [w146]
      i -> [w152]
      w154 = ""
      n70 = while {
        tunnel: w149 -> [w188]
        shift-right: [w181] -> _
        shift-left: w154 -> [w184]
        shift-right: [w184] -> _
        shift-left: w154 -> [w177]
        shift-right: [w177] -> _
        shift-left: w154 -> [w176]
        shift-right: [w176] -> _
        shift-left: w154 -> [_]
        tunnel: [w179] -> w153
        i -> [w178]
        stop <- w183 stop-if-true
        n71 = String Subset(string=w188, offset (0)=w178, length (rest)=1 ("length (rest)")) -> (substring=w181:string)
        n72 = Equal?(x=w177, y=w184) -> (x = y?=w182:bool)
        n73 = Equal?(x=w181, y="") -> (x = y?=w186:bool)
        n74 = Equal?(x=w176, y=w181) -> (x = y?=w180:bool)
        n75 = Not Equal?(x=w176, y=w177) -> (x != y?=w175:bool)
        n76 = Compound Arithmetic op=AND(w175, w182, w180) -> (w179:bool)
        n77 = Or(x=w179, y=w186) -> (x .or. y?=w183:bool)
      }
      n78 = Quotient & Remainder(x=w152, y=2) -> (x-y*floor(x/y)=w150:i32)  [unwired: 1 out]
      n79 = case shown="1" w150 {
        tunnel: w153 -> [w157 w167]
        tunnel: w148 -> [w158 w166]
        tunnel: [w160 w170] -> w147
        tunnel: w146 -> [w156 w169]
        tunnel: [w159 w168] -> w145
        frame 0, Default {
          n80 = Or(x=w156, y=w157) -> (x .or. y?=w155:bool)
          n81 = case shown="False" w158 {
            selector: w158 -> [w161 w163]
            tunnel: [w162 FALSE] -> w160
            tunnel: w155 -> [w162 _]
            tunnel: [w161 w163] -> w159
            frame False {
            }
            frame True {
            }
          }
        }
        frame 1 {
          n82 = Or(x=w166, y=w167) -> (x .or. y?=w165:bool)
          n83 = case shown="False" w165 {
            selector: w165 -> [w171 w173]
            tunnel: [w172 FALSE] -> w170
            tunnel: w169 -> [w172 _]
            tunnel: [w171 w173] -> w168
            frame False {
            }
            frame True {
            }
          }
        }
      }
    }
    n84 = Boolean To (0,1)(Boolean=w121) -> (0, 1=w122:i16)
    n85 = local read "ATS Support"() -> (w139:i16)
    n86 = Add(x=w122, y=w139) -> (x+y=w140:i16)
    n87 = local write "ATS Support"(w140) -> ()
  }
  "ATS Support" <- i16 0 ("ATS Support")
  "SLS Support" <- i16 0 ("SLS Support")
